vi "Generate NIPKG List from Installed Packages.vi"() -> ()   [LabVIEW 2017]
doc: "GUI tool for selecting NI PKG dependencies from the list of installed NI Packages. Allows selected package list to be exported to a file for use with the SBOM tools."
uses:
  <vilib>/National Instruments/NIPM API (Beta)/_support/package attributes.ctl
  ead8c88d-cf43-4405-a832-7fe61a0fbdd3.vi
  <vilib>/JDP Science/JSONtext/Variant to JSON Text.vi
  <userlib>/_OpenG.lib/array/array.llb/Delete Elements from 1D Array (Variant)__ogtk.vi
  <vilib>/National Instruments/NIPM API (Beta)/NIPM_API.lvlib
panel:
  in  "Export":bool
  in  "System Refresh Button":bool
  in  "System Stop Button":bool
  out "Package Info Progress":dbl(slide) scale=0.0..1.0
  in  "Add":bool
  in  "Remove":bool
  in  "Selected Packages":i32[](listbox)
  out "Current Package":T1={"Package Name"="", "Display name"="", "Version"="", "Display version"="", "Synopsis"="", "Description"="", "Maintainer"="", "Maintainer email address"="", "Category"="", "Homepage"="", "Release notes"="", "Depends"=[], "Recommends"=[], "Suggests"=[], "Conflicts"=[], "Provides"=[], "Replaces"=[], "Supplements"=[], "Enhances"=[], "Product"=FALSE, "User visible"=FALSE, "Installed size (KB)"=0, "Package filesize (bytes)"=0, "Architecture"="", "Agent"="file", "MD5Checksum"=""}
  in  "Installed NI Packages":i32[](listbox)
  # "NI Package Dependency Selector"
  # "Use this tool to generate a list of NI Package dependencies for a Software Bill-of-Materials."
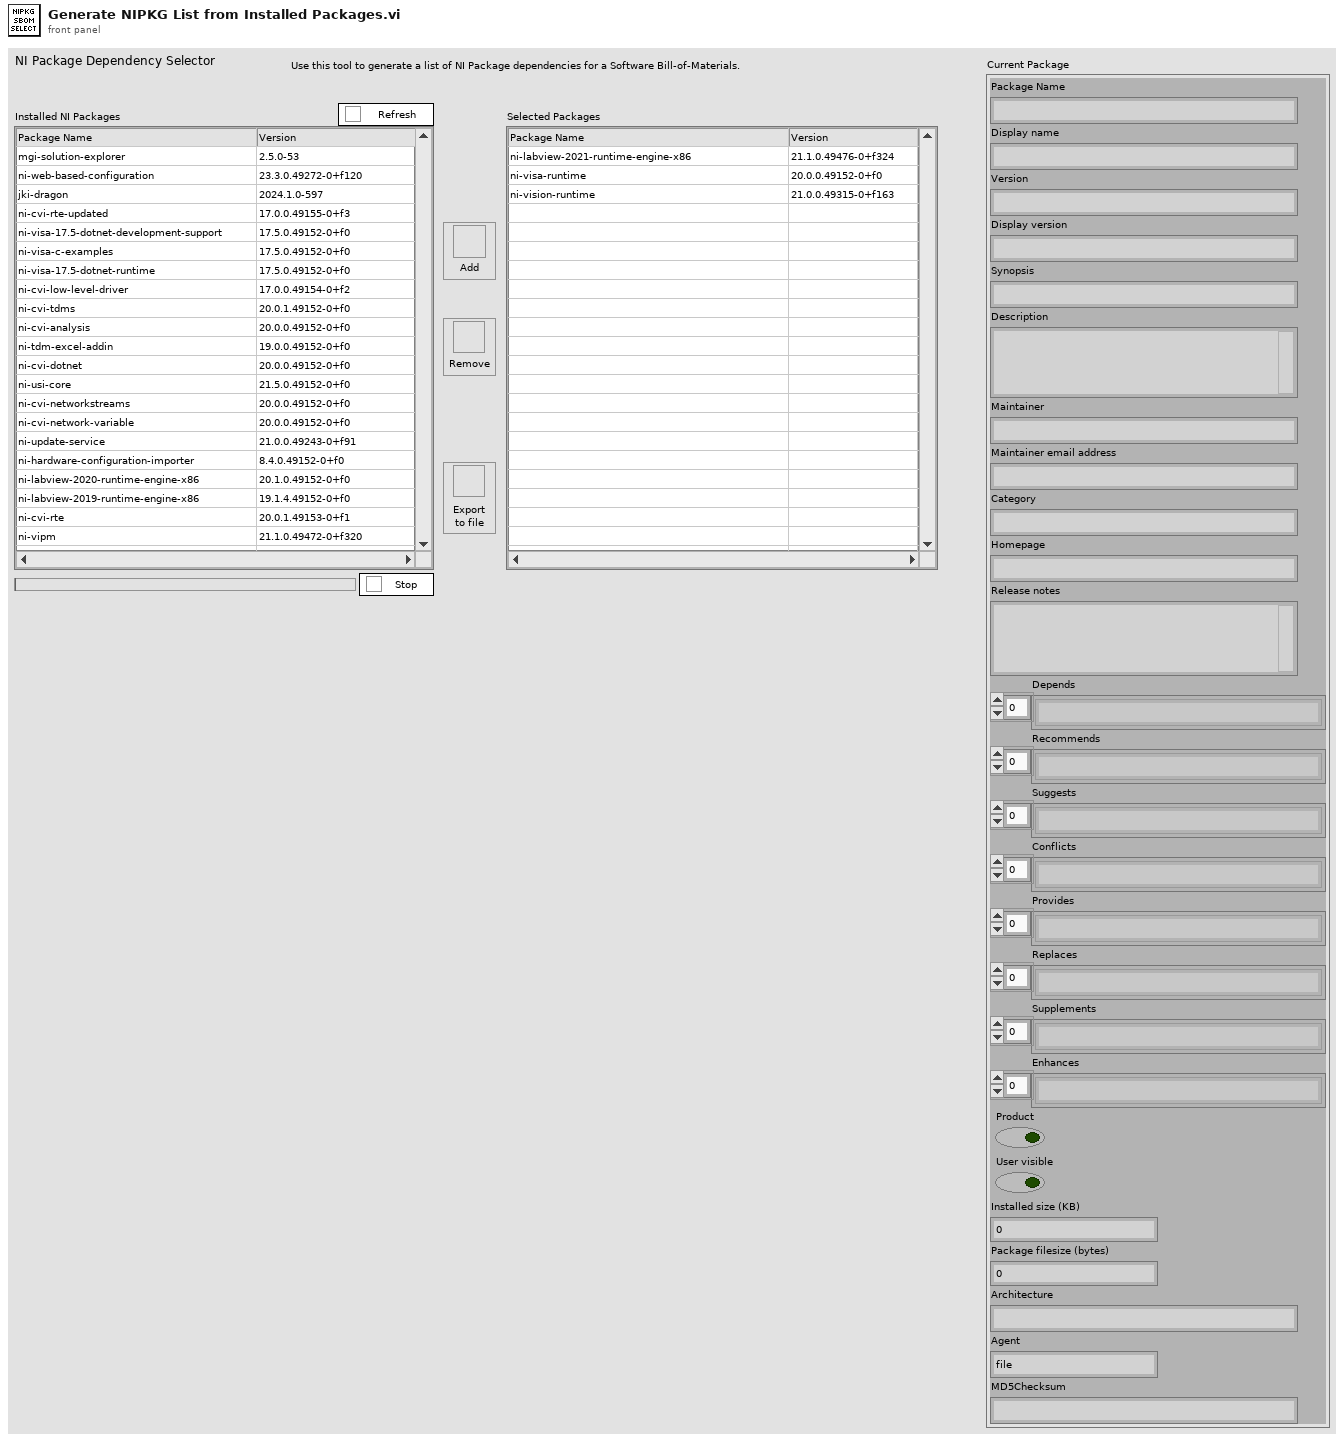
[diagram p1: front panel]
types:
  T1 = typedef "NIPM_API.lvlib/package attributes.ctl" = cluster{"Package Name":string, "Display name":string, "Version":string, "Display version":string, "Synopsis":string, "Description":string, "Maintainer":string, "Maintainer email address":string, "Category":string, "Homepage":string, "Release notes":string, "Depends":string[], "Recommends":string[], "Suggests":string[], "Conflicts":string[], "Provides":string[], "Replaces":string[], "Supplements":string[], "Enhances":string[], "Product":bool, "User visible":bool, "Installed size (KB)":u64, "Package filesize (bytes)":u64, "Architecture":string, "Agent":string, "MD5Checksum":string}
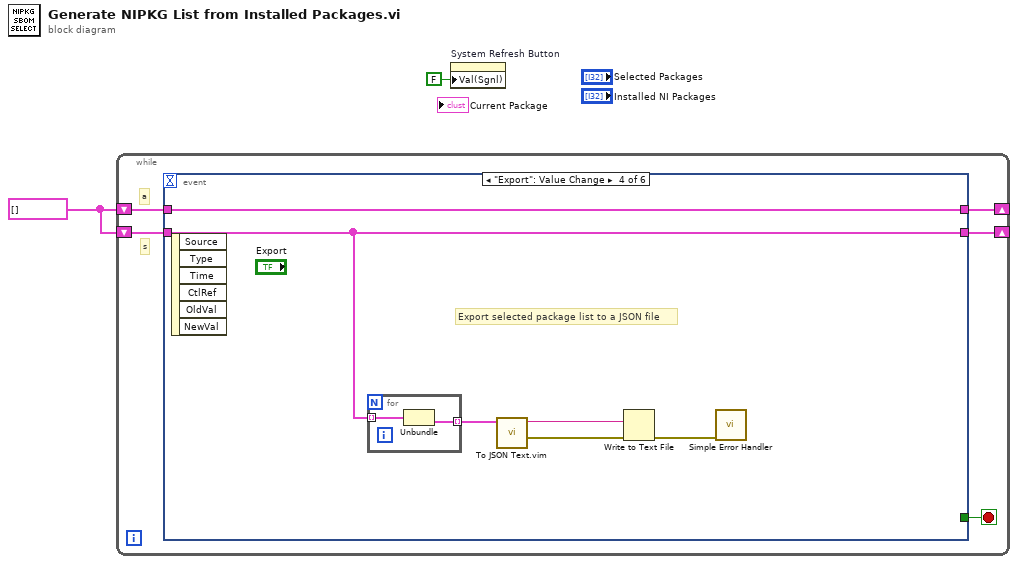
[diagram p0: block diagram]
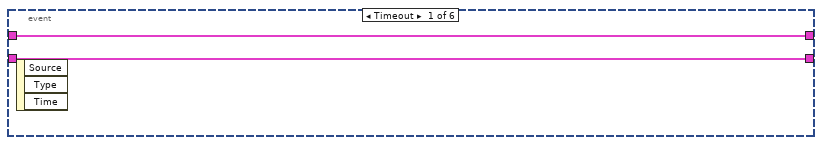
[diagram p2: hidden frame]
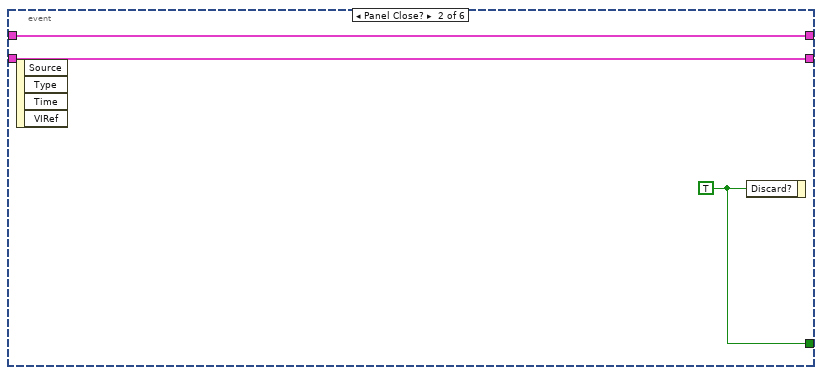
[diagram p3: hidden frame]
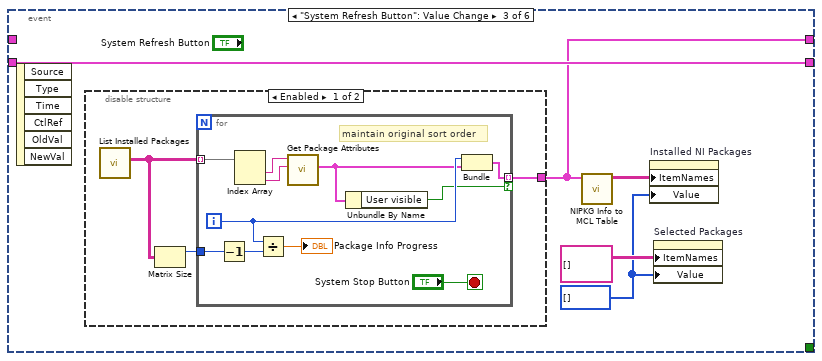
[diagram p4: hidden frame]
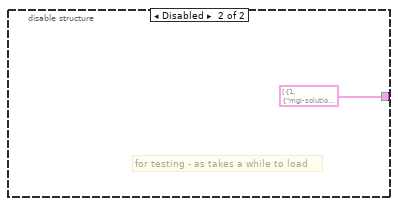
[diagram p5: hidden frame]
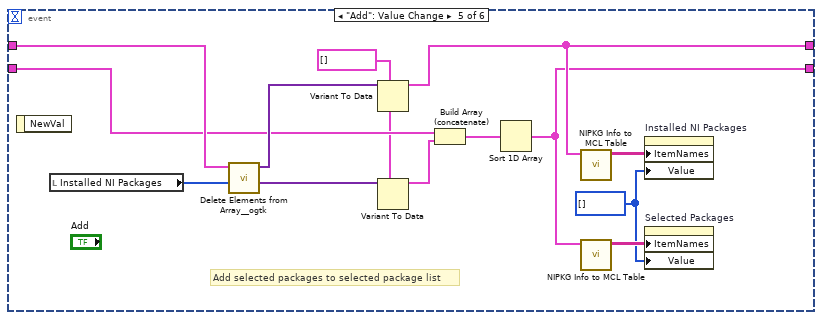
[diagram p6: hidden frame]
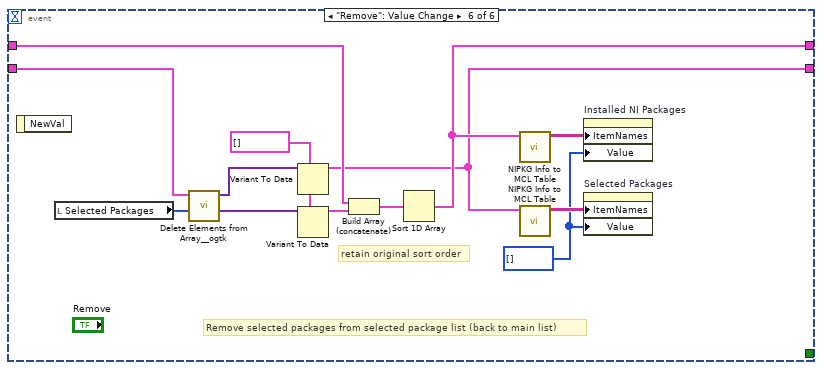
[diagram p7: hidden frame]
diagram:
  w1 = cluster{i32, "package attributes":T1}[] []
  n1 = while {
    shift-right: [w6] -> _
    shift-left: w1 -> [w5]
    shift-right: [w4] -> _
    shift-left: w1 -> [w3]
    stop <- w7 stop-if-true
    # "s"
    # "a"
    n2 = event shown="[3] \"Export\": Value Change" {
      selector: _ -> [_ _ _ _ _ _]
      dyn-events: _ -> [_ _ _ _ _ _]
      timeout: _ -> [_ _ _ _ _ _]
      tunnel: [_ w12 _ _ _ _] -> w7
      tunnel: [w9 w11 w14 w38 w43 w57] -> w6
      tunnel: w5 -> [w9 w11 _ w38 w53 w60]
      tunnel: [w8 w10 w17 w34 w42 w56] -> w4
      tunnel: w3 -> [w8 w10 w17 w34 w49 w63]
      event Timeout {
        n3 = event-data() -> ()  [unwired: 1 in, 3 out]
      }
      event Panel Close? {
        w12 = TRUE ("Discard?")
        n4 = event-data() -> ()  [unwired: 1 in, 4 out]
        n5 = event-data("Discard?"=w12) -> ()  [unwired: 1 in, 1 out]
      }
      event "System Refresh Button": Value Change {
        w13 = i32[] [] ("Installed NI Packages")
        n6 = event-data() -> ()  [unwired: 1 in, 6 out]
        n7 = disable-structure shown="Enabled" {
          disable-tunnel: [w18 cluster{i32, "package attributes":T1}[] [{1, "package attributes"={"Package Name"="mgi-solution-explorer", "Display name"="MGI Solution Explorer", "Version"="2.5.0-53", "Display version"="", "Synopsis"="Easily develop and build multi-project based LabVIEW Applications", "Description"="", "Maintainer"="Moore Good Ideas Inc", "Maintainer email address"="support@mooregoodideas.com", "Category"="Application Software", "Homepage"="http://www.mooregoodideas.com/products/solution-explorer/", "Release notes"="New supported features:\n\n* Added support for RT Packages and Exe\n\n* Added support for French, German, Japanese, Korean, and Chinese versions of LabVIEW (previously, some builds would fail in these environments due to differences in the build spec)\n\n.\n\nThe following reported bugs have all been fixed:\n\n* Unable to explore to destination when build spec destination is absolute (and other problems related to relative/absolute paths).\n\n* The version number saved in the lvsln file is not populated in the UI when the lvsoln is loaded from solution explorer vs double clicking a lvsln file on disk\n\n* Sub-Solutions always build as debug when using right-click shortcut to \"Rebuild\"", "Depends"=["ni-labview-2019-runtime-engine-x86"], "Recommends"=[], "Suggests"=[], "Conflicts"=[], "Provides"=["mgi-solution-explorer (= 2.5.0-53)"], "Replaces"=[], "Supplements"=[], "Enhances"=[], "Product"=TRUE, "User visible"=TRUE, "Installed size (KB)"=10798, "Package filesize (bytes)"=10207864, "Architecture"="windows_all", "Agent"="file", "MD5Checksum"=""}}, {7, "package attributes"={"Package Name"="ni-web-based-configuration", "Display name"="NI Web-Based Configuration and Monitoring", "Version"="23.3.0.49272-0+f120", "Display version"="2023 Q2", "Synopsis"="Enables remote configuration of the system from a web browser.", "Description"="Use NI Web-Based Configuration and Monitoring to configure and monitor NI web servers from a web browser.", "Maintainer"="National Instruments", "Maintainer email address"="support@ni.com", "Category"="Utilities", "Homepage"="https://www.ni.com", "Release notes"="", "Depends"=["ni-sysapi-webservice (>= 23.3.0)", "ni-system-webserver (>= 23.1.0)", "ni-wif-landingpage (>= 23.3.0)"], "Recommends"=[], "Suggests"=[], "Conflicts"=[], "Provides"=["ni-web-based-configuration (= 23.3.0.49272-0+f120)"], "Replaces"=[], "Supplements"=[], "Enhances"=[], "Product"=FALSE, "User visible"=TRUE, "Installed size (KB)"=0, "Package filesize (bytes)"=6390334, "Architecture"="windows_x64", "Agent"="file", "MD5Checksum"=""}}, {8, "package attributes"={"Package Name"="jki-dragon", "Display name"="JKI Dragon", "Version"="2024.1.0-597", "Display version"="2024 Q1", "Synopsis"="Manage package dependencies directly from your LabVIEW project. Works with VIPM and NI Package Manager to provide a complete dependency management solution for LabVIEW Add-ons, NI Software and Drivers, and more.", "Description"="", "Maintainer"="JKI", "Maintainer email address"="info@jki.net", "Category"="Application Software", "Homepage"="dragon.vipm.io", "Release notes"="", "Depends"=["ni-labview-command-line-interface-x86 (>= 23.1.0)", "ni-labview-2024-runtime-engine (>= 24.1.0)", "ni-certificates (>= 21.5.0)"], "Recommends"=["ni-certificates"], "Suggests"=[], "Conflicts"=[], "Provides"=["jki-dragon (= 2024.1.0-597)"], "Replaces"=[], "Supplements"=[], "Enhances"=[], "Product"=TRUE, "User visible"=TRUE, "Installed size (KB)"=6707, "Package filesize (bytes)"=30773408, "Architecture"="windows_x64", "Agent"="file", "MD5Checksum"=""}}, {13, "package attributes"={"Package Name"="ni-cvi-rte-updated", "Display name"="LabWindows/CVI Shared Runtime 2017 Merge Module Redeployment Support", "Version"="17.0.0.49155-0+f3", "Display version"="17.0.0", "Synopsis"="The LabWindows/CVI Shared Runtime 2017 Merge Module Redeployment Support contains the LabWindows/CVI support files necessary to deploy the LabWindows/CVI Runtime through merge modules to a target computer on which you want to run executables or use DLLs created with LabWindows/CVI.", "Description"="", "Maintainer"="National Instruments", "Maintainer email address"="support@ni.com", "Category"="Runtime", "Homepage"="http://www.ni.com", "Release notes"="", "Depends"=["ni-mdfsupport (>=17.0.0)", " ni-metauninstaller (>=17.0.0)", ""], "Recommends"=[], "Suggests"=[], "Conflicts"=["c6f76062-cdcb-4931-8580-012af2152602 (<<17.0.0)", ""], "Provides"=["c6f76062-cdcb-4931-8580-012af2152602 (=17.00.49155)", ""], "Replaces"=["c6f76062-cdcb-4931-8580-012af2152602 (<<17.0.0)", ""], "Supplements"=[], "Enhances"=[], "Product"=FALSE, "User visible"=TRUE, "Installed size (KB)"=0, "Package filesize (bytes)"=0, "Architecture"="windows_x64", "Agent"="wininst", "MD5Checksum"=""}}, {15, "package attributes"={"Package Name"="ni-visa-17.5-dotnet-development-support", "Display name"="NI-VISA .NET Development Support 17.5", "Version"="17.5.0.49152-0+f0", "Display version"="17.5.0", "Synopsis"="Installs the local assembly for development of NI-VISA applications using the standard .NET API specified by the IVI Foundation.", "Description"="", "Maintainer"="National Instruments", "Maintainer email address"="support@ni.com", "Category"="Drivers", "Homepage"="http://www.ni.com", "Release notes"="", "Depends"=["ni-help-assistant (>=2.1.0)", " ni-launcher (>=17.0.0)", " ni-mdfsupport (>=17.5.0)", " ni-metauninstaller (>=17.5.0)", " ni-msiproperties (>=17.5.0)", " ni-visa-17.5-dotnet-runtime (>=17.5.0)", " ni-visa-documentation (>=17.5.0)", ""], "Recommends"=[], "Suggests"=[], "Conflicts"=[], "Provides"=["ae0a052f-25d6-457c-8ef3-5a630d3852c5 (=17.50.49152)", " ec7cccdd-f896-4ef7-9679-bd24d9a0c5c3 (=17.50.49152)", ""], "Replaces"=[], "Supplements"=[], "Enhances"=[], "Product"=FALSE, "User visible"=TRUE, "Installed size (KB)"=0, "Package filesize (bytes)"=0, "Architecture"="windows_x64", "Agent"="wininst", "MD5Checksum"=""}}, {17, "package attributes"={"Package Name"="ni-visa-c-examples", "Display name"="NI-VISA C Examples", "Version"="17.5.0.49152-0+f0", "Display version"="17.5.0", "Synopsis"="NI-VISA examples for programming using the C API.", "Description"="", "Maintainer"="National Instruments", "Maintainer email address"="support@ni.com", "Category"="Drivers", "Homepage"="http://www.ni.com", "Release notes"="", "Depends"=["ni-launcher (>=17.0.0)", " ni-mdfsupport (>=17.5.0)", " ni-metauninstaller (>=17.5.0)", " ni-visa-development-support-compatibility (>=17.5.0)", ""], "Recommends"=[], "Suggests"=[], "Conflicts"=["e72d936f-f240-4f4b-90c4-a49999c2b116 (<<17.0.0)", ""], "Provides"=["e72d936f-f240-4f4b-90c4-a49999c2b116 (=17.50.49152)", ""], "Replaces"=["e72d936f-f240-4f4b-90c4-a49999c2b116 (<<17.0.0)", ""], "Supplements"=[], "Enhances"=[], "Product"=FALSE, "User visible"=TRUE, "Installed size (KB)"=0, "Package filesize (bytes)"=0, "Architecture"="windows_x64", "Agent"="wininst", "MD5Checksum"=""}}, {25, "package attributes"={"Package Name"="ni-visa-17.5-dotnet-runtime", "Display name"="NI-VISA .NET Runtime 17.5", "Version"="17.5.0.49152-0+f0", "Display version"="17.5.0", "Synopsis"="Enables you to run applications that use the NI-VISA .NET API.", "Description"="", "Maintainer"="National Instruments", "Maintainer email address"="support@ni.com", "Category"="Drivers", "Homepage"="http://www.ni.com", "Release notes"="", "Depends"=["ni-mdfsupport (>=17.5.0)", " ni-metauninstaller (>=17.5.0)", " ni-msiproperties (>=17.5.0)", " ni-mstudio-common-fx40-runtime (>=17.0.0)", " ni-visa-dotnet-shared-components-5.8 (>=5.8.1)", " ni-visa-runtime (>=17.5.0)", ""], "Recommends"=[], "Suggests"=[], "Conflicts"=[], "Provides"=["33687859-dc67-437f-a652-689b14a1c74c (=17.50.49152)", ""], "Replaces"=[], "Supplements"=[], "Enhances"=[], "Product"=FALSE, "User visible"=TRUE, "Installed size (KB)"=0, "Package filesize (bytes)"=0, "Architecture"="windows_x64", "Agent"="wininst", "MD5Checksum"=""}}, {36, "package attributes"={"Package Name"="ni-cvi-low-level-driver", "Display name"="LabWindows/CVI Low-Level Driver", "Version"="17.0.0.49154-0+f2", "Display version"="17.0.0", "Synopsis"="The NI LabWindows/CVI Low-Level Driver provides Port I/O functions.", "Description"="", "Maintainer"="National Instruments", "Maintainer email address"="support@ni.com", "Category"="Runtime", "Homepage"="http://www.ni.com", "Release notes"="", "Depends"=["ni-mdfsupport (>=17.0.0)", " ni-metauninstaller (>=17.0.0)", ""], "Recommends"=[], "Suggests"=[], "Conflicts"=["20931852-6aa9-4918-926b-130d07a4cf8b (<<15.5.0)", ""], "Provides"=["20931852-6aa9-4918-926b-130d07a4cf8b (=17.00.49154)", " f8d3f894-f912-4a7e-9318-0c547d37d033 (=17.00.49154)", ""], "Replaces"=["20931852-6aa9-4918-926b-130d07a4cf8b (<<15.5.0)", ""], "Supplements"=[], "Enhances"=[], "Product"=FALSE, "User visible"=TRUE, "Installed size (KB)"=0, "Package filesize (bytes)"=0, "Architecture"="windows_x64", "Agent"="wininst", "MD5Checksum"=""}}, {80, "package attributes"={"Package Name"="ni-cvi-tdms", "Display name"="LabWindows/CVI TDM Streaming Library Runtime", "Version"="20.0.1.49152-0+f0", "Display version"="2020 f1", "Synopsis"="The LabWindows/CVI TDM Streaming Library Runtime contains functions that you can use to log large amounts of test data quickly.", "Description"="", "Maintainer"="National Instruments", "Maintainer email address"="support@ni.com", "Category"="Runtime", "Homepage"="http://www.ni.com", "Release notes"="", "Depends"=["ni-mdfsupport (>= 20.0.0)", "ni-metauninstaller (>= 20.0.0)", "ni-tdms (>= 19.0.0)"], "Recommends"=[], "Suggests"=[], "Conflicts"=["5a8af88d-486d-4e30-a7a5-8d8a039bbebf (< 15.5.0)"], "Provides"=["5a8af88d-486d-4e30-a7a5-8d8a039bbebf (= 20.01.49152)", "d14439a1-ce0e-49de-9bed-1d89c532f9e4 (= 20.01.49152)", "ni-cvi-tdms (= 20.0.1.49152-0+f0)"], "Replaces"=["5a8af88d-486d-4e30-a7a5-8d8a039bbebf (< 15.5.0)"], "Supplements"=[], "Enhances"=[], "Product"=FALSE, "User visible"=TRUE, "Installed size (KB)"=0, "Package filesize (bytes)"=1050210, "Architecture"="windows_all", "Agent"="wininst", "MD5Checksum"=""}}, {81, "package attributes"={"Package Name"="ni-cvi-analysis", "Display name"="LabWindows/CVI Analysis Library Runtime", "Version"="20.0.0.49152-0+f0", "Display version"="2020", "Synopsis"="The LabWindows/CVI Analysis Library Runtime provides functions for 1D and 2D array manipulation, complex operations, matrix operations, and statistics.", "Description"="", "Maintainer"="National Instruments", "Maintainer email address"="support@ni.com", "Category"="Runtime", "Homepage"="http://www.ni.com", "Release notes"="", "Depends"=["ni-mdfsupport (>= 20.0.0)", "ni-metauninstaller (>= 20.0.0)", "ni-mkl-2020 (>= 20.0.0)"], "Recommends"=[], "Suggests"=[], "Conflicts"=["86208b51-159e-4f6f-9c62-0d5efc9324d8 (< 15.5.0)"], "Provides"=["6a61602b-c99a-49c8-a607-7fadd5124218 (= 20.00.49152)", "86208b51-159e-4f6f-9c62-0d5efc9324d8 (= 20.00.49152)", "ni-cvi-analysis (= 20.0.0.49152-0+f0)"], "Replaces"=["86208b51-159e-4f6f-9c62-0d5efc9324d8 (< 15.5.0)"], "Supplements"=[], "Enhances"=[], "Product"=FALSE, "User visible"=TRUE, "Installed size (KB)"=0, "Package filesize (bytes)"=1962742, "Architecture"="windows_all", "Agent"="wininst", "MD5Checksum"=""}}, {96, "package attributes"={"Package Name"="ni-tdm-excel-addin", "Display name"="TDM Excel Add-In", "Version"="19.0.0.49152-0+f0", "Display version"="19.0.0", "Synopsis"="Extends the capabilities of Microsoft Excel by adding the ability to load TDM or TDMS files written with NI hardware and application software.", "Description"="", "Maintainer"="National Instruments", "Maintainer email address"="support@ni.com", "Category"="Add-Ons", "Homepage"="http://www.ni.com", "Release notes"="", "Depends"=["ni-mdfsupport (>= 19.0.0)", "ni-metauninstaller (>= 19.0.0)", "ni-msvcrt-2015 (>= 14.1.5)"], "Recommends"=[], "Suggests"=[], "Conflicts"=["6d2ebdaf-6ccd-44f3-b767-4df9e0f2037b (< 15.1.0)"], "Provides"=["6d2ebdaf-6ccd-44f3-b767-4df9e0f2037b (= 19.00.49152)", "e19027c7-041a-ec1d-35b0-601b42088734 (= 19.00.49152)", "ni-tdm-excel-addin (= 19.0.0.49152-0+f0)"], "Replaces"=["6d2ebdaf-6ccd-44f3-b767-4df9e0f2037b (< 15.1.0)"], "Supplements"=[], "Enhances"=[], "Product"=FALSE, "User visible"=TRUE, "Installed size (KB)"=0, "Package filesize (bytes)"=17330464, "Architecture"="windows_all", "Agent"="wininst", "MD5Checksum"=""}}, {100, "package attributes"={"Package Name"="ni-cvi-dotnet", "Display name"="LabWindows/CVI .NET Library Runtime", "Version"="20.0.0.49152-0+f0", "Display version"="2020", "Synopsis"="The LabWindows/CVI .NET Library Runtime provides functions that facilitate calling .NET assemblies.", "Description"="", "Maintainer"="National Instruments", "Maintainer email address"="support@ni.com", "Category"="Runtime", "Homepage"="http://www.ni.com", "Release notes"="", "Depends"=["ni-cvi-2020-reflector (>= 20.0.0)", "ni-mdfsupport (>= 20.0.0)", "ni-metauninstaller (>= 20.0.0)", "ni-msvcrt-2015 (>= 14.1.5)"], "Recommends"=[], "Suggests"=[], "Conflicts"=["0ddb211a-941b-4125-9518-e81e10409f2e (< 15.5.0)"], "Provides"=["0ddb211a-941b-4125-9518-e81e10409f2e (= 20.00.49152)", "dea0ff7b-e7f3-45a4-80ea-cd21aad8b94e (= 20.00.49152)", "ni-cvi-dotnet (= 20.0.0.49152-0+f0)"], "Replaces"=["0ddb211a-941b-4125-9518-e81e10409f2e (< 15.5.0)"], "Supplements"=[], "Enhances"=[], "Product"=FALSE, "User visible"=TRUE, "Installed size (KB)"=0, "Package filesize (bytes)"=912820, "Architecture"="windows_all", "Agent"="wininst", "MD5Checksum"=""}}, {101, "package attributes"={"Package Name"="ni-usi-core", "Display name"="NI USI Core", "Version"="21.5.0.49152-0+f0", "Display version"="21.5.0", "Synopsis"="NI USI Core provides components for NI TDM software", "Description"="NI USI Core provides components for NI TDM software and allows access to any file format using DataPlugins.", "Maintainer"="National Instruments", "Maintainer email address"="support@ni.com", "Category"="Runtime", "Homepage"="https://www.ni.com", "Release notes"="", "Depends"=["ni-datafinder-desktop-quit-dc (>= 21.5.0)", "ni-dataplugins-python-host (>= 21.5.0)", "ni-mdfsupport (>= 20.7.0)", "ni-metauninstaller (>= 20.7.0)", "ni-msdotnet4x (>= 4.6.3)", "ni-msiproperties (>= 20.7.0)", "ni-msvcrt-2015 (>= 14.1.5)", "ni-tdms (>= 21.0.0)"], "Recommends"=[], "Suggests"=[], "Conflicts"=["10ccb544-327e-4681-a225-457c5c9a44a2 (< 18.00.0)"], "Provides"=["10ccb544-327e-4681-a225-457c5c9a44a2 (= 21.50.49152)", "61d0eb5a-10f6-49d6-afbc-83224e99263d (= 21.50.49152)", "ni-usi-core (= 21.5.0.49152-0+f0)"], "Replaces"=["10ccb544-327e-4681-a225-457c5c9a44a2 (< 18.00.0)"], "Supplements"=[], "Enhances"=[], "Product"=FALSE, "User visible"=TRUE, "Installed size (KB)"=0, "Package filesize (bytes)"=36049368, "Architecture"="windows_all", "Agent"="wininst", "MD5Checksum"=""}}, {109, "package attributes"={"Package Name"="ni-cvi-networkstreams", "Display name"="LabWindows/CVI Network Streams Library Runtime", "Version"="20.0.0.49152-0+f0", "Display version"="2020", "Synopsis"="The LabWindows/CVI Network Streams Library Runtime provides functions for reading and writing data to network streams. You also can use the Network Streams Library functions in real-time (RT) applications.", "Description"="", "Maintainer"="National Instruments", "Maintainer email address"="support@ni.com", "Category"="Runtime", "Homepage"="http://www.ni.com", "Release notes"="", "Depends"=["ni-logos (>= 20.0.0)", "ni-mdfsupport (>= 20.0.0)", "ni-metauninstaller (>= 20.0.0)", "ni-msvcrt-2015 (>= 14.1.5)"], "Recommends"=[], "Suggests"=[], "Conflicts"=["40a5ad7f-4baf-4a5c-8b56-426b84f75c05 (< 15.5.0)"], "Provides"=["1ab6d8ff-2c26-4bc0-b35b-afc94d6b0f0b (= 20.00.49152)", "40a5ad7f-4baf-4a5c-8b56-426b84f75c05 (= 20.00.49152)", "ni-cvi-networkstreams (= 20.0.0.49152-0+f0)"], "Replaces"=["40a5ad7f-4baf-4a5c-8b56-426b84f75c05 (< 15.5.0)"], "Supplements"=[], "Enhances"=[], "Product"=FALSE, "User visible"=TRUE, "Installed size (KB)"=0, "Package filesize (bytes)"=1353240, "Architecture"="windows_all", "Agent"="wininst", "MD5Checksum"=""}}, {110, "package attributes"={"Package Name"="ni-cvi-network-variable", "Display name"="LabWindows/CVI Network Variable Library Runtime", "Version"="20.0.0.49152-0+f0", "Display version"="2020", "Synopsis"="The LabWindows/CVI Network Variable Library Runtime provides functions for reading and writing data to network variables. You can use the functions in this library to communicate with LabVIEW shared variables and Measurement Studio network variables. You also can use the Network Variable Library functions in real-time (RT) applications.", "Description"="", "Maintainer"="National Instruments", "Maintainer email address"="support@ni.com", "Category"="Runtime", "Homepage"="http://www.ni.com", "Release notes"="", "Depends"=["ni-logos (>= 20.0.0)", "ni-mdfsupport (>= 20.0.0)", "ni-metauninstaller (>= 20.0.0)"], "Recommends"=[], "Suggests"=[], "Conflicts"=["15ce39fe-1354-484d-b8ca-459077449fb3 (< 15.5.0)"], "Provides"=["15ce39fe-1354-484d-b8ca-459077449fb3 (= 20.00.49152)", "f31a3240-633d-4040-ac85-0168d0f48b5f (= 20.00.49152)", "ni-cvi-network-variable (= 20.0.0.49152-0+f0)"], "Replaces"=["15ce39fe-1354-484d-b8ca-459077449fb3 (< 15.5.0)"], "Supplements"=[], "Enhances"=[], "Product"=FALSE, "User visible"=TRUE, "Installed size (KB)"=0, "Package filesize (bytes)"=1321840, "Architecture"="windows_all", "Agent"="wininst", "MD5Checksum"=""}}, {112, "package attributes"={"Package Name"="ni-update-service", "Display name"="NI Update Service", "Version"="21.0.0.49243-0+f91", "Display version"="21.0.0", "Synopsis"="NI Update Service checks for and electronically delivers software updates for NI software and drivers.", "Description"="", "Maintainer"="National Instruments", "Maintainer email address"="support@ni.com", "Category"="Utilities", "Homepage"="https://www.ni.com", "Release notes"="IMPROVEMENTS - Added support for NI Package Manager and package updates on 32-bit Windows OSes. - No longer holds installation mutex when UI is showing so that now you can install packages from NI Package Manager while Update Service is open. - When an update is selected, included package updates are automatically selected.\n\nRefer to the NI website at https://www.ni.com/r/zr1xoo for more information regarding known issues, compatibility, and important notices for Update Service.", "Depends"=["ni-euladepot (>= 21.0.0)", "ni-help-assistant (>= 2.2.0)", "ni-mdfsupport (>= 21.0.0)", "ni-metasuite (>= 21.0.0)", "ni-metauninstaller (>= 21.0.0)", "ni-msdotnet4x (>= 4.6.3)", "ni-msiproperties (>= 21.0.0)", "ni-msvcrt-2015 (>= 14.1.5)"], "Recommends"=[], "Suggests"=[], "Conflicts"=["11d580a9-caa9-4fae-acce-008751a7ae9f (< 16.1)"], "Provides"=["11d580a9-caa9-4fae-acce-008751a7ae9f (= 21.00.49243)", "a3b0165f-4500-4a92-b134-27f1a7dd5732 (= 21.00.49243)", "e14c752c-9307-4a71-b65e-e7b9ce0d063c (= 21.00.49243)", "ni-update-service (= 21.0.0.49243-0+f91)"], "Replaces"=["11d580a9-caa9-4fae-acce-008751a7ae9f (< 16.1)"], "Supplements"=[], "Enhances"=[], "Product"=TRUE, "User visible"=TRUE, "Installed size (KB)"=0, "Package filesize (bytes)"=28661130, "Architecture"="windows_x64", "Agent"="wininst", "MD5Checksum"=""}}, {123, "package attributes"={"Package Name"="ni-hardware-configuration-importer", "Display name"="NI Hardware Configuration Importer", "Version"="8.4.0.49152-0+f0", "Display version"="5.1.0", "Synopsis"="Program for importing NI hardware configurations.", "Description"="", "Maintainer"="National Instruments", "Maintainer email address"="support@ni.com", "Category"="Utilities", "Homepage"="https://www.ni.com", "Release notes"="", "Depends"=["ni-mdfsupport (>= 20.6.0)", "ni-metauninstaller (>= 20.6.0)", "ni-mstudio-common-fx40-19.0.0-runtime (>= 19.0.0)", "ni-portable-configuration (>= 19.5.0)", "ni-sysapi (>= 20.0.0)"], "Recommends"=[], "Suggests"=[], "Conflicts"=["b8ac606b-a9af-403c-9009-a8f27288faf1 (< 0.0.1)"], "Provides"=["b8ac606b-a9af-403c-9009-a8f27288faf1 (= 8.40.49152)", "ni-hardware-configuration-importer (= 8.4.0.49152-0+f0)"], "Replaces"=["b8ac606b-a9af-403c-9009-a8f27288faf1 (< 0.0.1)"], "Supplements"=[], "Enhances"=[], "Product"=FALSE, "User visible"=TRUE, "Installed size (KB)"=0, "Package filesize (bytes)"=16600588, "Architecture"="windows_x64", "Agent"="wininst", "MD5Checksum"=""}}, {124, "package attributes"={"Package Name"="ni-labview-2020-runtime-engine-x86", "Display name"="LabVIEW Runtime (32-bit)", "Version"="20.1.0.49152-0+f0", "Display version"="2020 SP1", "Synopsis"="The LabVIEW Runtime is a software add-on that enables engineers to run executables on a nondevelopment machine.", "Description"="The LabVIEW Runtime enables you to run executables created with the LabVIEW Application Builder on machines that do not have LabVIEW installed. The LabVIEW Runtime includes the libraries and other files necessary to run basic application types built in LabVIEW.", "Maintainer"="National Instruments", "Maintainer email address"="support@ni.com", "Category"="Programming Environments", "Homepage"="https://www.ni.com", "Release notes"="Refer to the NI website at https://www.ni.com/r/lv2020x1rm for installation instructions, known issues, bug fixes, compatibility information, and other important notices about this product.", "Depends"=["ni-activex-container (>= 17.1.2)", "ni-curl (>= 20.5.0)", "ni-deployment-framework-x86 (>= 20.0.0)", "ni-error-report-x86 (>= 20.1.0)", "ni-error-reporting-interface (>= 20.1.0)", "ni-labview-2020-realtime-nbfifo-x86 (>= 20.0.0)", "ni-labview-2020-runtime-engine-resource (>= 20.1.0)", "ni-logos (>= 20.0.0)", "ni-lv-web-server-labview-2020-runtime-engine-x86-support (>= 20.5.1)", "ni-mdfsupport (>= 20.6.0)", "ni-mdnsresponder (>= 19.0.0)", "ni-metauninstaller (>= 20.6.0)", "ni-mkl-2017 (>= 17.0.1)", "ni-mkl-2020 (>= 20.0.0)", "ni-msiproperties (>= 20.6.0)", "ni-mstudio-cw3dgraph (>= 8.7.5)", "ni-msvcrt-2015 (>= 14.1.5)", "ni-python-interface (>= 20.0.0)", "ni-svcloc (>= 20.0.0)", "ni-systemlogging-utils (>= 20.0.0)", "ni-tdms (>= 19.0.0)", "ni-traceengine (>= 20.0.0)"], "Recommends"=[], "Suggests"=[], "Conflicts"=[], "Provides"=["6394b505-4b86-41e5-affb-f6f12e05046c (= 20.10.49152)", "d84fc73f-d1e0-4c05-a30c-db882cd1abd8 (= 20.10.49152)", "ni-labview-2020-runtime-engine-x86 (= 20.1.0.49152-0+f0)"], "Replaces"=[], "Supplements"=[], "Enhances"=[], "Product"=TRUE, "User visible"=TRUE, "Installed size (KB)"=0, "Package filesize (bytes)"=27713636, "Architecture"="windows_all", "Agent"="wininst", "MD5Checksum"=""}}, {125, "package attributes"={"Package Name"="ni-labview-2019-runtime-engine-x86", "Display name"="LabVIEW Runtime (32-bit)", "Version"="19.1.4.49152-0+f0", "Display version"="2019 SP1 f4", "Synopsis"="The LabVIEW Runtime is a software add-on that enables engineers to run executables on a nondevelopment machine.", "Description"="The LabVIEW Runtime enables you to run executables created with the LabVIEW Application Builder on machines that do not have LabVIEW installed. The LabVIEW Runtime includes the libraries and other files necessary to run basic application types built in LabVIEW.", "Maintainer"="National Instruments", "Maintainer email address"="support@ni.com", "Category"="Programming Environments", "Homepage"="http://www.ni.com", "Release notes"="Refer to the NI website at http://www.ni.com/r/lv2019sp1rm for installation instructions, known issues, bug fixes, compatibility information, and other important notices about this product.", "Depends"=["ni-activex-container (>= 17.1.1)", "ni-curl (>= 20.5.0)", "ni-deployment-framework-x86 (>= 19.0.0)", "ni-error-report-x86 (>= 19.0.0)", "ni-error-reporting-interface (>= 19.0.0)", "ni-labview-2019-realtime-nbfifo-x86 (>= 19.0.0)", "ni-labview-2019-runtime-engine-resource (>= 19.1.0)", "ni-logos (>= 19.0.0)", "ni-lv-web-server-labview-2019-runtime-engine-x86-support (>= 19.0.0)", "ni-mdfsupport (>= 19.0.0)", "ni-mdnsresponder (>= 19.0.0)", "ni-metauninstaller (>= 19.0.0)", "ni-mkl-2017 (>= 17.0.1)", "ni-mkl-2018 (>= 18.0.1)", "ni-msiproperties (>= 19.0.0)", "ni-mstudio-cw3dgraph (>= 8.7.5)", "ni-msvcrt-2015 (>= 14.1.5)", "ni-python-interface (>= 19.0.0)", "ni-svcloc (>= 19.0.0)", "ni-systemlogging-utils (>= 19.0.0)", "ni-tdms (>= 19.0.0)", "ni-traceengine (>= 19.0.0)"], "Recommends"=[], "Suggests"=[], "Conflicts"=[], "Provides"=["76adfbe4-105e-4341-a6fb-36b5aefea0c7 (= 19.14.49152)", "7d6295e5-8fb8-4bce-b1cd-b5b396fa1d3f (= 19.14.49152)", "ni-labview-2019-runtime-engine-x86 (= 19.1.4.49152-0+f0)"], "Replaces"=[], "Supplements"=[], "Enhances"=[], "Product"=TRUE, "User visible"=TRUE, "Installed size (KB)"=0, "Package filesize (bytes)"=27547534, "Architecture"="windows_all", "Agent"="wininst", "MD5Checksum"=""}}, {126, "package attributes"={"Package Name"="ni-labview-2021-runtime-engine-x86", "Display name"="LabVIEW Runtime (32-bit)", "Version"="21.1.0.49476-0+f324", "Display version"="2021 SP1", "Synopsis"="The LabVIEW Runtime is a software add-on that enables engineers to run executables on a nondevelopment machine.", "Description"="The LabVIEW Runtime enables you to run executables created with the LabVIEW Application Builder on machines that do not have LabVIEW installed. The LabVIEW Runtime includes the libraries and other files necessary to run basic application types built in LabVIEW.", "Maintainer"="National Instruments", "Maintainer email address"="support@ni.com", "Category"="Programming Environments", "Homepage"="https://www.ni.com", "Release notes"="Refer to the NI website at https://www.ni.com/r/lv2021x1rm for installation instructions, known issues, bug fixes, compatibility information, and other important notices about this product.", "Depends"=["ni-activex-container (>= 17.1.2)", "ni-curl (>= 21.3.0)", "ni-deployment-framework-x86 (>= 21.0.0)", "ni-error-report-x86 (>= 20.1.0)", "ni-error-reporting-interface (>= 20.1.0)", "ni-labview-2021-realtime-nbfifo-x86 (>= 21.0.0)", "ni-labview-2021-runtime-engine-resource (>= 21.1.0)", "ni-logos (>= 21.0.0)", "ni-lv-web-server-labview-2021-runtime-engine-x86-support (>= 21.5.0)", "ni-matlab-interface (>= 21.1.0)", "ni-mdfsupport (>= 21.5.0)", "ni-mdnsresponder (>= 21.5.0)", "ni-metauninstaller (>= 21.5.0)", "ni-mkl-2017 (>= 17.0.1)", "ni-mkl-2020 (>= 20.0.0)", "ni-msiproperties (>= 21.5.0)", "ni-mstudio-cw3dgraph (>= 8.7.5)", "ni-msvcrt-2015 (>= 14.1.5)", "ni-python-interface (>= 21.1.0)", "ni-svcloc (>= 21.0.0)", "ni-systemlogging-utils (>= 20.0.0)", "ni-tdms (>= 21.1.0)", "ni-traceengine (>= 20.0.0)"], "Recommends"=[], "Suggests"=[], "Conflicts"=[], "Provides"=["0f5c3d28-ccea-37fa-af9e-554c677a3f03 (= 21.10.49476)", "251e8668-4013-3671-857c-61d46b2ac827 (= 21.10.49476)", "ni-labview-runtime-engine-x86 (= 21.1.0)", "ni-labview-2021-runtime-engine-x86 (= 21.1.0.49476-0+f324)"], "Replaces"=[], "Supplements"=[], "Enhances"=[], "Product"=TRUE, "User visible"=TRUE, "Installed size (KB)"=0, "Package filesize (bytes)"=29378434, "Architecture"="windows_x64", "Agent"="wininst", "MD5Checksum"=""}}, {127, "package attributes"={"Package Name"="ni-cvi-rte", "Display name"="LabWindows/CVI Shared Runtime Base", "Version"="20.0.1.49153-0+f1", "Display version"="2020 f1", "Synopsis"="The LabWindows/CVI Shared Runtime Base enables you to run most executables or use most DLLs created with LabWindows/CVI on a machine without the development environment installed.", "Description"="The LabWindows/CVI Shared Runtime Base enables you to run executables or use DLLs created with LabWindows/CVI that do not use separate LabWindows/CVI Shared Runtime libraries, and it must be present on any target computer on which you want to run your executable program. You can distribute the Runtime according to your license agreement.\n\nThe mark LabWindows is used under a license from Microsoft Corporation. Windows is a registered trademark of Microsoft Corporation in the United States and other countries.", "Maintainer"="National Instruments", "Maintainer email address"="support@ni.com", "Category"="Runtime", "Homepage"="http://www.ni.com", "Release notes"="", "Depends"=["ni-activex-container (>= 17.1.2)", "ni-cvi-activex (>= 20.0.0)", "ni-cvi-datasocket (>= 20.0.0)", "ni-cvi-instrsup (>= 20.0.1)", "ni-cvi-internet (>= 20.0.0)", "ni-cvi-opengl (>= 20.0.0)", "ni-cvi-openmp (>= 20.0.0)", "ni-cvi-runtime-core (>= 20.0.1)", "ni-cvi-runtime-realtime (>= 20.0.0)", "ni-cvi-usi (>= 20.0.0)", "ni-mdfsupport (>= 20.0.0)", "ni-mesa (>= 17.1.1)", "ni-metauninstaller (>= 20.0.0)", "ni-msiproperties (>= 20.0.0)", "ni-remote-configuration (>= 20.0.0)"], "Recommends"=["ni-cvi-analysis (>= 20.0.0)", "ni-cvi-dotnet (>= 20.0.0)", "ni-cvi-network-variable (>= 20.0.0)", "ni-cvi-networkstreams (>= 20.0.0)", "ni-cvi-tdms (>= 20.0.1)", "ni-datasocket (>= 20.0.0)"], "Suggests"=[], "Conflicts"=["80d3d303-75b9-4607-9312-e5fc68e5bfd2 (< 15.5.0)"], "Provides"=["5cf04e1e-f5d2-43ab-b9f1-5dcfb0df6cb6 (= 20.01.49153)", "80d3d303-75b9-4607-9312-e5fc68e5bfd2 (= 20.01.49153)", "ni-cvi-rte (= 20.0.1.49153-0+f1)"], "Replaces"=["80d3d303-75b9-4607-9312-e5fc68e5bfd2 (< 15.5.0)"], "Supplements"=[], "Enhances"=[], "Product"=FALSE, "User visible"=TRUE, "Installed size (KB)"=0, "Package filesize (bytes)"=863794, "Architecture"="windows_all", "Agent"="wininst", "MD5Checksum"=""}}, {128, "package attributes"={"Package Name"="ni-vipm", "Display name"="JKI VI Package Manager", "Version"="21.1.0.49472-0+f320", "Display version"="2021 SP1", "Synopsis"="VI Package Manager helps you discover, create, and install LabVIEW add-ons.", "Description"="VI Package Manager helps you discover and install LabVIEW add-ons from the LabVIEW Tools Network. VI Package Manager can also help you work smarter by building reusable code libraries and tools for your developers and customers.", "Maintainer"="JKI", "Maintainer email address"="https://vipm.jki.net/", "Category"="Add-Ons", "Homepage"="https://vipm.jki.net/", "Release notes"="Refer to the JKI website at https://vipm.jki.net/ for installation instructions, known issues, bug fixes, compatibility information, and other important notices about this product.", "Depends"=["ni-labview-2019-runtime-engine-x86 (>= 19.1.4)", "ni-mdfsupport (>= 21.5.0)", "ni-metauninstaller (>= 21.5.0)", "ni-msiproperties (>= 21.5.0)"], "Recommends"=[], "Suggests"=[], "Conflicts"=["ccfdbb6f-1545-4eba-93dd-9cc7cd53cdde (< 17.0.10000)"], "Provides"=["09f056a7-a421-4827-8514-430d9e6e1d62 (= 21.10.49472)", "5663f4ac-5ec4-4d6d-851f-c5c5bbe495ce (= 21.1.2754)", "ccfdbb6f-1545-4eba-93dd-9cc7cd53cdde (= 21.10.49472)", "ni-vipm (= 21.1.0.49472-0+f320)"], "Replaces"=["ccfdbb6f-1545-4eba-93dd-9cc7cd53cdde (< 17.0.10000)"], "Supplements"=[], "Enhances"=[], "Product"=TRUE, "User visible"=TRUE, "Installed size (KB)"=0, "Package filesize (bytes)"=72011214, "Architecture"="windows_x64", "Agent"="wininst", "MD5Checksum"=""}}, {129, "package attributes"={"Package Name"="ni-labview-2021-datafinder-runtime-x86", "Display name"="LabVIEW DataFinder Connectivity Runtime (32-bit)", "Version"="21.0.0.49153-0+f1", "Display version"="2021", "Synopsis"="LabVIEW DataFinder Connectivity Runtime enables the connection to DataFinder Server", "Description"="", "Maintainer"="National Instruments", "Maintainer email address"="support@ni.com", "Category"="Runtime", "Homepage"="https://www.ni.com", "Release notes"="Place Holder", "Depends"=["ni-datafinder-client-api (>= 21.0.0)", "ni-dataplugins-aop5 (>= 19.5.0)", "ni-labview-2021-runtime-engine-x86 (>= 21.0.0)", "ni-mdfsupport (>= 21.0.0)", "ni-metauninstaller (>= 21.0.0)", "ni-msvcrt-2015 (>= 14.1.5)", "ni-usi-core (>= 21.0.0)"], "Recommends"=[], "Suggests"=[], "Conflicts"=[], "Provides"=["7e2dacda-6020-4633-bc96-e4ed2c4c2881 (= 21.00.49153)", "ni-labview-2021-datafinder-runtime-x86 (= 21.0.0.49153-0+f1)"], "Replaces"=[], "Supplements"=[], "Enhances"=[], "Product"=FALSE, "User visible"=TRUE, "Installed size (KB)"=0, "Package filesize (bytes)"=740294, "Architecture"="windows_x64", "Agent"="wininst", "MD5Checksum"=""}}, {130, "package attributes"={"Package Name"="ni-distributed-system-manager-2021", "Display name"="NI Distributed System Manager 2021", "Version"="21.0.0.49488-0+f336", "Display version"="21.0.0", "Synopsis"="Support for creating and monitoring variables, processes, I/O servers, and Web services, as well as interacting with the NI Variable Engine and managing security aliases.", "Description"="", "Maintainer"="National Instruments", "Maintainer email address"="support@ni.com", "Category"="Runtime", "Homepage"="https://www.ni.com", "Release notes"="Refer to the NI website at https://www.ni.com/r/lv2021rm for installation instructions, known issues, bug fixes, compatibility information, and other important notices about this product.", "Depends"=["ni-deployment-framework-x86 (>= 21.0.0)", "ni-labview-2021-runtime-engine-x86 (>= 21.0.0)", "ni-mdfsupport (>= 21.0.0)", "ni-metauninstaller (>= 21.0.0)"], "Recommends"=[], "Suggests"=[], "Conflicts"=["ecaf201a-e0cc-3bc4-984d-e94c3af29064 (< 19.0.0)"], "Provides"=["ecaf201a-e0cc-3bc4-984d-e94c3af29064 (= 21.00.49488)", "ni-distributed-system-manager-2021 (= 21.0.0.49488-0+f336)"], "Replaces"=["ecaf201a-e0cc-3bc4-984d-e94c3af29064 (< 19.0.0)"], "Supplements"=[], "Enhances"=[], "Product"=TRUE, "User visible"=TRUE, "Installed size (KB)"=0, "Package filesize (bytes)"=17139738, "Architecture"="windows_x64", "Agent"="wininst", "MD5Checksum"=""}}, {131, "package attributes"={"Package Name"="ni-cvi-runtime-engine", "Display name"="LabWindows/CVI Shared Runtime", "Version"="20.0.1.49154-0+f2", "Display version"="2020 f1", "Synopsis"="The LabWindows/CVI Shared Runtime enables you to run executables or use DLLs created with LabWindows/CVI on machines without LabWindows/CVI installed.", "Description"="The LabWindows/CVI Shared Runtime is backwards compatible and may be used with applications that were created with previous versions of LabWindows/CVI. You can distribute the Runtime according to your license agreement. The mark LabWindows is used under a license from Microsoft Corporation. Windows is a registered trademark of Microsoft Corporation in the United States and other countries.", "Maintainer"="National Instruments", "Maintainer email address"="support@ni.com", "Category"="Runtime", "Homepage"="http://www.ni.com", "Release notes"="Refer to the NI website at http://www.ni.com/r/cvi2020readme for installation instructions, known issues, bug fixes, compatibility information, and other important notices about this product.\n\nYou must have at least 200 MB of free space available to install this product.", "Depends"=["ni-cvi-analysis (>= 20.0.0)", "ni-cvi-dotnet (>= 20.0.0)", "ni-cvi-network-variable (>= 20.0.0)", "ni-cvi-networkstreams (>= 20.0.0)", "ni-cvi-rte (>= 20.0.1)", "ni-cvi-tdms (>= 20.0.1)", "ni-datasocket (>= 20.0.0)", "ni-metauninstaller (>= 20.0.0)"], "Recommends"=[], "Suggests"=[], "Conflicts"=["8c766eca-a110-4317-a767-5027278427ae (< 19.0.0)"], "Provides"=["8c766eca-a110-4317-a767-5027278427ae (= 20.01.49154)", "ni-cvi-runtime-engine (= 20.0.1.49154-0+f2)"], "Replaces"=["8c766eca-a110-4317-a767-5027278427ae (< 19.0.0)"], "Supplements"=[], "Enhances"=[], "Product"=TRUE, "User visible"=TRUE, "Installed size (KB)"=0, "Package filesize (bytes)"=434570, "Architecture"="windows_all", "Agent"="wininst", "MD5Checksum"=""}}, {132, "package attributes"={"Package Name"="ni-labview-2021-core-x86-en", "Display name"="LabVIEW (32-bit) English", "Version"="21.1.0.49478-0+f326", "Display version"="2021 SP1", "Synopsis"="LabVIEW is systems engineering software for applications that require test, measurement, and control with rapid access to hardware and data insights.", "Description"="The LabVIEW programming environment simplifies hardware integration for engineering applications so that you have a consistent way to acquire data from NI and third-party hardware. LabVIEW reduces the complexity of programming, so you can focus on your unique engineering problem. LabVIEW enables you to immediately visualize results with built-in, drag-and-drop engineering user interface creation and integrated data viewers. To turn your acquired data into real business results, you can develop algorithms for data analysis and advanced control with included math and signal processing IP or reuse your own libraries from a variety of tools. To ensure compatibility with other engineering tools, LabVIEW can interoperate with, and reuse libraries from, other software and open-source languages.", "Maintainer"="National Instruments", "Maintainer email address"="support@ni.com", "Category"="Programming Environments", "Homepage"="https://www.ni.com", "Release notes"="Refer to the NI website at https://www.ni.com/r/lv2021x1rm for installation instructions, known issues, bug fixes, compatibility information, and other important notices about this product.", "Depends"=["ni-assistant-framework-labview-2021-codegen-x86-support (>= 21.0.0)", "ni-assistant-framework-x86 (>= 21.0.0)", "ni-ceip-x86 (>= 21.5.0)", "ni-codesignapi (>= 21.0.0)", "ni-curl (>= 21.3.0)", "ni-cvi-labview-dll-builder-15.1.0 (>= 15.1.1)", "ni-cvi-runtime-engine (>= 20.0.1)", "ni-daqmx-labview-shared-docs (>= 21.3.0)", "ni-datasocket (>= 21.0.0)", "ni-distributed-system-manager-2021 (>= 21.0.0)", "ni-error-report-x86 (>= 20.1.0)", "ni-example-finder-x86 (>= 21.0.0)", "ni-iioa-labview-2020-support-x86 (>= 20.0.0)", "ni-json-map (>= 21.0.0)", "ni-labview-2021-coreother-x86-en (>= 21.1.0)", "ni-labview-2021-deployable-license (>= 21.1.0)", "ni-labview-2021-example-x86-en (>= 21.1.0)", "ni-labview-2021-executable-x86 (>= 21.1.0)", "ni-labview-2021-help-x86-en (>= 21.1.0)", "ni-labview-2021-helpchm (>= 21.1.0)", "ni-labview-2021-license (>= 21.1.0)", "ni-labview-2021-manuals-x86-en (>= 21.1.0)", "ni-labview-2021-measapps-chm (>= 21.0.0)", "ni-labview-2021-runtime-engine-x86 (>= 21.1.0)", "ni-labview-2021-scripting-codegen-x86 (>= 21.0.0)", "ni-labview-2021-simulation-x86 (>= 21.1.0)", "ni-labview-2021-vilib-x86-en (>= 21.1.0)", "ni-labview-c-interface (>= 1.0.4)", "ni-labview-max-xml (>= 19.0.0)", "ni-labview-vicompare-x86 (>= 21.0.0)", "ni-labview-vimerge-x86 (>= 21.0.0)", "ni-logos (>= 21.0.0)", "ni-logos-labview-2021-support-x86-en (>= 21.1.0)", "ni-mdfsupport (>= 21.5.0)", "ni-metauninstaller (>= 21.5.0)", "ni-mkl-2020 (>= 20.0.0)", "ni-msdotnet4x (>= 4.6.3)", "ni-msvcrt-2015 (>= 14.1.5)", "ni-mxs (>= 21.5.0)", "ni-opc-support (>= 21.0.0)", "ni-package-builder-labview-2021-support-x86-en (>= 21.1.0)", "ni-python-interface (>= 21.1.0)", "ni-search-labview-2021-support-x86 (>= 21.0.0)", "ni-slcp-x86 (>= 21.5.0)", "ni-ssl-labview-2021-x86-support (>= 21.0.0)", "ni-ssp-notifier (>= 20.6.0)", "ni-svcloc (>= 21.0.0)", "ni-system-webserver (>= 21.5.0)", "ni-system-webserver-appserver (>= 21.5.0)", "ni-systemlogging-utils (>= 20.0.0)", "ni-update-service (>= 21.0.0)", "ni-usi-core (>= 21.0.0)", "ni-variable-engine (>= 21.0.0)", "ni-variable-engine-labview-2021-support-x86-en (>= 21.1.0)", "ni-vipm-helper (>= 21.1.0)", "ni-web-based-configuration (>= 21.5.0)", "ni-web-pipeline-19.0 (>= 19.0.0)", "ni-web-services-labview-2021-x86-support (>= 21.5.0)"], "Recommends"=["mgi-solution-explorer (>= 2.5.0)", "ni-certificates (>= 21.5.0)", "ni-labview-2021-database-toolkit-x86 (>= 21.0.0)", "ni-labview-2021-datafinder-connectivity-x86 (>= 21.0.0)", "ni-labview-2021-report-generation-toolkit-x86 (>= 21.0.0)", "ni-labview-command-line-interface-x86 (>= 4.0.0)", "ni-max (>= 21.5.0)", "ni-syscfg-labview-2021-support-x86 (>= 21.5.0)", "ni-tdm-excel-addin (>= 19.0.0)", "ni-vipm (>= 21.1.0)", "ni-webservices-amqp-labview-2021-support-x86 (>= 21.5.0)"], "Suggests"=["ni-labview-2021-ff-runtime-engine-x86 (>= 21.1.0)", "ni-wif (>= 20.5.1)"], "Conflicts"=["ni-labview-2021-x86-de (>= 0.0.0)", "ni-labview-2021-x86-fr (>= 0.0.0)", "ni-labview-2021-x86-ja (>= 0.0.0)", "ni-labview-2021-x86-ko (>= 0.0.0)", "ni-labview-2021-x86-zh-cn (>= 0.0.0)"], "Provides"=["1c63d3e6-6922-3263-ab3c-5a79761ae0fc (= 21.10.49478)", "456b17ca-f321-36cf-abe1-12d8844d4395 (= 21.10.49478)", "ni-labview (= 21.1.0)", "ni-labview-2021-x86 (= 21.1.0)", "ni-labview-2021-x86-en", "ni-labview-2021-core-x86-en (= 21.1.0.49478-0+f326)"], "Replaces"=[], "Supplements"=[], "Enhances"=[], "Product"=TRUE, "User visible"=TRUE, "Installed size (KB)"=0, "Package filesize (bytes)"=2419060, "Architecture"="windows_x64", "Agent"="wininst", "MD5Checksum"=""}}, {133, "package attributes"={"Package Name"="ni-labview-2021-database-toolkit-x86", "Display name"="LabVIEW Database Connectivity Toolkit (32-bit)", "Version"="21.0.0.49154-0+f2", "Display version"="2021", "Synopsis"="The LabVIEW Database Connectivity Toolkit helps you connect to local and remote databases and implement common database operations.", "Description"="The LabVIEW Database Connectivity Toolkit is a software add-on for LabVIEW that helps you perform many database operations without using structured query language (SQL) programming. It readily connects to popular databases, such as Microsoft Access, SQL Server, and Oracle. If you need advanced database functionality and flexibility, the LabVIEW Database Connectivity Toolkit also offers complete SQL capabilities.", "Maintainer"="National Instruments", "Maintainer email address"="support@ni.com", "Category"="Add-Ons", "Homepage"="https://www.ni.com", "Release notes"="Refer to the NI website at https://www.ni.com/r/lvdct2021rm for installation instructions, known issues, bug fixes, compatibility information, and other important notices about this product.", "Depends"=["ni-labview-2021-database-toolkit-lic (>= 21.0.0)", "ni-labview-2021-x86 (>= 21.0.0)", "ni-mdfsupport (>= 21.0.0)", "ni-metauninstaller (>= 21.0.0)"], "Recommends"=[], "Suggests"=[], "Conflicts"=[], "Provides"=["6ac8b688-f4ea-4625-90b8-acec8ec0a211 (= 21.00.49154)", "ni-labview-2021-database-toolkit-x86 (= 21.0.0.49154-0+f2)"], "Replaces"=[], "Supplements"=["ni-labview-2021-x86 (>= 21.0.0)"], "Enhances"=[], "Product"=TRUE, "User visible"=TRUE, "Installed size (KB)"=0, "Package filesize (bytes)"=5704496, "Architecture"="windows_x64", "Agent"="wininst", "MD5Checksum"=""}}, {134, "package attributes"={"Package Name"="ni-labview-2021-datafinder-connectivity-x86", "Display name"="LabVIEW DataFinder Connectivity VIs (32-bit)", "Version"="21.0.0.49152-0+f0", "Display version"="2021", "Synopsis"="The LabVIEW DataFinder Connectivity VIs software provides a DataFinder Server interface for LabVIEW applications.", "Description"="The LabVIEW DataFinder Connectivity VIs software add-on for LabVIEW connects your LabVIEW applications with the indexing and searching capabilities of DataFinder Server. Using this functionality, you can design interfaces to search a DataFinder Server index and find valuable information in your test files. DataFinder technology indexes the properties and metadata in your test files and stores them in a behind-the-scenes, self-scaling database for fast search and retrieval. DataFinder Server enables distributed networked data communications, storage, and mining.", "Maintainer"="National Instruments", "Maintainer email address"="support@ni.com", "Category"="Add-Ons", "Homepage"="https://www.ni.com", "Release notes"="Refer to the NI website at https://www.ni.com/r/lv2021rm for installation instructions, known issues, bug fixes, compatibility information, and other important notices about this product.", "Depends"=["ni-labview-2021-datafinder-runtime-x86 (>= 21.0.0)", "ni-labview-2021-x86 (>= 21.0.0)", "ni-mdfsupport (>= 21.0.0)", "ni-metauninstaller (>= 21.0.0)"], "Recommends"=[], "Suggests"=[], "Conflicts"=[], "Provides"=["86e2bedd-b28e-4270-ae5c-d47f2004fc7f (= 21.00.49152)", "ni-labview-2021-datafinder-connectivity-x86 (= 21.0.0.49152-0+f0)"], "Replaces"=[], "Supplements"=[], "Enhances"=["ni-labview-2021-x86 (>= 21.0.0)"], "Product"=TRUE, "User visible"=TRUE, "Installed size (KB)"=0, "Package filesize (bytes)"=2352712, "Architecture"="windows_x64", "Agent"="wininst", "MD5Checksum"=""}}, {135, "package attributes"={"Package Name"="ni-labview-2021-report-generation-toolkit-x86", "Display name"="LabVIEW Report Generation Toolkit (32-bit)", "Version"="21.0.0.49154-0+f2", "Display version"="2021", "Synopsis"="The LabVIEW Report Generation Toolkit provides VIs for programmatically creating and editing Microsoft Word and Excel reports from LabVIEW.", "Description"="The LabVIEW Report Generation Toolkit is a software add-on for LabVIEW that can generate reports on manufacturing test results or compile process statistics to improve your production yields. With this toolkit, you can easily populate report templates, email reports, execute macros, and manage report layout and appearance.", "Maintainer"="National Instruments", "Maintainer email address"="support@ni.com", "Category"="Add-Ons", "Homepage"="https://www.ni.com", "Release notes"="Refer to the NI website at https://www.ni.com/r/lvrgt2021rm for installation instructions, known issues, bug fixes, compatibility information, and other important notices about this product.", "Depends"=["ni-labview-2021-report-generation-toolkit-lic (>= 21.0.0)", "ni-labview-2021-x86 (>= 21.0.0)", "ni-mdfsupport (>= 21.0.0)", "ni-metauninstaller (>= 21.0.0)"], "Recommends"=[], "Suggests"=[], "Conflicts"=[], "Provides"=["c075d068-8cb6-4666-8419-8a9f7a452457 (= 21.00.49154)", "ni-labview-2021-report-generation-toolkit-x86 (= 21.0.0.49154-0+f2)"], "Replaces"=[], "Supplements"=["ni-labview-2021-x86 (>= 21.0.0)"], "Enhances"=[], "Product"=TRUE, "User visible"=TRUE, "Installed size (KB)"=0, "Package filesize (bytes)"=6817692, "Architecture"="windows_x64", "Agent"="wininst", "MD5Checksum"=""}}, {136, "package attributes"={"Package Name"="ni-syscfg-labview-2021-support-x86", "Display name"="NI System Configuration Support for LabVIEW 2021 (32-bit)", "Version"="21.5.0.49392-0+f240", "Display version"="21.5.0", "Synopsis"="Provides libraries, documentation, and examples for using the NI System Configuration API to discover and configure systems and devices within LabVIEW 2021 (32-bit).", "Description"="", "Maintainer"="National Instruments", "Maintainer email address"="support@ni.com", "Category"="Add-Ons", "Homepage"="https://www.ni.com", "Release notes"="", "Depends"=["ni-mdfsupport (>= 21.5.0)", "ni-metauninstaller (>= 21.5.0)", "ni-syscfg-labview-support (>= 21.5.0)", "ni-syscfg-runtime (>= 21.5.0)", "ni-labview-2021-x86 (>= 21.0.0)"], "Recommends"=[], "Suggests"=[], "Conflicts"=["50dc228b-a5b3-47a2-9367-bad46b8e8bfd (< 17.99.9)"], "Provides"=["50dc228b-a5b3-47a2-9367-bad46b8e8bfd (= 21.50.49392)", "ni-syscfg-labview-2021-support-x86 (= 21.5.0.49392-0+f240)"], "Replaces"=["50dc228b-a5b3-47a2-9367-bad46b8e8bfd (< 17.99.9)"], "Supplements"=["ni-labview-2021-x86 (>= 21.0.0)"], "Enhances"=[], "Product"=FALSE, "User visible"=TRUE, "Installed size (KB)"=0, "Package filesize (bytes)"=12368540, "Architecture"="windows_x64", "Agent"="wininst", "MD5Checksum"=""}}, {137, "package attributes"={"Package Name"="ni-webservices-amqp-labview-2021-support-x86", "Display name"="NI Web Server Development Support for LabVIEW 2021 32-bit", "Version"="21.5.0.49152-0+f0", "Display version"="21.5.0", "Synopsis"="Provides support for developing G Web services in LabVIEW 2021 (32-bit) hosted by NI Web Server.", "Description"="", "Maintainer"="National Instruments", "Maintainer email address"="support@ni.com", "Category"="Add-Ons", "Homepage"="https://www.ni.com", "Release notes"="", "Depends"=["ni-labview-2021-x86 (>= 21.0.0)", "ni-mdfsupport (>= 21.5.0)", "ni-metauninstaller (>= 21.5.0)", "ni-webservices-amqp-deployment-support-x86 (>= 21.5.0)"], "Recommends"=[], "Suggests"=[], "Conflicts"=[], "Provides"=["e0c60e83-8804-32a9-a787-0a293daf2eae (= 21.50.49152)", "ni-webservices-amqp-labview-2021-support-x86 (= 21.5.0.49152-0+f0)"], "Replaces"=[], "Supplements"=["ni-labview-2021-x86 (>= 21.0.0)"], "Enhances"=[], "Product"=FALSE, "User visible"=TRUE, "Installed size (KB)"=0, "Package filesize (bytes)"=886044, "Architecture"="windows_x64", "Agent"="wininst", "MD5Checksum"=""}}, {150, "package attributes"={"Package Name"="ni-iotrace", "Display name"="NI I/O Trace", "Version"="20.0.0.49152-0+f0", "Display version"="20.0.0", "Synopsis"="Debugging utility for monitoring function calls to various National Instruments APIs.", "Description"="NI I/O Trace is an application that monitors, records, and displays National Instruments API calls made by applications. Use NI I/O Trace to quickly locate and analyze any erroneous National Instruments API calls that your application makes, and to verify that the communication with your instrument is correct.", "Maintainer"="National Instruments", "Maintainer email address"="support@ni.com", "Category"="Utilities", "Homepage"="http://www.ni.com", "Release notes"="", "Depends"=["ni-labview-2019-runtime-engine-x86 (>= 19.1.1)", "ni-launcher (>= 20.0.0)", "ni-mdfsupport (>= 20.0.0)", "ni-metauninstaller (>= 20.0.0)", "ni-msvcrt-2015 (>= 14.1.5)"], "Recommends"=[], "Suggests"=[], "Conflicts"=["b87bcb47-3c93-11d4-88e6-0008c7c25519 (< 17.0.0)"], "Provides"=["0a0c3489-a948-4922-b9ac-92e09de3162e (= 20.00.49152)", "b87bcb47-3c93-11d4-88e6-0008c7c25519 (= 20.00.49152)", "ni-iotrace (= 20.0.0.49152-0+f0)"], "Replaces"=["b87bcb47-3c93-11d4-88e6-0008c7c25519 (< 17.0.0)"], "Supplements"=[], "Enhances"=[], "Product"=FALSE, "User visible"=TRUE, "Installed size (KB)"=0, "Package filesize (bytes)"=3903218, "Architecture"="windows_all", "Agent"="wininst", "MD5Checksum"=""}}, {153, "package attributes"={"Package Name"="ni-visa-runtime", "Display name"="NI-VISA Runtime", "Version"="20.0.0.49152-0+f0", "Display version"="20.0.0", "Synopsis"="Provides an API for controlling USB, TCPIP, GPIB, Serial, PXI, and other types of instruments.", "Description"="", "Maintainer"="National Instruments", "Maintainer email address"="support@ni.com", "Category"="Drivers", "Homepage"="http://www.ni.com", "Release notes"="", "Depends"=["ni-curl (>= 20.0.0)", "ni-mdfsupport (>= 20.0.0)", "ni-mdnsresponder (>= 19.0.0)", "ni-metauninstaller (>= 20.0.0)", "ni-msiproperties (>= 20.0.0)", "ni-msvcrt-2015 (>= 14.1.5)", "ni-svcloc (>= 20.0.0)", "ni-visa-errors (>= 20.0.0)", "ni-visa-headers (>= 20.0.0)", "ni-visa-passport-enet (>= 20.0.0)", "ni-visa-passport-enet-serial (>= 20.0.0)", "ni-visa-passport-gpib (>= 20.0.0)", "ni-visa-passport-pxi (>= 20.0.0)", "ni-visa-passport-remote (>= 20.0.0)", "ni-visa-passport-serial (>= 20.0.0)", "ni-visa-passport-tulip (>= 20.0.0)", "ni-visa-passport-usb (>= 20.0.0)", "ni-visa-shared-components (>= 5.12.0)", "ni-visa-sysapi (>= 20.0.0)"], "Recommends"=[], "Suggests"=[], "Conflicts"=["8627993a-3f66-483c-a562-0d3ba3f267b1 (< 17.0.0)"], "Provides"=["8627993a-3f66-483c-a562-0d3ba3f267b1 (= 20.00.49152)", "b44b9383-dfac-4ff5-a056-354ccd10bd77 (= 20.00.49152)", "ni-visa-runtime (= 20.0.0.49152-0+f0)"], "Replaces"=["8627993a-3f66-483c-a562-0d3ba3f267b1 (< 17.0.0)"], "Supplements"=[], "Enhances"=[], "Product"=FALSE, "User visible"=TRUE, "Installed size (KB)"=0, "Package filesize (bytes)"=1481252, "Architecture"="windows_all", "Agent"="wininst", "MD5Checksum"=""}}, {154, "package attributes"={"Package Name"="ni-visa-interactive-control", "Display name"="NI-VISA Interactive Control", "Version"="20.0.0.49152-0+f0", "Display version"="20.0.0", "Synopsis"="Provides the NI-VISA Interactive Control utility to interact and communicate with NI-VISA resources.", "Description"="", "Maintainer"="National Instruments", "Maintainer email address"="support@ni.com", "Category"="Drivers", "Homepage"="http://www.ni.com", "Release notes"="", "Depends"=["ni-labview-2019-runtime-engine-x86 (>= 19.1.1)", "ni-launcher (>= 19.0.0)", "ni-mdfsupport (>= 20.0.0)", "ni-metauninstaller (>= 20.0.0)", "ni-visa-documentation (>= 20.0.0)", "ni-visa-runtime (>= 20.0.0)"], "Recommends"=[], "Suggests"=[], "Conflicts"=["8b393b9f-4233-4ae4-9f2e-982bedd305d3 (< 17.0.0)"], "Provides"=["65188d4e-5a04-4431-89bb-ca12a5c97de3 (= 20.00.49152)", "8b393b9f-4233-4ae4-9f2e-982bedd305d3 (= 20.00.49152)", "ni-visa-interactive-control (= 20.0.0.49152-0+f0)"], "Replaces"=["8b393b9f-4233-4ae4-9f2e-982bedd305d3 (< 17.0.0)"], "Supplements"=[], "Enhances"=[], "Product"=FALSE, "User visible"=TRUE, "Installed size (KB)"=0, "Package filesize (bytes)"=3641194, "Architecture"="windows_all", "Agent"="wininst", "MD5Checksum"=""}}, {155, "package attributes"={"Package Name"="ni-visa-configuration", "Display name"="NI-VISA Configuration Support", "Version"="20.0.0.49152-0+f0", "Display version"="20.0.0", "Synopsis"="Provides support for viewing and/or configuring NI-VISA resources in NI MAX.", "Description"="", "Maintainer"="National Instruments", "Maintainer email address"="support@ni.com", "Category"="Drivers", "Homepage"="http://www.ni.com", "Release notes"="", "Depends"=["ni-max (>= 20.0.0)", "ni-mdfsupport (>= 20.0.0)", "ni-metauninstaller (>= 20.0.0)", "ni-msvcrt-2015 (>= 14.1.5)", "ni-visa-runtime (>= 20.0.0)"], "Recommends"=[], "Suggests"=[], "Conflicts"=["093eeccf-de2b-4226-b7e5-b1fd4028a783 (< 17.0.0)"], "Provides"=["093eeccf-de2b-4226-b7e5-b1fd4028a783 (= 20.00.49152)", "48be9cc1-5b4f-43f2-aab5-cb4117eea019 (= 20.00.49152)", "ni-visa-configuration (= 20.0.0.49152-0+f0)"], "Replaces"=["093eeccf-de2b-4226-b7e5-b1fd4028a783 (< 17.0.0)"], "Supplements"=[], "Enhances"=[], "Product"=FALSE, "User visible"=TRUE, "Installed size (KB)"=0, "Package filesize (bytes)"=4282110, "Architecture"="windows_all", "Agent"="wininst", "MD5Checksum"=""}}, {156, "package attributes"={"Package Name"="ni-pxiplatformservices-provider", "Display name"="NI PXI Platform Services Configuration", "Version"="20.0.0.49152-0+f0", "Display version"="20.0.0", "Synopsis"="Allows PXI system configuration in Measurement & Automation Explorer.", "Description"="", "Maintainer"="National Instruments", "Maintainer email address"="support@ni.com", "Category"="Drivers", "Homepage"="http://www.ni.com", "Release notes"="", "Depends"=["ni-max (>= 20.0.0)", "ni-mdfsupport (>= 19.5.0)", "ni-metauninstaller (>= 19.5.0)", "ni-msvcrt-2015 (>= 14.1.5)", "ni-pxiplatformservices-runtime (>= 20.0.0)"], "Recommends"=[], "Suggests"=[], "Conflicts"=["84494c93-949f-40db-8ce2-d9728e8eaa49 (< 17.0.0)"], "Provides"=["84494c93-949f-40db-8ce2-d9728e8eaa49 (= 20.00.49152)", "ni-pxiplatformservices-provider (= 20.0.0.49152-0+f0)"], "Replaces"=["84494c93-949f-40db-8ce2-d9728e8eaa49 (< 17.0.0)"], "Supplements"=[], "Enhances"=[], "Product"=FALSE, "User visible"=TRUE, "Installed size (KB)"=0, "Package filesize (bytes)"=8369750, "Architecture"="windows_all", "Agent"="wininst", "MD5Checksum"=""}}, {157, "package attributes"={"Package Name"="ni-visa-server", "Display name"="NI-VISA Server", "Version"="20.0.0.49152-0+f0", "Display version"="20.0.0", "Synopsis"="Provides remote access to resources on the current machine.", "Description"="", "Maintainer"="National Instruments", "Maintainer email address"="support@ni.com", "Category"="Drivers", "Homepage"="http://www.ni.com", "Release notes"="", "Depends"=["ni-launcher (>= 19.0.0)", "ni-mdfsupport (>= 20.0.0)", "ni-metauninstaller (>= 20.0.0)", "ni-msvcrt-2015 (>= 14.1.5)", "ni-rpc (>= 19.0.0)", "ni-visa-configuration (>= 20.0.0)", "ni-visa-runtime (>= 20.0.0)"], "Recommends"=[], "Suggests"=[], "Conflicts"=["951e7f56-f1cd-403c-b138-9befc6ceb343 (< 17.0.0)"], "Provides"=["951e7f56-f1cd-403c-b138-9befc6ceb343 (= 20.00.49152)", "ni-visa-server (= 20.0.0.49152-0+f0)"], "Replaces"=["951e7f56-f1cd-403c-b138-9befc6ceb343 (< 17.0.0)"], "Supplements"=[], "Enhances"=[], "Product"=FALSE, "User visible"=TRUE, "Installed size (KB)"=0, "Package filesize (bytes)"=475510, "Architecture"="windows_all", "Agent"="wininst", "MD5Checksum"=""}}, {160, "package attributes"={"Package Name"="ni-visa-labview-2017-support-x86", "Display name"="NI-VISA LabVIEW 2017 (32-Bit) Support", "Version"="20.0.0.49152-0+f0", "Display version"="20.0.0", "Synopsis"="Provides NI-VISA Probes for using NI-VISA resources within LabVIEW 2017 (32-bit).", "Description"="", "Maintainer"="National Instruments", "Maintainer email address"="support@ni.com", "Category"="Drivers", "Homepage"="http://www.ni.com", "Release notes"="", "Depends"=["ni-mdfsupport (>= 20.0.0)", "ni-metauninstaller (>= 20.0.0)", "ni-visa-development-support-compatibility (>= 20.0.0)", "aa4b25c0-a1f6-472e-8f76-32e406b7e44d (>= 17.0.0) | 7a80ea72-c69d-4740-afbf-326544b9462c (>= 17.1.0)"], "Recommends"=[], "Suggests"=[], "Conflicts"=["d8c88edf-395a-4334-8067-9650c6a28d83 (< 17.0.0)"], "Provides"=["d8c88edf-395a-4334-8067-9650c6a28d83 (= 20.00.49152)", "ni-visa-labview-2017-support-x86 (= 20.0.0.49152-0+f0)"], "Replaces"=["d8c88edf-395a-4334-8067-9650c6a28d83 (< 17.0.0)"], "Supplements"=["7a80ea72-c69d-4740-afbf-326544b9462c (>= 17.1.0)", "aa4b25c0-a1f6-472e-8f76-32e406b7e44d (>= 17.0.0)"], "Enhances"=[], "Product"=FALSE, "User visible"=TRUE, "Installed size (KB)"=0, "Package filesize (bytes)"=735922, "Architecture"="windows_all", "Agent"="wininst", "MD5Checksum"=""}}, {161, "package attributes"={"Package Name"="ni-visa-driver-development-wizard", "Display name"="NI-VISA Driver Development Wizard", "Version"="20.0.0.49152-0+f0", "Display version"="20.0.0", "Synopsis"="Provides the NI-VISA Driver Development Wizard for creating INF files for PXI and USB.", "Description"="", "Maintainer"="National Instruments", "Maintainer email address"="support@ni.com", "Category"="Drivers", "Homepage"="http://www.ni.com", "Release notes"="", "Depends"=["ni-labview-2019-runtime-engine-x86 (>= 19.1.1)", "ni-launcher (>= 19.0.0)", "ni-mdfsupport (>= 20.0.0)", "ni-metauninstaller (>= 20.0.0)", "ni-visa-development-support-compatibility (>= 20.0.0)"], "Recommends"=[], "Suggests"=[], "Conflicts"=["b0068589-eb45-4591-b602-ed3a3a259dca (< 17.0.0)"], "Provides"=["b0068589-eb45-4591-b602-ed3a3a259dca (= 20.00.49152)", "ni-visa-driver-development-wizard (= 20.0.0.49152-0+f0)"], "Replaces"=["b0068589-eb45-4591-b602-ed3a3a259dca (< 17.0.0)"], "Supplements"=[], "Enhances"=[], "Product"=FALSE, "User visible"=TRUE, "Installed size (KB)"=0, "Package filesize (bytes)"=3456406, "Architecture"="windows_all", "Agent"="wininst", "MD5Checksum"=""}}, {162, "package attributes"={"Package Name"="ni-visa", "Display name"="NI-VISA", "Version"="20.0.0.49152-0+f0", "Display version"="20.0.0", "Synopsis"="NI-VISA provides support for customers using Ethernet, GPIB, serial, USB, and other types of instruments.", "Description"="NI-VISA is an NI instrument driver that is an implementation of the Virtual Instrument Software Architecture (VISA) I/O standard. VISA is a standard for configuring, programming, and troubleshooting instrumentation systems comprising GPIB, VXI, PXI, serial (RS232/RS485), Ethernet/LXI, and/or USB interfaces. NI-VISA includes utilities, low-level control features, and examples to help you create your application.", "Maintainer"="National Instruments", "Maintainer email address"="support@ni.com", "Category"="Drivers", "Homepage"="http://www.ni.com", "Release notes"="Refer to the NI website at http://www.ni.com/r/visa200readme for installation instructions, known issues, bug fixes, compatibility information, and other important notices about this product.\n\nYou must have at least 910 MB of free space available to install this product.\n\nThis version supports LabVIEW NXG 5.0.", "Depends"=["ni-mdfsupport (>= 20.0.0)", "ni-metauninstaller (>= 20.0.0)", "ni-update-service (>= 19.0.0)", "ni-visa-runtime (>= 20.0.0)"], "Recommends"=["ni-iotrace (>= 20.0.0)", "ni-pxiplatformservices-runtime (>= 20.0.0)", "ni-visa-19.0-dotnet-development-support (>= 19.0.0)", "ni-visa-19.0-dotnet-runtime (>= 19.0.0)", "ni-visa-20.0.0-realtime-bin (>= 20.0.0)", "ni-visa-c-examples (>= 20.0.0)", "ni-visa-configuration (>= 20.0.0)", "ni-visa-driver-development-wizard (>= 20.0.0)", "ni-visa-interactive-control (>= 20.0.0)", "ni-visa-labview-2017-support (>= 20.0.0)", "ni-visa-labview-2017-support-x86 (>= 20.0.0)", "ni-visa-labview-2018-support (>= 20.0.0)", "ni-visa-labview-2018-support-x86 (>= 20.0.0)", "ni-visa-labview-2019-support (>= 20.0.0)", "ni-visa-labview-2019-support-x86 (>= 20.0.0)", "ni-visa-labview-2020-support (>= 20.0.0)", "ni-visa-labview-2020-support-x86 (>= 20.0.0)", "ni-visa-labview-nxg-5.0.0-rte-support (>= 20.0.0)", "ni-visa-labview-nxg-5.0.0-support (>= 20.0.0)"], "Suggests"=["ni-linux-rt-system-image-20.0.0 (>= 20.0.0)", "ni-visa-cvi-examples (>= 20.0.0)", "ni-visa-cvi-support (>= 20.0.0)", "ni-visa-server (>= 20.0.0)"], "Conflicts"=["8cf4f6cd-20c9-4bbc-962d-8d8c0d72e22d (< 16.99.0)"], "Provides"=["8cf4f6cd-20c9-4bbc-962d-8d8c0d72e22d (= 20.00.49152)", "ni-visa (= 20.0.0.49152-0+f0)"], "Replaces"=["8cf4f6cd-20c9-4bbc-962d-8d8c0d72e22d (< 16.99.0)"], "Supplements"=[], "Enhances"=[], "Product"=TRUE, "User visible"=TRUE, "Installed size (KB)"=0, "Package filesize (bytes)"=377744, "Architecture"="windows_all", "Agent"="wininst", "MD5Checksum"=""}}, {164, "package attributes"={"Package Name"="ni-labview-2021-vi-analyzer-toolkit-x86", "Display name"="LabVIEW VI Analyzer Toolkit (32-bit)", "Version"="21.0.0.49154-0+f2", "Display version"="2021", "Synopsis"="The LabVIEW VI Analyzer Toolkit helps you perform static code analysis to improve the quality and readability of your LabVIEW code.", "Description"="The LabVIEW VI Analyzer Toolkit is a software add-on for LabVIEW that helps you improve graphical code developed in LabVIEW. With this toolkit, you can configure more than 90 included tests for automated code review and static code analysis of all VIs in an application, or you can create your own using the test creation wizard. The LabVIEW VI Analyzer Toolkit provides debugging tools that help you avoid improper coding techniques that could impact an application's performance, functionality, or maintainability. In addition, you can enforce effective programming practices and coding styles within teams of developers to ensure code readability and functionality.", "Maintainer"="National Instruments", "Maintainer email address"="support@ni.com", "Category"="Add-Ons", "Homepage"="https://www.ni.com", "Release notes"="Refer to the NI website at https://www.ni.com/r/lvvat2021rm for installation instructions, known issues, bug fixes, compatibility information, and other important notices about this product.", "Depends"=["ni-labview-2021-vi-analyzer-toolkit-lic (>= 21.0.0)", "ni-labview-2021-x86 (>= 21.0.0)", "ni-mdfsupport (>= 21.0.0)", "ni-metauninstaller (>= 21.0.0)"], "Recommends"=[], "Suggests"=[], "Conflicts"=[], "Provides"=["143ec0b7-6e7a-4cd2-aa4b-9044162f847c (= 21.00.49154)", "ni-labview-2021-vi-analyzer-toolkit-x86 (= 21.0.0.49154-0+f2)"], "Replaces"=[], "Supplements"=["ni-labview-2021-x86 (>= 21.0.0)"], "Enhances"=[], "Product"=TRUE, "User visible"=TRUE, "Installed size (KB)"=0, "Package filesize (bytes)"=10375768, "Architecture"="windows_x64", "Agent"="wininst", "MD5Checksum"=""}}, {165, "package attributes"={"Package Name"="ni-openvino-model-optimizer", "Display name"="NI OpenVINO Model Optimizer Support for Python 3.6", "Version"="21.0.0.49315-0+f163", "Display version"="21.0.0", "Synopsis"="Provides Python 3.6 support for using the OpenVINO Toolkit Model Optimizer", "Description"="", "Maintainer"="National Instruments", "Maintainer email address"="support@ni.com", "Category"="Add-Ons", "Homepage"="https://www.ni.com", "Release notes"="", "Depends"=["ni-mdfsupport (>= 21.0.0)", "ni-metauninstaller (>= 21.0.0)"], "Recommends"=[], "Suggests"=[], "Conflicts"=["4b7c7d16-1e9f-41c3-921e-3c9685a3518b (< 0.0.1)"], "Provides"=["4b7c7d16-1e9f-41c3-921e-3c9685a3518b (= 21.00.49315)", "71ab5a9b-3040-4518-b4d8-f50a4b17a91e (= 21.00.49315)", "ni-openvino-model-optimizer (= 21.0.0.49315-0+f163)"], "Replaces"=["4b7c7d16-1e9f-41c3-921e-3c9685a3518b (< 0.0.1)"], "Supplements"=[], "Enhances"=[], "Product"=FALSE, "User visible"=TRUE, "Installed size (KB)"=0, "Package filesize (bytes)"=6403120, "Architecture"="windows_x64", "Agent"="wininst", "MD5Checksum"=""}}, {201, "package attributes"={"Package Name"="ni-pxiplatformservices-runtime", "Display name"="PXI Platform Services Runtime", "Version"="21.0.0.49348-0+f196", "Display version"="21.0.0", "Synopsis"="PXI Platform Services Runtime supports NI PXI Chassis and Controllers, implements the PXI specifications, and supplies system services to other NI products.", "Description"="", "Maintainer"="National Instruments", "Maintainer email address"="support@ni.com", "Category"="Drivers", "Homepage"="https://www.ni.com", "Release notes"="", "Depends"=["ni-apal-errors (>= 21.0.0)", "ni-apxipm2 (>= 21.0.0)", "ni-controllerdriver (>= 21.0.0)", "ni-mdfsupport (>= 21.0.0)", "ni-metauninstaller (>= 21.0.0)", "ni-mru (>= 21.0.0)", "ni-msvcrt-2015 (>= 14.1.5)", "ni-mximanager (>= 21.0.0)", "ni-pal (>= 21.0.0)", "ni-pcibrd (>= 21.0.0)", "ni-pxiplatformframework (>= 21.0.0)", "ni-pxiplatformservices-expert (>= 21.0.0)", "ni-pxiplatformsoftware-errors (>= 21.0.0)", "ni-qpxi (>= 21.0.0)", "ni-roco (>= 21.0.0)", "ni-svcloc (>= 21.0.0)", "ni-sysapi (>= 21.0.0)"], "Recommends"=["ni-certificates (>= 21.0.0)"], "Suggests"=[], "Conflicts"=["a0865ca8-e3fc-4fa2-ae33-3b027dafff94 (< 17.0.0)"], "Provides"=["2e41587c-0be1-455f-8ce6-671921397484 (= 21.00.49348)", "74cd996e-746d-4a5e-b7d9-4ed5fbafcf0d (= 21.00.49348)", "a0865ca8-e3fc-4fa2-ae33-3b027dafff94 (= 21.00.49348)", "c3b27671-335d-4816-b189-3eac7e5db5e7 (= 21.00.49348)", "ni-pxiplatformservices-runtime (= 21.0.0.49348-0+f196)"], "Replaces"=["a0865ca8-e3fc-4fa2-ae33-3b027dafff94 (< 17.0.0)"], "Supplements"=[], "Enhances"=[], "Product"=FALSE, "User visible"=TRUE, "Installed size (KB)"=0, "Package filesize (bytes)"=9000854, "Architecture"="windows_x64", "Agent"="wininst", "MD5Checksum"=""}}, {204, "package attributes"={"Package Name"="ni-vision-common-resources", "Display name"="Vision Common Resources", "Version"="21.0.0.49315-0+f163", "Display version"="2021", "Synopsis"="Vision Common Resources provides support for developing and deploying applications using basic machine vision functions.", "Description"="Vision Common Resources provides support for NI Vision image management functions, Image Display controls, and image shared variables across both Windows or NI Linux Real-Time hardware. Comprehensive machine vision support is available through the Vision Development Module.", "Maintainer"="National Instruments", "Maintainer email address"="support@ni.com", "Category"="Drivers", "Homepage"="https://www.ni.com", "Release notes"="Refer to the NI website at https://www.ni.com/r/vdmreadme2021 for installation instructions, known issues, bug fixes, compatibility information, and other important notices about this product.", "Depends"=["ni-mdfsupport (>= 21.0.0)", "ni-metauninstaller (>= 21.0.0)", "ni-msvcrt-2015 (>= 14.1.5)", "ni-openvino-inference-engine (>= 21.0.0)", "ni-rpc (>= 21.0.0)", "ni-tensorflow (>= 21.0.0)", "ni-vision-errors (>= 21.0.0)"], "Recommends"=["ni-vision-common-labview-2018-support (>= 21.0.0)", "ni-vision-common-labview-2018-support-x86 (>= 21.0.0)", "ni-vision-common-labview-2019-support (>= 21.0.0)", "ni-vision-common-labview-2019-support-x86 (>= 21.0.0)", "ni-vision-common-labview-2020-support (>= 21.0.0)", "ni-vision-common-labview-2020-support-x86 (>= 21.0.0)", "ni-vision-common-labview-2021-support (>= 21.0.0)", "ni-vision-common-labview-2021-support-x86 (>= 21.0.0)", "ni-vision-common-resources-21.0.0-realtime-bin (>= 21.0.0)"], "Suggests"=["ni-linux-rt-system-image-21.0.0 (>= 21.0.0)"], "Conflicts"=["409befa9-eb3e-472f-ad77-271a4a1d5927 (< 17.49.0)"], "Provides"=["409befa9-eb3e-472f-ad77-271a4a1d5927 (= 21.00.49315)", "7f4475d6-4602-47c8-a5f0-c896e5ba80f6 (= 21.00.49315)", "ni-vision-common-resources (= 21.0.0.49315-0+f163)"], "Replaces"=["409befa9-eb3e-472f-ad77-271a4a1d5927 (< 17.49.0)"], "Supplements"=[], "Enhances"=[], "Product"=TRUE, "User visible"=TRUE, "Installed size (KB)"=0, "Package filesize (bytes)"=29024130, "Architecture"="windows_x64", "Agent"="wininst", "MD5Checksum"=""}}, {205, "package attributes"={"Package Name"="ni-vision-common-labview-2021-support-x86", "Display name"="NI Vision Common Support for LabVIEW 2021 (32-bit)", "Version"="21.0.0.49316-0+f164", "Display version"="21.0.0", "Synopsis"="Provides LabVIEW 2021 (32-bit) Common support for NI Vision.", "Description"="", "Maintainer"="National Instruments", "Maintainer email address"="support@ni.com", "Category"="Add-Ons", "Homepage"="https://www.ni.com", "Release notes"="", "Depends"=["ni-labview-2021-fpga-advanced-session-resources-x86 (>= 21.0.0)", "ni-labview-2021-x86 (>= 21.0.0)", "ni-metauninstaller (>= 21.0.0)", "ni-vision-common-resources (>= 21.0.0)"], "Recommends"=[], "Suggests"=[], "Conflicts"=[], "Provides"=["ni-vision-common-labview-2021-support-x86 (= 21.0.0.49316-0+f164)"], "Replaces"=[], "Supplements"=["ni-labview-2021-x86 (>= 21.0.0)"], "Enhances"=[], "Product"=FALSE, "User visible"=TRUE, "Installed size (KB)"=0, "Package filesize (bytes)"=20096134, "Architecture"="windows_x64", "Agent"="wininst", "MD5Checksum"=""}}, {206, "package attributes"={"Package Name"="ni-vision-runtime", "Display name"="Vision Development Module Runtime", "Version"="21.0.0.49315-0+f163", "Display version"="2021", "Synopsis"="The Vision Development Module Runtime helps you run compiled code such as DLLs, libraries, and executables built using Vision Development Module software.", "Description"="The Vision Development Module (VDM) Runtime is an edition of VDM software that helps you deploy code to target hardware, but the edition does not include APIs for developing and running applications in the programming environments. The VDM Runtime includes the libraries and other files required to run machine vision applications built with VDM.", "Maintainer"="National Instruments", "Maintainer email address"="support@ni.com", "Category"="Add-Ons", "Homepage"="https://www.ni.com", "Release notes"="Refer to the NI website at https://www.ni.com/r/vdmreadme2021 for installation instructions, known issues, bug fixes, compatibility information, and other important notices about this product.", "Depends"=["ni-license-manager (>= 21.0.0)", "ni-mdfsupport (>= 21.0.0)", "ni-metauninstaller (>= 21.0.0)", "ni-mstudio-common-fx40-19.1.0-runtime (>= 19.1.0)", "ni-slcp (>= 21.0.0)", "ni-slcp-x86 (>= 21.0.0)", "ni-vision-common-resources (>= 21.0.0)"], "Recommends"=[], "Suggests"=[], "Conflicts"=["63df74e5-a5c9-11d4-814e-005004d6cdd6 (< 17.49.0)"], "Provides"=["63df74e5-a5c9-11d4-814e-005004d6cdd6 (= 21.00.49315)", "a497e263-56ae-44bd-b2b6-1497f3229135 (= 21.00.49315)", "c1ed176f-5f97-4349-90be-4b742ecc97b4 (= 21.00.49315)", "ni-vision-runtime (= 21.0.0.49315-0+f163)"], "Replaces"=["63df74e5-a5c9-11d4-814e-005004d6cdd6 (< 17.49.0)"], "Supplements"=[], "Enhances"=[], "Product"=TRUE, "User visible"=TRUE, "Installed size (KB)"=0, "Package filesize (bytes)"=1128762, "Architecture"="windows_x64", "Agent"="wininst", "MD5Checksum"=""}}, {207, "package attributes"={"Package Name"="ni-vision-full-common", "Display name"="NI Vision Common Development Support", "Version"="21.0.0.49315-0+f163", "Display version"="21.0.0", "Synopsis"="Provides shared development support for NI Vision across development environments", "Description"="", "Maintainer"="National Instruments", "Maintainer email address"="support@ni.com", "Category"="Add-Ons", "Homepage"="https://www.ni.com", "Release notes"="", "Depends"=["ni-license-manager (>= 21.0.0)", "ni-mdfsupport (>= 21.0.0)", "ni-metauninstaller (>= 21.0.0)", "ni-mstudio-common-fx40-19.1.0-development (>= 19.1.1)", "ni-vision-runtime (>= 21.0.0)"], "Recommends"=[], "Suggests"=[], "Conflicts"=["7f7bd153-832b-4e6e-a100-3f28e7bc5d80 (< 17.49.0)"], "Provides"=["7f7bd153-832b-4e6e-a100-3f28e7bc5d80 (= 21.00.49315)", "ee6868ef-1adc-42f8-b39f-61cdf9083610 (= 21.00.49315)", "ni-vision-full-common (= 21.0.0.49315-0+f163)"], "Replaces"=["7f7bd153-832b-4e6e-a100-3f28e7bc5d80 (< 17.49.0)"], "Supplements"=[], "Enhances"=[], "Product"=FALSE, "User visible"=TRUE, "Installed size (KB)"=0, "Package filesize (bytes)"=941850, "Architecture"="windows_x64", "Agent"="wininst", "MD5Checksum"=""}}, {209, "package attributes"={"Package Name"="ni-vision-assistant-app-x86", "Display name"="Vision Assistant (32-bit)", "Version"="21.0.0.49316-0+f164", "Display version"="21.0.0", "Synopsis"="Provides Vision Assistant (32-bit) Application.", "Description"="", "Maintainer"="National Instruments", "Maintainer email address"="support@ni.com", "Category"="Add-Ons", "Homepage"="https://www.ni.com", "Release notes"="", "Depends"=["ni-ceip-x86 (>= 21.0.0)", "ni-labview-2021-runtime-engine-x86 (>= 21.0.0)", "ni-license-manager (>= 21.0.0)", "ni-metauninstaller (>= 21.0.0)", "ni-msvcrt-2015 (>= 14.1.5)", "ni-vision-assistant-common (>= 21.0.0)", "ni-vision-assistant-examples-x86 (>= 21.0.0)", "ni-vision-full-common (>= 21.0.0)"], "Recommends"=[], "Suggests"=[], "Conflicts"=["4f5311cf-c7fd-4d9b-8c07-802147170128 (< 18.49.0)", "e829c668-e1bd-4a79-8820-0838961d3268 (< 18.49.0)"], "Provides"=["4f5311cf-c7fd-4d9b-8c07-802147170128 (= 21.00.49316)", "c978398d-94da-4cd7-a905-ca939dbc7a35 (= 21.00.49316)", "e829c668-e1bd-4a79-8820-0838961d3268 (= 21.00.49316)", "ni-vision-assistant-app-x86 (= 21.0.0.49316-0+f164)"], "Replaces"=["4f5311cf-c7fd-4d9b-8c07-802147170128 (< 18.49.0)", "e829c668-e1bd-4a79-8820-0838961d3268 (< 18.49.0)"], "Supplements"=[], "Enhances"=[], "Product"=FALSE, "User visible"=TRUE, "Installed size (KB)"=0, "Package filesize (bytes)"=56459424, "Architecture"="windows_x64", "Agent"="wininst", "MD5Checksum"=""}}, {212, "package attributes"={"Package Name"="ni-vision-labview-2021-support-x86", "Display name"="NI Vision Support for LabVIEW 2021 (32-bit)", "Version"="21.0.0.49316-0+f164", "Display version"="21.0.0", "Synopsis"="Provides LabVIEW 2021 (32-bit) support for NI Vision.", "Description"="", "Maintainer"="National Instruments", "Maintainer email address"="support@ni.com", "Category"="Add-Ons", "Homepage"="https://www.ni.com", "Release notes"="", "Depends"=["ni-ceip-x86 (>= 21.0.0)", "ni-labview-2021-x86 (>= 21.0.0)", "ni-metauninstaller (>= 21.0.0)", "ni-vision-common-labview-2021-support-x86 (>= 21.0.0)", "ni-vision-example-finder-support-x86 (>= 21.0.0)", "ni-vision-example-images (>= 21.0.0)", "ni-vision-full-common (>= 21.0.0)", "ni-vision-legacy (>= 21.0.0)", "ni-vision-training-interfaces (>= 21.0.0)"], "Recommends"=[], "Suggests"=[], "Conflicts"=[], "Provides"=["ni-vision-labview-2021-support-x86 (= 21.0.0.49316-0+f164)"], "Replaces"=[], "Supplements"=["ni-labview-2021-x86 (>= 21.0.0)"], "Enhances"=[], "Product"=FALSE, "User visible"=TRUE, "Installed size (KB)"=0, "Package filesize (bytes)"=16807904, "Architecture"="windows_x64", "Agent"="wininst", "MD5Checksum"=""}}, {213, "package attributes"={"Package Name"="ni-vision-assistant-labview-2021-support-x86", "Display name"="Vision Assistant Support for LabVIEW 2021 (32-bit)", "Version"="21.0.0.49316-0+f164", "Display version"="21.0.0", "Synopsis"="Provides LabVIEW 2021 (32-bit) Code Generation and Express VI support for Vision Assistant.", "Description"="", "Maintainer"="National Instruments", "Maintainer email address"="support@ni.com", "Category"="Add-Ons", "Homepage"="https://www.ni.com", "Release notes"="", "Depends"=["ni-assistant-framework-labview-2021-codegen-x86-support (>= 21.0.0)", "ni-labview-2021-x86 (>= 21.0.0)", "ni-mdfsupport (>= 21.0.0)", "ni-metauninstaller (>= 21.0.0)", "ni-vision-assistant-app-x86 (>= 21.0.0)", "ni-vision-assistant-labview-common-x86 (>= 21.0.0)", "ni-vision-labview-2021-support-x86 (>= 21.0.0)"], "Recommends"=[], "Suggests"=[], "Conflicts"=[], "Provides"=["ni-vision-assistant-labview-2021-support-x86 (= 21.0.0.49316-0+f164)"], "Replaces"=[], "Supplements"=["ni-labview-2021-x86 (>= 21.0.0)"], "Enhances"=[], "Product"=FALSE, "User visible"=TRUE, "Installed size (KB)"=0, "Package filesize (bytes)"=6127832, "Architecture"="windows_x64", "Agent"="wininst", "MD5Checksum"=""}}, {214, "package attributes"={"Package Name"="ni-vision-development-module", "Display name"="Vision Development Module", "Version"="21.0.0.49316-0+f164", "Display version"="2021", "Synopsis"="Vision Development Module provides hundreds of functions for developing and deploying machine vision applications.", "Description"="Vision Development Module (VDM) is designed to help you develop machine vision applications using LabVIEW or C/C++ and deploy those applications to Windows or NI Linux Real-Time hardware. With its comprehensive function library, you can access hundreds of image processing algorithms and machine vision functions to enhance images, check for presence, locate features, identify objects, measure parts, and more. VDM also includes the Vision Assistant, which is an algorithm engineering tool that simplifies vision system design by helping you develop algorithms for deployment on either CPUs or FPGAs.", "Maintainer"="National Instruments", "Maintainer email address"="support@ni.com", "Category"="Add-Ons", "Homepage"="https://www.ni.com", "Release notes"="Refer to the NI website at https://www.ni.com/r/vdmreadme2021 for installation instructions, known issues, bug fixes, compatibility information, and other important notices about this product.\n\nThis version supports LabVIEW NXG 5.1.", "Depends"=["ni-metauninstaller (>= 21.0.0)", "ni-update-service (>= 21.0.0)", "ni-vision-runtime (>= 21.0.0)"], "Recommends"=["ni-openvino-model-optimizer (>= 21.0.0)", "ni-vision-assistant-app (>= 21.0.0)", "ni-vision-assistant-app-x86 (>= 21.0.0)", "ni-vision-assistant-c-support (>= 21.0.0)", "ni-vision-assistant-c-support-x86 (>= 21.0.0)", "ni-vision-assistant-labview-2018-support (>= 21.0.0)", "ni-vision-assistant-labview-2018-support-x86 (>= 21.0.0)", "ni-vision-assistant-labview-2019-support (>= 21.0.0)", "ni-vision-assistant-labview-2019-support-x86 (>= 21.0.0)", "ni-vision-assistant-labview-2020-support (>= 21.0.0)", "ni-vision-assistant-labview-2020-support-x86 (>= 21.0.0)", "ni-vision-assistant-labview-2021-support (>= 21.0.0)", "ni-vision-assistant-labview-2021-support-x86 (>= 21.0.0)", "ni-vision-assistant-labview-nxg-5.0.0-support (>= 21.0.0)", "ni-vision-assistant-labview-nxg-5.0.0-support-x86 (>= 21.0.0)", "ni-vision-c-support-x86 (>= 21.0.0)", "ni-vision-common-resources-21.0.0-realtime-bin (>= 21.0.0)", "ni-vision-cvi-support-x86 (>= 21.0.0)", "ni-vision-fpga-labview-2018-x86 (>= 21.0.0)", "ni-vision-fpga-labview-2019-x86 (>= 21.0.0)", "ni-vision-fpga-labview-2020 (>= 21.0.0)", "ni-vision-fpga-labview-2020-x86 (>= 21.0.0)", "ni-vision-fpga-labview-2021 (>= 21.0.0)", "ni-vision-fpga-labview-2021-x86 (>= 21.0.0)", "ni-vision-full-common (>= 21.0.0)", "ni-vision-labview-2018-support (>= 21.0.0)", "ni-vision-labview-2018-support-x86 (>= 21.0.0)", "ni-vision-labview-2019-support (>= 21.0.0)", "ni-vision-labview-2019-support-x86 (>= 21.0.0)", "ni-vision-labview-2020-support (>= 21.0.0)", "ni-vision-labview-2020-support-x86 (>= 21.0.0)", "ni-vision-labview-2021-support (>= 21.0.0)", "ni-vision-labview-2021-support-x86 (>= 21.0.0)", "ni-vision-labview-nxg-5.0.0-rte-support (>= 21.0.0)", "ni-vision-labview-nxg-5.0.0-support (>= 21.0.0)"], "Suggests"=["ni-linux-rt-system-image-21.0.0 (>= 21.0.0)", "ni-max (>= 21.0.0)"], "Conflicts"=["261ea00d-33df-42bd-b4c6-3a47a64289f8 (< 0.0.1)"], "Provides"=["261ea00d-33df-42bd-b4c6-3a47a64289f8 (= 21.00.49316)", "ni-vision-development-module (= 21.0.0.49316-0+f164)"], "Replaces"=["261ea00d-33df-42bd-b4c6-3a47a64289f8 (< 0.0.1)"], "Supplements"=[], "Enhances"=[], "Product"=TRUE, "User visible"=TRUE, "Installed size (KB)"=0, "Package filesize (bytes)"=380506, "Architecture"="windows_x64", "Agent"="wininst", "MD5Checksum"=""}}, {217, "package attributes"={"Package Name"="ni-gigevision", "Display name"="NI GigE Vision Driver", "Version"="21.0.0.49308-0+f156", "Display version"="21.0.0", "Synopsis"="Optimized GigE Vision driver supporting Intel Pro 1000 Network Interface Cards and NI 8237 cards.", "Description"="", "Maintainer"="National Instruments", "Maintainer email address"="support@ni.com", "Category"="Drivers", "Homepage"="https://www.ni.com", "Release notes"="", "Depends"=["ni-mdfsupport (>= 21.0.0)", "ni-metauninstaller (>= 21.0.0)", "ni-msiproperties (>= 21.0.0)", "ni-pal (>= 21.0.0)"], "Recommends"=["ni-certificates (>= 21.0.0)"], "Suggests"=[], "Conflicts"=["05544a20-4a6f-4ef3-b202-cfe6c5e6041c (< 17.49.0)"], "Provides"=["05544a20-4a6f-4ef3-b202-cfe6c5e6041c (= 21.00.49308)", "1051d066-b795-40e9-a1b7-1bb215033dfa (= 21.00.49308)", "ni-gigevision (= 21.0.0.49308-0+f156)"], "Replaces"=["05544a20-4a6f-4ef3-b202-cfe6c5e6041c (< 17.49.0)"], "Supplements"=[], "Enhances"=[], "Product"=FALSE, "User visible"=TRUE, "Installed size (KB)"=0, "Package filesize (bytes)"=1493584, "Architecture"="windows_x64", "Agent"="wininst", "MD5Checksum"=""}}, {233, "package attributes"={"Package Name"="ni-serial-runtime", "Display name"="NI-Serial Runtime", "Version"="20.0.0.49152-0+f0", "Display version"="20.0.0", "Synopsis"="NI-Serial support for National Instruments RS-232 and RS-485 Hardware.", "Description"="", "Maintainer"="National Instruments", "Maintainer email address"="support@ni.com", "Category"="Drivers", "Homepage"="http://www.ni.com", "Release notes"="", "Depends"=["ni-apal-errors (>= 19.0.0)", "ni-apxipm (>= 19.0.0)", "ni-mdfsupport (>= 20.0.0)", "ni-metauninstaller (>= 20.0.0)", "ni-msvcrt-2008 (>= 9.1.1)", "ni-msvcrt-2015 (>= 14.1.5)", "ni-mxs (>= 20.0.0)", "ni-qpxi (>= 20.0.0)", "ni-sysapi (>= 20.0.0)"], "Recommends"=["ni-certificates (>= 2.0.2)"], "Suggests"=[], "Conflicts"=["01d82f43-b48d-46ff-8601-fc4faae20f41 (< 17.0.0)"], "Provides"=["01d82f43-b48d-46ff-8601-fc4faae20f41 (= 20.00.49152)", "664a2b91-5e36-4102-ad42-e1dd3d61c77b (= 20.00.49152)", "ni-visa-optional-runtime (= 20.00.49152)", "ni-serial-runtime (= 20.0.0.49152-0+f0)"], "Replaces"=["01d82f43-b48d-46ff-8601-fc4faae20f41 (< 17.0.0)"], "Supplements"=[], "Enhances"=[], "Product"=FALSE, "User visible"=TRUE, "Installed size (KB)"=0, "Package filesize (bytes)"=3318370, "Architecture"="windows_all", "Agent"="wininst", "MD5Checksum"=""}}, {236, "package attributes"={"Package Name"="ni-imaq-runtime", "Display name"="NI-IMAQ Runtime", "Version"="21.0.0.49311-0+f159", "Display version"="21.0.0", "Synopsis"="NI-IMAQ provides support for acquiring, displaying, and saving images from parallel digital and Camera Link devices.", "Description"="", "Maintainer"="National Instruments", "Maintainer email address"="support@ni.com", "Category"="Drivers", "Homepage"="https://www.ni.com", "Release notes"="", "Depends"=["ni-imaq-expert (>= 21.0.0)", "ni-mdfsupport (>= 21.0.0)", "ni-metauninstaller (>= 21.0.0)", "ni-msiproperties (>= 21.0.0)", "ni-msvcrt-2015 (>= 14.1.5)", "ni-pal (>= 21.0.0)", "ni-pxiplatformframework (>= 21.0.0)", "ni-pxiplatformservices-runtime (>= 21.0.0)", "ni-vas-coinstaller (>= 21.0.0)", "ni-vas-errors (>= 21.0.0)", "ni-vision-common-resources (>= 21.0.0)"], "Recommends"=["ni-certificates (>= 21.0.0)"], "Suggests"=[], "Conflicts"=["a1a903c1-6270-11d4-8133-005004d6cdd6 (< 17.49.0)"], "Provides"=["497b8a53-0198-43e7-a361-d3d3b41267c9 (= 21.00.49311)", "a1a903c1-6270-11d4-8133-005004d6cdd6 (= 21.00.49311)", "ni-imaq-runtime (= 21.0.0.49311-0+f159)"], "Replaces"=["a1a903c1-6270-11d4-8133-005004d6cdd6 (< 17.49.0)"], "Supplements"=[], "Enhances"=[], "Product"=FALSE, "User visible"=TRUE, "Installed size (KB)"=0, "Package filesize (bytes)"=10420554, "Architecture"="windows_x64", "Agent"="wininst", "MD5Checksum"=""}}, {237, "package attributes"={"Package Name"="ni-imaq-config", "Display name"="NI Vision Acquisition Software Configuration Support", "Version"="21.0.0.49311-0+f159", "Display version"="21.0.0", "Synopsis"="Provides support for configuring cameras and Camera Link image acquisition devices via Measurement & Automation Explorer (MAX). Refer to the Vision Acquisition Software readme on ni.com/manuals for a full list of supported hardware.", "Description"="", "Maintainer"="National Instruments", "Maintainer email address"="support@ni.com", "Category"="Drivers", "Homepage"="https://www.ni.com", "Release notes"="", "Depends"=["ni-imaq-camera-files (>= 21.0.0)", "ni-imaq-config-client (>= 21.0.0)", "ni-labview-2020-runtime-engine-x86 (>= 20.1.0)", "ni-max (>= 21.0.0)", "ni-mdfsupport (>= 21.0.0)", "ni-mesa (>= 17.1.1)", "ni-metauninstaller (>= 21.0.0)", "ni-mstudio-cw-ui (>= 8.6.8)", "ni-msvcrt-2015 (>= 14.1.5)"], "Recommends"=[], "Suggests"=[], "Conflicts"=["1a86bcc0-3fee-4cc7-96d8-cdec14d6ed8c (< 17.49.0)", "93b90cdf-a4a3-4ee5-a063-19c0ff0602c5 (< 17.49.0)"], "Provides"=["93b90cdf-a4a3-4ee5-a063-19c0ff0602c5 (= 21.00.49311)", "f7279756-89cb-484e-b59c-f9ec4ac4404b (= 21.00.49311)", "ni-imaq-config (= 21.0.0.49311-0+f159)"], "Replaces"=["78c4d7cc-e93e-4c8f-92d2-39821cdf9854 (< 17.49.0)", "93b90cdf-a4a3-4ee5-a063-19c0ff0602c5 (< 17.49.0)"], "Supplements"=[], "Enhances"=[], "Product"=FALSE, "User visible"=TRUE, "Installed size (KB)"=0, "Package filesize (bytes)"=6864094, "Architecture"="windows_x64", "Agent"="wininst", "MD5Checksum"=""}}, {238, "package attributes"={"Package Name"="ni-serial-config", "Display name"="NI-Serial Configuration", "Version"="20.0.0.49152-0+f0", "Display version"="20.0.0", "Synopsis"="Support for configuring NI-Serial hardware settings in Measurement & Automation Explorer.", "Description"="", "Maintainer"="National Instruments", "Maintainer email address"="support@ni.com", "Category"="Drivers", "Homepage"="http://www.ni.com", "Release notes"="", "Depends"=["ni-iotrace (>= 20.0.0)", "ni-launcher (>= 20.0.0)", "ni-max (>= 20.0.0)", "ni-mdfsupport (>= 20.0.0)", "ni-metauninstaller (>= 20.0.0)", "ni-msvcrt-2008 (>= 9.1.1)", "ni-msvcrt-2015 (>= 14.1.5)", "ni-serial-runtime (>= 20.0.0)", "ni-visa-configuration (>= 20.0.0)", "ni-visa-runtime (>= 20.0.0)"], "Recommends"=[], "Suggests"=[], "Conflicts"=["795891ec-c372-47d5-acdc-cb64f07783da (< 17.0.0)"], "Provides"=["795891ec-c372-47d5-acdc-cb64f07783da (= 20.00.49152)", "ni-serial-config (= 20.0.0.49152-0+f0)"], "Replaces"=["795891ec-c372-47d5-acdc-cb64f07783da (< 17.0.0)"], "Supplements"=[], "Enhances"=[], "Product"=FALSE, "User visible"=TRUE, "Installed size (KB)"=0, "Package filesize (bytes)"=2186044, "Architecture"="windows_all", "Agent"="wininst", "MD5Checksum"=""}}, {239, "package attributes"={"Package Name"="ni-imaqdx-runtime", "Display name"="NI-IMAQdx Runtime", "Version"="21.0.0.49311-0+f159", "Display version"="21.0.0", "Synopsis"="Runtime components required to deploy image acquisition applications.", "Description"="", "Maintainer"="National Instruments", "Maintainer email address"="support@ni.com", "Category"="Drivers", "Homepage"="https://www.ni.com", "Release notes"="", "Depends"=["ni-gvsp (>= 21.0.0)", "ni-imaq-config-client (>= 21.0.0)", "ni-imaq-runtime (>= 21.0.0)", "ni-imaqdx-expert (>= 21.0.0)", "ni-imaqdx-isc178x-win (>= 21.0.0)", "ni-license-manager (>= 21.0.0)", "ni-mdfsupport (>= 21.0.0)", "ni-mdnsresponder (>= 21.0.0)", "ni-metauninstaller (>= 21.0.0)", "ni-msiproperties (>= 21.0.0)", "ni-mstudio-common-fx40-19.0.0-runtime (>= 19.0.0)", "ni-msvcrt-2015 (>= 14.1.5)", "ni-pal (>= 21.0.0)", "ni-slcp (>= 21.0.0)", "ni-slcp-x86 (>= 21.0.0)", "ni-usb3vision (>= 21.0.0)", "ni-vas-coinstaller (>= 21.0.0)", "ni-vas-errors (>= 21.0.0)", "ni-vision-common-resources (>= 21.0.0)"], "Recommends"=["ni-certificates (>= 21.0.0)", "ni-gvsp-gigevision (>= 17.5.0)"], "Suggests"=[], "Conflicts"=["3d104ab3-ce10-43c0-b647-07600754072c (< 17.49.0)"], "Provides"=["05b883f6-ebf8-428c-bdd3-9a72bb9f37e9 (= 21.00.49311)", "3d104ab3-ce10-43c0-b647-07600754072c (= 21.00.49311)", "ni-imaqdx-runtime (= 21.0.0.49311-0+f159)"], "Replaces"=["3d104ab3-ce10-43c0-b647-07600754072c (< 17.49.0)"], "Supplements"=[], "Enhances"=[], "Product"=FALSE, "User visible"=TRUE, "Installed size (KB)"=0, "Package filesize (bytes)"=4658872, "Architecture"="windows_x64", "Agent"="wininst", "MD5Checksum"=""}}, {241, "package attributes"={"Package Name"="ni-imaqdx-development-support", "Display name"="NI-IMAQdx Common Development Support", "Version"="21.0.0.49311-0+f159", "Display version"="21.0.0", "Synopsis"="Provides shared development support for NI-IMAQdx across development environments", "Description"="", "Maintainer"="National Instruments", "Maintainer email address"="support@ni.com", "Category"="Drivers", "Homepage"="https://www.ni.com", "Release notes"="", "Depends"=["ni-cvs-firmware (>= 21.0.0)", "ni-cvs-max-provider (>= 21.0.0)", "ni-imaq-config (>= 21.0.0)", "ni-mdfsupport (>= 21.0.0)", "ni-metauninstaller (>= 21.0.0)", "ni-mstudio-common-fx40-19.0.0-development (>= 19.0.0)", "ni-serial-config (>= 20.0.0)", "ni-smartcamera-max-provider (>= 21.0.0)"], "Recommends"=[], "Suggests"=[], "Conflicts"=["870fd426-33dc-43b4-8ec8-22d38cb92015 (< 18.99.0)"], "Provides"=["4c079442-2937-4bd9-8f1c-0dac19f8af5d (= 21.00.49311)", "870fd426-33dc-43b4-8ec8-22d38cb92015 (= 21.00.49311)", "ni-imaqdx-development-support (= 21.0.0.49311-0+f159)"], "Replaces"=["870fd426-33dc-43b4-8ec8-22d38cb92015 (< 18.99.0)"], "Supplements"=[], "Enhances"=[], "Product"=FALSE, "User visible"=TRUE, "Installed size (KB)"=0, "Package filesize (bytes)"=1635834, "Architecture"="windows_x64", "Agent"="wininst", "MD5Checksum"=""}}, {242, "package attributes"={"Package Name"="ni-gvsp-gigevision", "Display name"="NI-IMAQdx High-Performance GigE Vision Driver", "Version"="21.0.0.49311-0+f159", "Display version"="21.0.0", "Synopsis"="Optimized GigE Vision driver supporting Intel Pro 1000 Network Interface Cards.", "Description"="", "Maintainer"="National Instruments", "Maintainer email address"="support@ni.com", "Category"="Drivers", "Homepage"="https://www.ni.com", "Release notes"="", "Depends"=["ni-apal-errors (>= 21.0.0)", "ni-gigevision (>= 21.0.0)", "ni-imaqdx-runtime (>= 21.0.0)", "ni-mdfsupport (>= 21.0.0)", "ni-metauninstaller (>= 21.0.0)", "ni-msiproperties (>= 21.0.0)", "ni-msvcrt-2015 (>= 14.1.5)"], "Recommends"=["ni-certificates (>= 21.0.0)"], "Suggests"=[], "Conflicts"=["b2eea39b-669f-4fe0-b559-ff4bb9b21229 (< 17.49.0)"], "Provides"=["b2eea39b-669f-4fe0-b559-ff4bb9b21229 (= 21.00.49311)", "e85b1f5a-0b0e-43fe-9d85-41fdb014147b (= 21.00.49311)", "vision-gigevision-optional-runtime", "ni-gvsp-gigevision (= 21.0.0.49311-0+f159)"], "Replaces"=["b2eea39b-669f-4fe0-b559-ff4bb9b21229 (< 17.49.0)"], "Supplements"=[], "Enhances"=[], "Product"=FALSE, "User visible"=TRUE, "Installed size (KB)"=0, "Package filesize (bytes)"=1690534, "Architecture"="windows_x64", "Agent"="wininst", "MD5Checksum"=""}}, {243, "package attributes"={"Package Name"="ni-imaq-labview-2021-support-x86", "Display name"="NI-IMAQ Support for LabVIEW 2021 (32-bit)", "Version"="21.0.0.49313-0+f161", "Display version"="21.0.0", "Synopsis"="Provides API, documentation, and examples for using NI-IMAQ devices within LabVIEW 2021 (32-bit)", "Description"="", "Maintainer"="National Instruments", "Maintainer email address"="support@ni.com", "Category"="Drivers", "Homepage"="https://www.ni.com", "Release notes"="", "Depends"=["ni-ceip-x86 (>= 21.0.0)", "ni-imaq-development-support (>= 21.0.0)", "ni-imaq-runtime (>= 21.0.0)", "ni-labview-2021-x86 (>= 21.0.0)", "ni-mdfsupport (>= 21.0.0)", "ni-metauninstaller (>= 21.0.0)", "ni-syscfg-labview-2021-support-x86 (>= 21.0.0)", "ni-vision-acquisition-express-labview-2021-x86 (>= 21.0.0)", "ni-vision-acquisition-labview-2021-provider (>= 21.0.0)", "ni-vision-common-labview-2021-support-x86 (>= 21.0.0)", "ni-vision-example-finder-support-x86 (>= 21.0.0)"], "Recommends"=[], "Suggests"=[], "Conflicts"=[], "Provides"=["ni-imaq-labview-2021-support-x86 (= 21.0.0.49313-0+f161)"], "Replaces"=[], "Supplements"=["ni-labview-2021-x86 (>= 21.0.0)"], "Enhances"=[], "Product"=FALSE, "User visible"=TRUE, "Installed size (KB)"=0, "Package filesize (bytes)"=2905668, "Architecture"="windows_x64", "Agent"="wininst", "MD5Checksum"=""}}, {244, "package attributes"={"Package Name"="ni-imaqdx-labview-2021-support-x86", "Display name"="NI-IMAQdx Support for LabVIEW 2021 (32-bit)", "Version"="21.0.0.49313-0+f161", "Display version"="21.0.0", "Synopsis"="Provides API, documentation, and examples for using NI-IMAQdx devices within LabVIEW 2021 (32-bit)", "Description"="", "Maintainer"="National Instruments", "Maintainer email address"="support@ni.com", "Category"="Drivers", "Homepage"="https://www.ni.com", "Release notes"="", "Depends"=["ni-ceip-x86 (>= 21.0.0)", "ni-imaqdx-development-support (>= 21.0.0)", "ni-imaqdx-runtime (>= 21.0.0)", "ni-labview-2021-x86 (>= 21.0.0)", "ni-mdfsupport (>= 21.0.0)", "ni-metauninstaller (>= 21.0.0)", "ni-rio-fpga-driver (>= 21.0.0)", "ni-syscfg-labview-2021-support-x86 (>= 21.0.0)", "ni-vision-acquisition-express-labview-2021-x86 (>= 21.0.0)", "ni-vision-acquisition-labview-2021-provider (>= 21.0.0)", "ni-vision-common-labview-2021-support-x86 (>= 21.0.0)", "ni-vision-example-finder-support-x86 (>= 21.0.0)"], "Recommends"=[], "Suggests"=[], "Conflicts"=[], "Provides"=["ni-imaqdx-labview-2021-support-x86 (= 21.0.0.49313-0+f161)"], "Replaces"=[], "Supplements"=["ni-labview-2021-x86 (>= 21.0.0)"], "Enhances"=[], "Product"=FALSE, "User visible"=TRUE, "Installed size (KB)"=0, "Package filesize (bytes)"=3055952, "Architecture"="windows_x64", "Agent"="wininst", "MD5Checksum"=""}}, {245, "package attributes"={"Package Name"="ni-imaq", "Display name"="NI-IMAQ", "Version"="21.0.0.49313-0+f161", "Display version"="21.0.0", "Synopsis"="NI-IMAQ is driver software for acquiring, displaying, and saving images using Camera Link Frame Grabber Devices.", "Description"="NI-IMAQ is driver software for acquiring images from Camera Link Frame Grabber Devices. You can use this driver in conjunction with the Vision Development Module or Vision Builder for Automated Inspection to develop and deploy machine vision applications.", "Maintainer"="National Instruments", "Maintainer email address"="support@ni.com", "Category"="Drivers", "Homepage"="https://www.ni.com", "Release notes"="Refer to the NI website at https://www.ni.com/r/vasreadme210 for installation instructions, known issues, bug fixes, compatibility information, and other important notices about this product.", "Depends"=["ni-imaq-runtime (>= 21.0.0)", "ni-metauninstaller (>= 21.0.0)", "ni-msiproperties (>= 21.0.0)", "ni-update-service (>= 21.0.0)"], "Recommends"=["ni-imaq-c-support (>= 21.0.0)", "ni-imaq-config (>= 21.0.0)", "ni-imaq-cvi-support (>= 21.0.0)", "ni-imaq-labview-2018-support (>= 21.0.0)", "ni-imaq-labview-2018-support-x86 (>= 21.0.0)", "ni-imaq-labview-2019-support (>= 21.0.0)", "ni-imaq-labview-2019-support-x86 (>= 21.0.0)", "ni-imaq-labview-2020-support (>= 21.0.0)", "ni-imaq-labview-2020-support-x86 (>= 21.0.0)", "ni-imaq-labview-2021-support (>= 21.0.0)", "ni-imaq-labview-2021-support-x86 (>= 21.0.0)"], "Suggests"=[], "Conflicts"=["2daef249-ffc5-4da0-b89a-c45aa3c8a8c1 (< 0.0.1)"], "Provides"=["2daef249-ffc5-4da0-b89a-c45aa3c8a8c1 (= 21.00.49313)", "ni-imaq (= 21.0.0.49313-0+f161)"], "Replaces"=["2daef249-ffc5-4da0-b89a-c45aa3c8a8c1 (< 0.0.1)"], "Supplements"=[], "Enhances"=[], "Product"=TRUE, "User visible"=TRUE, "Installed size (KB)"=0, "Package filesize (bytes)"=374418, "Architecture"="windows_x64", "Agent"="wininst", "MD5Checksum"=""}}, {246, "package attributes"={"Package Name"="ni-imaqdx", "Display name"="NI-IMAQdx", "Version"="21.0.0.49313-0+f161", "Display version"="21.0.0", "Synopsis"="NI-IMAQdx supports acquiring, displaying, and saving images from cameras.", "Description"="NI-IMAQdx is driver software for acquiring images from Camera Link, USB3 Vision, GigE Vision cameras, DirectShow-compliant USB devices, and Smart Cameras. You can use this driver in conjunction with the Vision Development Module or Vision Builder for Automated Inspection to develop and deploy machine vision applications.", "Maintainer"="National Instruments", "Maintainer email address"="support@ni.com", "Category"="Drivers", "Homepage"="https://www.ni.com", "Release notes"="Refer to the NI website at https://www.ni.com/r/vasreadme210 for installation instructions, known issues, bug fixes, compatibility information, and other important notices about this product.\n\nThis version supports LabVIEW NXG 5.1.", "Depends"=["ni-imaqdx-runtime (>= 21.0.0)", "ni-metauninstaller (>= 21.0.0)", "ni-msiproperties (>= 21.0.0)", "ni-update-service (>= 21.0.0)"], "Recommends"=["ni-gvsp-gigevision (>= 21.0.0)", "ni-imaq-config (>= 21.0.0)", "ni-imaqdx-21.0.0-realtime-bin (>= 21.0.0)", "ni-imaqdx-c-support (>= 21.0.0)", "ni-imaqdx-cvi-support (>= 21.0.0)", "ni-imaqdx-development-support (>= 21.0.0)", "ni-imaqdx-labview-2018-support (>= 21.0.0)", "ni-imaqdx-labview-2018-support-x86 (>= 21.0.0)", "ni-imaqdx-labview-2019-support (>= 21.0.0)", "ni-imaqdx-labview-2019-support-x86 (>= 21.0.0)", "ni-imaqdx-labview-2020-support (>= 21.0.0)", "ni-imaqdx-labview-2020-support-x86 (>= 21.0.0)", "ni-imaqdx-labview-2021-support (>= 21.0.0)", "ni-imaqdx-labview-2021-support-x86 (>= 21.0.0)", "ni-imaqdx-labview-nxg-5.0.0-rte-support (>= 21.0.0)", "ni-imaqdx-labview-nxg-5.0.0-support (>= 21.0.0)"], "Suggests"=["ni-linux-rt-system-image-21.0.0 (>= 21.0.0)"], "Conflicts"=["d95c0954-bbb0-44cb-938a-ad4815937902 (< 0.0.1)"], "Provides"=["d95c0954-bbb0-44cb-938a-ad4815937902 (= 21.00.49313)", "ni-imaqdx (= 21.0.0.49313-0+f161)"], "Replaces"=["d95c0954-bbb0-44cb-938a-ad4815937902 (< 0.0.1)"], "Supplements"=[], "Enhances"=[], "Product"=TRUE, "User visible"=TRUE, "Installed size (KB)"=0, "Package filesize (bytes)"=380040, "Architecture"="windows_x64", "Agent"="wininst", "MD5Checksum"=""}}, {247, "package attributes"={"Package Name"="ni-labview-2017-runtime-engine-x86", "Display name"="NI LabVIEW 2017 Runtime", "Version"="17.5.1.49152-0+f0", "Display version"="17.5.1", "Synopsis"="NI LabVIEW 2017 Runtime provides libraries and other files necessary to execute LabVIEW 2017-built applications and shared libraries. Includes NI Reports, 3D graph support, and a browser plug-in that enables clients to view and control front panels remotely using a browser.", "Description"="", "Maintainer"="National Instruments", "Maintainer email address"="support@ni.com", "Category"="Programming Environments", "Homepage"="http://www.ni.com", "Release notes"="", "Depends"=["ni-activex-container (>=17.1.0)", " ni-curl (>=18.0.0)", " ni-cvi-low-level-driver (>=17.0.0)", " ni-deployment-framework-x86 (>=18.0.0)", " ni-error-report-x86 (>=18.0.0)", " ni-error-reporting-interface (>=18.0.0)", " ni-labview-2017-runtime-engine-resource (>=17.1.0)", " ni-logos (>=18.0.0)", " ni-lv-web-server-labview-2017-runtime-engine-x86-support (>=17.0.1)", " ni-mdfsupport (>=18.0.0)", " ni-mdnsresponder (>=17.0.0)", " ni-metauninstaller (>=18.0.0)", " ni-mkl-2017 (>=17.0.0)", " ni-msiproperties (>=18.0.0)", " ni-mstudio-cw3dgraph (>=8.6.3)", " ni-msvcrt-2008 (>=9.1.0)", " ni-msvcrt-2010 (>=10.1.0)", " ni-msvcrt-2015 (>=14.1.4)", " ni-realtime-nbfifo-labview-2017-support (>=17.0.0)", " ni-svcloc (>=18.0.0)", " ni-systemlogging-utils (>=18.0.0)", " ni-tdms (>=18.0.0)", " ni-traceengine (>=18.0.0)", ""], "Recommends"=[], "Suggests"=[], "Conflicts"=[], "Provides"=["1f26181b-7add-482f-be80-20b5023c2580 (=17.51.49152)", " 620dbae1-b159-4204-8186-0813c8a6434c (=17.51.49152)", ""], "Replaces"=[], "Supplements"=[], "Enhances"=[], "Product"=TRUE, "User visible"=TRUE, "Installed size (KB)"=0, "Package filesize (bytes)"=0, "Architecture"="windows_x64", "Agent"="wininst", "MD5Checksum"=""}}, {251, "package attributes"={"Package Name"="ni-labview-dett-labview-2021-support-x86", "Display name"="LabVIEW Desktop Execution Trace Toolkit Support for LabVIEW 2021", "Version"="21.0.0.49152-0+f0", "Display version"="2021", "Synopsis"="This installs the LabVIEW Desktop Execution Trace Toolkit support files for LabVIEW 2021.", "Description"="", "Maintainer"="National Instruments", "Maintainer email address"="support@ni.com", "Category"="Add-Ons", "Homepage"="https://www.ni.com", "Release notes"="", "Depends"=["ni-labview-2021-helpchm (>= 21.0.0)", "ni-labview-2021-x86 (>= 21.0.0)", "ni-labview-dett (>= 21.0.0)", "ni-mdfsupport (>= 21.0.0)", "ni-metauninstaller (>= 21.0.0)"], "Recommends"=[], "Suggests"=[], "Conflicts"=["6a00423d-5b21-4ce1-bc64-aadece149d7d (< 19.0.0)"], "Provides"=["6a00423d-5b21-4ce1-bc64-aadece149d7d (= 21.00.49152)", "ni-labview-dett-labview-2021-support-x86 (= 21.0.0.49152-0+f0)"], "Replaces"=["6a00423d-5b21-4ce1-bc64-aadece149d7d (< 19.0.0)"], "Supplements"=["ni-labview-2021-x86 (>= 21.0.0)"], "Enhances"=[], "Product"=FALSE, "User visible"=TRUE, "Installed size (KB)"=0, "Package filesize (bytes)"=750612, "Architecture"="windows_x64", "Agent"="wininst", "MD5Checksum"=""}}, {267, "package attributes"={"Package Name"="e2930e04-b1e7-49c2-9d5d-d9d8d208a4ba", "Display name"="Command", "Version"="1.1.0", "Display version"="", "Synopsis"="This is built using NI software.", "Description"="", "Maintainer"="Agilent Technologies Inc.", "Maintainer email address"="", "Category"="Other Software", "Homepage"="", "Release notes"="", "Depends"=["fcf64b73-b7d4-4971-8f11-24baf7cc3e6c (>= 17.0.59)", " 620dbae1-b159-4204-8186-0813c8a6434c (>= 17.02.49152)", " 578b3422-eae6-428c-a17a-7549578fe2c1 (>= 8.75.49152)"], "Recommends"=[], "Suggests"=[], "Conflicts"=[], "Provides"=["e2930e04-b1e7-49c2-9d5d-d9d8d208a4ba (= 1.1.0)"], "Replaces"=[], "Supplements"=[], "Enhances"=[], "Product"=FALSE, "User visible"=TRUE, "Installed size (KB)"=0, "Package filesize (bytes)"=0, "Architecture"="windows_all", "Agent"="wininst", "MD5Checksum"=""}}, {270, "package attributes"={"Package Name"="ff14843e-cd62-44fd-8b3f-2b6e418fbbd3", "Display name"="NI 1588-2008 Network Management 17.0.0 LabVIEW API Core", "Version"="17.0.26", "Display version"="", "Synopsis"="This is required for NI software.", "Description"="", "Maintainer"="National Instruments", "Maintainer email address"="support@ni.com", "Category"="Other Software", "Homepage"="", "Release notes"="", "Depends"=["5b0cb826-e499-4e6b-94f0-75b6327ed934", " be400a3d-e9d6-48d9-af14-337722a11d40", " 5b0cb826-e499-4e6b-94f0-75b6327ed934", " be400a3d-e9d6-48d9-af14-337722a11d40", " 47022337-36f3-4ac7-9021-e190df115288 (>= 17.00.32772)", " aa333f93-319c-4ecc-8388-d40d5f7582f4 (>= 17.0.20)"], "Recommends"=[], "Suggests"=[], "Conflicts"=[], "Provides"=["cce3dc38-7a88-47e1-8466-ccc2ce49c049 (= 17.00)", " ff14843e-cd62-44fd-8b3f-2b6e418fbbd3 (= 17.0.26)"], "Replaces"=[], "Supplements"=[], "Enhances"=[], "Product"=FALSE, "User visible"=TRUE, "Installed size (KB)"=0, "Package filesize (bytes)"=0, "Architecture"="windows_all", "Agent"="wininst", "MD5Checksum"=""}}, {282, "package attributes"={"Package Name"="5200154e-c313-4829-96aa-04adb772c374", "Display name"="NI LabVIEW 2013 SP1 (32-bit)", "Version"="13.1.101", "Display version"="", "Synopsis"="This is required for NI software.", "Description"="", "Maintainer"="National Instruments", "Maintainer email address"="support@ni.com", "Category"="LabVIEW", "Homepage"="", "Release notes"="", "Depends"=["5b0cb826-e499-4e6b-94f0-75b6327ed934", " be400a3d-e9d6-48d9-af14-337722a11d40", " 5b0cb826-e499-4e6b-94f0-75b6327ed934", " 81a7e53e-9524-41ce-90d3-7dd3d90b6c58 (>= 5.1.227)", " 9ac94877-534e-480a-8770-90007dcdd5fb (>= 1.0.1)", " b07bce56-3625-40e3-8d46-5e6ea0fd65c8 (>= 13.1.99)", " 1670a9fc-09ea-49f9-9f9e-ca88675aba17 (>= 13.1.99)", " 8f101784-9b55-4e67-92c8-0e845f12f3ab (>= 9.75.49152)", " 9b45d5a6-3453-459c-8b9f-3a2253295364 (>= 1.0.14.0)", " 6119c43c-b47a-4f5d-bf64-977e510d0761 (>= 9.0.6.0)", " 16188476-79e6-4579-b97a-d01daf48554f (>= 13.1.99)", " ea05dcf9-f239-4387-8904-04d678031f6b (>= 13.0.13)", " ab3599b6-97d9-4fe7-9e0d-87528fd8e8a7 (>= 5.60.49152)", " be400a3d-e9d6-48d9-af14-337722a11d40", " 5e4a4ce3-4d06-11d4-8b22-006008c16337 (>= 5.5.293)", " d1edc484-7b17-11d7-83ce-00c0f03ebebe (>= 2.1.05374)", " d41b7da9-c5a7-41b5-8420-4cd6c925ef58 (>= 13.0.296)", " eb7a3c81-1c0f-4495-8ce5-0a427e4e6285 (>= 2.7.297)", " e3edda5c-9326-44cb-8cc1-567e6b7a745f (>= 3.30.24)", " a298c267-3ce7-4b95-9d8b-bcb6672bc7b9 (>= 2.70.346)", " 11d580a9-caa9-4fae-acce-008751a7ae9f (>= 2.30.65)", " f8eb8d56-5463-4111-867f-16fe80585c0a (>= 13.1.99)", " 63b491e3-07d0-4df4-80d4-3e750eb6770b (>= 13.1.99)", " e5b722cc-4a62-4556-9bbc-2140d8c08c00 (>= 13.1.99)", " 5b0cb826-e499-4e6b-94f0-75b6327ed934", " 14627488-7864-4983-9279-21a2eda32254 (>= 13.1.99)", " e7ede771-7c2b-4703-89c1-73f5336a23d9 (>= 13.1.99)", " 2ad69d6e-8bb6-4b2f-9d1c-7d148ced9a7f (>= 13.1.99)", " 43502725-a204-aa51-7023-e7bca149cac9 (>= 13.0.16)", " 36d12883-82a6-4be5-82dd-7fcbc50d2aef (>= 13.0.324)", " f8dde999-ce37-4251-9233-5eda85f0fa38 (>= 13.0.339)", " 686b8442-1f2d-4821-b40f-a1f5bd419bb8 (>= 13.0.340)", " 3db93f85-a052-4cc0-a7ca-bf8269170235 (>= 13.0.338)", " 690350a2-a200-4724-9cdb-ca5ba6bfff38 (>= 13.5.26)", " 784a62b0-6185-4e48-affb-0f4b0311f30f (>= 13.5.26)", " be400a3d-e9d6-48d9-af14-337722a11d40", " 04df33ba-8339-4a40-b62c-f9b859206716 (>= 13.5.70)", " f8ddb933-6a5d-4518-aea1-f251411ed98a (>= 13.5.69)", " f546fd4f-adc2-4933-bc31-9cae6c1a8685 (>= 13.5.70)", " b235b862-6a92-4a04-a8b2-6d71f777de67 (>= 13.5.70)", " 24ce31e6-358e-4583-9171-339af97c4847 (>= 13.1.99)", " a661d981-0a3b-4081-a5b5-1faa03cfaf84 (>= 13.1.101)", " 42e818c6-2b08-4de7-bd91-b0fd704c119a (>= 13.1.98)", " 562b2def-90a0-44a4-b79c-580b98833817 (>= 13.1.8)", " 3b7f3be4-8b26-4920-872e-b63cf714aaca (>= 13.1.99)", " d7aa8e34-ae59-45eb-acb9-3573dbf88dc9 (>= 2.0.77)", " 883e8a94-1250-442b-bb63-464792c2ed3c (>= 9.0.143)", " 82cae047-05b9-47ab-9c11-60dc11943f9d (>= 2.0.27)", " 47022337-36f3-4ac7-9021-e190df115288 (>= 5.60.30)", " d5004764-029c-4be1-828d-c8bc7b2f96a1 (>= 5.60.28)", " fda3f8bb-baa9-45d7-8dc7-22e1f5c76315 (>= 9.0.401)", " ba13bc17-0a77-40fb-8066-58b4266b153c (>= 4.01.49152)", " 7fb990c5-1a51-4c1d-99c4-c6e50368e105 (>= 3.11.190)", " 63b2a505-eba1-4284-af46-7c458073ab41 (>= 9.0.107)", " a9c3aed6-ae46-47ae-88e4-7aaeecf71a73 (>= 9.0.172)", " 80d3d303-75b9-4607-9312-e5fc68e5bfd2 (>= 10.0.1434)", " 9477fd26-0006-480f-9585-16a4c4f3f743 (>= 12.0.0422)", " 5b0cb826-e499-4e6b-94f0-75b6327ed934", " be400a3d-e9d6-48d9-af14-337722a11d40", " 5b0cb826-e499-4e6b-94f0-75b6327ed934", " be400a3d-e9d6-48d9-af14-337722a11d40", " 5b0cb826-e499-4e6b-94f0-75b6327ed934", " be400a3d-e9d6-48d9-af14-337722a11d40", " 5b0cb826-e499-4e6b-94f0-75b6327ed934", " be400a3d-e9d6-48d9-af14-337722a11d40", " 5b0cb826-e499-4e6b-94f0-75b6327ed934", " be400a3d-e9d6-48d9-af14-337722a11d40", " 5b0cb826-e499-4e6b-94f0-75b6327ed934", " be400a3d-e9d6-48d9-af14-337722a11d40", " 5b0cb826-e499-4e6b-94f0-75b6327ed934", " be400a3d-e9d6-48d9-af14-337722a11d40"], "Recommends"=[], "Suggests"=[], "Conflicts"=[], "Provides"=["b1197a7f-b64c-45de-b22d-f77e71c77a25 (= 13.1.101)", " 5200154e-c313-4829-96aa-04adb772c374 (= 13.1.101)", " 57a06a9a-a158-4b43-983e-1d14874f7e89 (= 13.1.101)", " 34dc243e-8b33-47f3-aa66-4a4bb7213b8b (= 13.1.101)", " f9ec26b7-9632-41a9-9c0b-22c424a9eafe (= 13.1.101)", " ad216f72-9c5d-4502-9f65-bde194bcc552 (= 13.1.101)", " a7b668a7-cf75-49c4-8f26-0489a3843173 (= 13.1.101)", " 7ef255b7-8219-4130-8077-5baeb7972fca (= 13.1.101)", " 0b45c248-4c28-42fd-bc86-6669aaac31ae (= 13.1.101)"], "Replaces"=[], "Supplements"=[], "Enhances"=[], "Product"=FALSE, "User visible"=TRUE, "Installed size (KB)"=0, "Package filesize (bytes)"=0, "Architecture"="windows_all", "Agent"="wininst", "MD5Checksum"=""}}, {287, "package attributes"={"Package Name"="a5e522fc-df4c-4aa7-a7c0-08b696662aa8", "Display name"="NI Instrument I/O Assistant", "Version"="17.0.9", "Display version"="", "Synopsis"="This is required for NI software.", "Description"="", "Maintainer"="National Instruments", "Maintainer email address"="support@ni.com", "Category"="Other Software", "Homepage"="", "Release notes"="", "Depends"=["5b0cb826-e499-4e6b-94f0-75b6327ed934", " be400a3d-e9d6-48d9-af14-337722a11d40", " 125332d8-372f-406e-baf2-9a6f1f9f57b2 (>= 4.80.768)", " 883e8a94-1250-442b-bb63-464792c2ed3c (>= 17.00.49152)", " 249f796d-f8da-49ff-89c5-be2d582fc277 (>= 8.6.10603)", " 5d6378b2-b24d-4ad6-5da2-faefdb81a250 (>= 13.0.3)", " be400a3d-e9d6-48d9-af14-337722a11d40", " 5b0cb826-e499-4e6b-94f0-75b6327ed934", " be400a3d-e9d6-48d9-af14-337722a11d40", " 5b0cb826-e499-4e6b-94f0-75b6327ed934", " be400a3d-e9d6-48d9-af14-337722a11d40", " 5b0cb826-e499-4e6b-94f0-75b6327ed934", " be400a3d-e9d6-48d9-af14-337722a11d40", " 5b0cb826-e499-4e6b-94f0-75b6327ed934"], "Recommends"=[], "Suggests"=[], "Conflicts"=[], "Provides"=["a5e522fc-df4c-4aa7-a7c0-08b696662aa8 (= 17.0.9)"], "Replaces"=[], "Supplements"=[], "Enhances"=[], "Product"=FALSE, "User visible"=TRUE, "Installed size (KB)"=0, "Package filesize (bytes)"=0, "Architecture"="windows_all", "Agent"="wininst", "MD5Checksum"=""}}, {294, "package attributes"={"Package Name"="3f4af77b-da0f-4b38-ae9b-56be5ab6da16", "Display name"="NI LabVIEW 2017 SP1 (32-bit)", "Version"="17.1.55", "Display version"="", "Synopsis"="This is required for NI software.", "Description"="", "Maintainer"="National Instruments", "Maintainer email address"="support@ni.com", "Category"="LabVIEW", "Homepage"="", "Release notes"="", "Depends"=["5b0cb826-e499-4e6b-94f0-75b6327ed934", " be400a3d-e9d6-48d9-af14-337722a11d40", " 5b0cb826-e499-4e6b-94f0-75b6327ed934", " be400a3d-e9d6-48d9-af14-337722a11d40", " 5b0cb826-e499-4e6b-94f0-75b6327ed934", " be400a3d-e9d6-48d9-af14-337722a11d40", " 5b0cb826-e499-4e6b-94f0-75b6327ed934", " be400a3d-e9d6-48d9-af14-337722a11d40", " 5b0cb826-e499-4e6b-94f0-75b6327ed934", " be400a3d-e9d6-48d9-af14-337722a11d40", " 5b0cb826-e499-4e6b-94f0-75b6327ed934", " 81a7e53e-9524-41ce-90d3-7dd3d90b6c58 (>= 5.50.49152)", " 9ac94877-534e-480a-8770-90007dcdd5fb (>= 1.03.49152)", " 62b7f1f4-da37-4ac5-9927-bc2bb4f59a6b (>= 17.1.51)", " 1e832e4e-2e4c-440d-83cb-523c610ba673 (>= 17.1.51)", " 8f101784-9b55-4e67-92c8-0e845f12f3ab (>= 17.10.49152)", " 5f89de52-e2a5-4e59-968c-f8e36e4703ed (>= 17.0.9)", " 6119c43c-b47a-4f5d-bf64-977e510d0761 (>= 15.0.4)", " 57119033-3f01-4ec2-a13d-f68ac8a80c54 (>= 17.1.51)", " 699c1ac5-2cf2-4745-9674-b19536eba8a3 (>= 17.00.49152)", " ab3599b6-97d9-4fe7-9e0d-87528fd8e8a7 (>= 17.00.49152)", " be400a3d-e9d6-48d9-af14-337722a11d40", " 5e4a4ce3-4d06-11d4-8b22-006008c16337 (>= 5.90.49152)", " d1edc484-7b17-11d7-83ce-00c0f03ebebe (>= 17.0.06654)", " d41b7da9-c5a7-41b5-8420-4cd6c925ef58 (>= 17.00.49152)", " eb7a3c81-1c0f-4495-8ce5-0a427e4e6285 (>= 17.00.49152)", " 739a9903-3a5f-442f-b551-ae7e3c83a668 (>= 17.00.49152)", " a298c267-3ce7-4b95-9d8b-bcb6672bc7b9 (>= 2.70.346)", " 11d580a9-caa9-4fae-acce-008751a7ae9f (>= 17.00.49152)", " fa89e82f-c220-43ff-acc0-47aa84d2be86 (>= 17.1.51)", " f25b73d5-73ef-457c-a906-b97ee6aa9998 (>= 17.1.51)", " 66421a85-b860-4356-a4cf-227fc81e2b5e (>= 17.1.51)", " 5b0cb826-e499-4e6b-94f0-75b6327ed934", " 2b749e2a-f771-4d55-80b2-322d1343c96f (>= 17.1.51)", " ab9b6d50-242e-4a2e-ac74-71647f3238c8 (>= 17.1.52)", " 683fc7bb-3f45-4156-a835-6f33b768888b (>= 17.00.49152)", " e48165c3-1d98-4281-ba67-e90a94e3a7ea (>= 17.0.5)", " 36d12883-82a6-4be5-82dd-7fcbc50d2aef (>= 17.0.207)", " f8dde999-ce37-4251-9233-5eda85f0fa38 (>= 17.0.205)", " 686b8442-1f2d-4821-b40f-a1f5bd419bb8 (>= 17.0.205)", " 49570182-efa6-4b4e-9181-572ecd14b262 (>= 17.0.206)", " a0851bb9-ad72-42db-bce9-24a13e79af47 (>= 17.0.62)", " b387fb1d-d22f-4dbe-bb3d-b689323905d7 (>= 17.0.57)", " be400a3d-e9d6-48d9-af14-337722a11d40", " 04df33ba-8339-4a40-b62c-f9b859206716 (>= 16.0.148)", " f8ddb933-6a5d-4518-aea1-f251411ed98a (>= 17.00.49152)", " f546fd4f-adc2-4933-bc31-9cae6c1a8685 (>= 17.0.57)", " fcf64b73-b7d4-4971-8f11-24baf7cc3e6c (>= 17.0.59)", " b235b862-6a92-4a04-a8b2-6d71f777de67 (>= 17.00.49153)", " 7a80ea72-c69d-4740-afbf-326544b9462c (>= 17.1.48)", " 620dbae1-b159-4204-8186-0813c8a6434c (>= 17.10.49154)", " 42e818c6-2b08-4de7-bd91-b0fd704c119a (>= 17.00.49152)", " 562b2def-90a0-44a4-b79c-580b98833817 (>= 17.01.49152)", " d7aa8e34-ae59-45eb-acb9-3573dbf88dc9 (>= 2.20.49155)", " 883e8a94-1250-442b-bb63-464792c2ed3c (>= 17.00.49153)", " 82cae047-05b9-47ab-9c11-60dc11943f9d (>= 2.20.49155)", " 47022337-36f3-4ac7-9021-e190df115288 (>= 17.50.32778)", " df644b10-84f5-4898-8e72-5f6af0d91330 (>= 17.50.32778)", " fda3f8bb-baa9-45d7-8dc7-22e1f5c76315 (>= 9.10.49152)", " d42e7bae-6589-4570-b6a3-3e28889392e7 (>= 14.14.49153)", " ba13bc17-0a77-40fb-8066-58b4266b153c (>= 4.62.49152)", " 7fb990c5-1a51-4c1d-99c4-c6e50368e105 (>= 17.50.49153)", " c3f9801f-8582-223e-e7ad-491795eeb8a6 (>= 17.1.3)", " fda19990-a725-4c6a-826c-a4f248917c7a (>= 17.00.49153)", " 0d590f8e-bfa2-49c8-b568-5a2d4001698c (>= 17.00.49153)", " 2ba6dd5e-d6eb-40ee-b781-3e61615e434a (>= 17.00.49152)", " 80d3d303-75b9-4607-9312-e5fc68e5bfd2 (>= 17.00.49157)", " ffd34a4d-6f7f-484b-a7c2-e34a427a27b6 (>= 15.00.49153)", " 5b0cb826-e499-4e6b-94f0-75b6327ed934", " be400a3d-e9d6-48d9-af14-337722a11d40", " 5b0cb826-e499-4e6b-94f0-75b6327ed934", " be400a3d-e9d6-48d9-af14-337722a11d40", " 5b0cb826-e499-4e6b-94f0-75b6327ed934", " be400a3d-e9d6-48d9-af14-337722a11d40", " 5b0cb826-e499-4e6b-94f0-75b6327ed934", " be400a3d-e9d6-48d9-af14-337722a11d40"], "Recommends"=[], "Suggests"=[], "Conflicts"=[], "Provides"=["c7846bae-e048-4342-8645-8d9b10d8b68f (= 17.1.55)", " dc669ffb-aa39-4fe5-af97-323288b1337e (= 17.1.55)", " 7804f495-62d3-43ab-b757-c77f9c798350 (= 17.1.55)", " 811c31ea-6ba5-4397-b4b5-acaacb053b0d (= 17.1.55)", " 9e2401b2-edb8-4faf-b0ff-d2801e3c9c60 (= 17.1.55)", " 3f4af77b-da0f-4b38-ae9b-56be5ab6da16 (= 17.1.55)", " 90dc7ac9-20f8-44ff-bbb7-db3c8ccd1e68 (= 17.1.263)", " e87a5b54-7589-4dce-bf76-032c21d97a3b (= 17.1.55)", " d6b0af80-1b82-4b87-94ea-219ade4eb883 (= 17.1.55)", " ee8caee7-07df-44f2-9584-5eeaaa2d0c4b (= 17.1.55)"], "Replaces"=[], "Supplements"=[], "Enhances"=[], "Product"=FALSE, "User visible"=TRUE, "Installed size (KB)"=0, "Package filesize (bytes)"=0, "Architecture"="windows_all", "Agent"="wininst", "MD5Checksum"=""}}, {297, "package attributes"={"Package Name"="aa333f93-319c-4ecc-8388-d40d5f7582f4", "Display name"="NI 1588-2008 Network Management Runtime 17.0.0", "Version"="17.0.26", "Display version"="", "Synopsis"="This is required for NI software.", "Description"="", "Maintainer"="National Instruments", "Maintainer email address"="support@ni.com", "Category"="Other Software", "Homepage"="", "Release notes"="", "Depends"=["5b0cb826-e499-4e6b-94f0-75b6327ed934", " be400a3d-e9d6-48d9-af14-337722a11d40", " 0e192465-cc28-4c84-be81-710b71c595a3 (>= 17.00.32772)", " 5b0cb826-e499-4e6b-94f0-75b6327ed934", " be400a3d-e9d6-48d9-af14-337722a11d40", " 0e192465-cc28-4c84-be81-710b71c595a3 (>= 17.00.32772)", " fda3f8bb-baa9-45d7-8dc7-22e1f5c76315 (>= 9.0.401)"], "Recommends"=[], "Suggests"=[], "Conflicts"=[], "Provides"=["aa333f93-319c-4ecc-8388-d40d5f7582f4 (= 17.0.26)", " 79fc6919-546a-4625-ae4c-a4e3db7d76ac (= 17.0.26)"], "Replaces"=[], "Supplements"=[], "Enhances"=[], "Product"=FALSE, "User visible"=TRUE, "Installed size (KB)"=0, "Package filesize (bytes)"=0, "Architecture"="windows_all", "Agent"="wininst", "MD5Checksum"=""}}, {299, "package attributes"={"Package Name"="6f882022-a36e-49bf-a815-f8142c16915f", "Display name"="NI LabVIEW 2017 Report Generation Toolkit for Microsoft Office", "Version"="17.0.166", "Display version"="", "Synopsis"="This is required for NI software.", "Description"="", "Maintainer"="National Instruments", "Maintainer email address"="support@ni.com", "Category"="LabVIEW", "Homepage"="", "Release notes"="", "Depends"=["5b0cb826-e499-4e6b-94f0-75b6327ed934", " be400a3d-e9d6-48d9-af14-337722a11d40", " 1f21a337-af6a-4451-b909-36a7874f26df (>= 17.0.174)"], "Recommends"=[], "Suggests"=[], "Conflicts"=[], "Provides"=["6f882022-a36e-49bf-a815-f8142c16915f (= 17.0.166)"], "Replaces"=[], "Supplements"=[], "Enhances"=[], "Product"=FALSE, "User visible"=TRUE, "Installed size (KB)"=0, "Package filesize (bytes)"=0, "Architecture"="windows_all", "Agent"="wininst", "MD5Checksum"=""}}, {303, "package attributes"={"Package Name"="d419ef00-27bb-48ea-936a-48466aec76ee", "Display name"="NI LabVIEW 2017 Database Connectivity Toolkit", "Version"="17.0.179", "Display version"="", "Synopsis"="This is required for NI software.", "Description"="", "Maintainer"="National Instruments", "Maintainer email address"="support@ni.com", "Category"="LabVIEW", "Homepage"="", "Release notes"="", "Depends"=["5b0cb826-e499-4e6b-94f0-75b6327ed934", " be400a3d-e9d6-48d9-af14-337722a11d40", " 86458082-85e4-47ff-a1f6-0c3ad40e6ffa (>= 17.0.180)"], "Recommends"=[], "Suggests"=[], "Conflicts"=[], "Provides"=["d419ef00-27bb-48ea-936a-48466aec76ee (= 17.0.179)"], "Replaces"=[], "Supplements"=[], "Enhances"=[], "Product"=FALSE, "User visible"=TRUE, "Installed size (KB)"=0, "Package filesize (bytes)"=0, "Architecture"="windows_all", "Agent"="wininst", "MD5Checksum"=""}}, {314, "package attributes"={"Package Name"="d9869122-d97c-42e4-8dfe-8e83b46698e6", "Display name"="NI LabWindows/CVI Side-By-Side Run-Time Engine 2013 SP2", "Version"="13.0.2278", "Display version"="", "Synopsis"="This is required for NI software.", "Description"="", "Maintainer"="National Instruments", "Maintainer email address"="support@ni.com", "Category"="Other Software", "Homepage"="", "Release notes"="", "Depends"=["be400a3d-e9d6-48d9-af14-337722a11d40 (>= 3.3.0)", " 5b0cb826-e499-4e6b-94f0-75b6327ed934 (>= 3.3.0)", " f222d8cd-bcab-4bcb-be60-767846d12a1b (>= 13.0)", " efba6f9e-f934-4bd7-ac51-60cca480489c (>= 10.0.100)", " bd1e864a-2acc-4f7e-9a7d-977c39952a52 (>= 9.0)", " 3109870c-c165-4896-ac99-afdd3ca3304a (>= 10.10)", " 5d6378b2-b24d-4ad6-5da2-faefdb81a250 (>= 13.0.0)", " 1038a887-23e1-4289-b0bd-0c4b83c6ba21 (>= 14.0.0)", " dd161794-1659-45e4-b2fd-53897e751e5b (>= 13.0)", " 63297dd3-02f1-4480-9f0c-b22d2f882749 (>= 13.0)", " d5cd591f-b8d5-4982-83e4-d19a33d85c4c (>= 13.0)", " 4eb6cbae-61a4-413d-a615-cc9012a73412 (>= 13.0)", " 20931852-6aa9-4918-926b-130d07a4cf8b (>= 13.0)", " 5b0cb826-e499-4e6b-94f0-75b6327ed934 (>= 3.3.0)", " be400a3d-e9d6-48d9-af14-337722a11d40 (>= 3.3.0)", " da6bbf6f-0910-4860-ad46-f14dadf645e9 (>= 14.00)", " fda3f8bb-baa9-45d7-8dc7-22e1f5c76315 (>= 9.0.401)"], "Recommends"=[], "Suggests"=[], "Conflicts"=[], "Provides"=["b10f5d52-1efa-435f-9404-c566d09e4875 (= 13.0.2278)", " d9869122-d97c-42e4-8dfe-8e83b46698e6 (= 13.0.2278)"], "Replaces"=[], "Supplements"=[], "Enhances"=[], "Product"=FALSE, "User visible"=TRUE, "Installed size (KB)"=0, "Package filesize (bytes)"=0, "Architecture"="windows_all", "Agent"="wininst", "MD5Checksum"=""}}, {326, "package attributes"={"Package Name"="ni-labview-2020-runtime-engine", "Display name"="LabVIEW Runtime (64-bit)", "Version"="20.1.1.49157-0+f5", "Display version"="2020 SP1 f1", "Synopsis"="The LabVIEW Runtime is a software add-on that enables engineers to run executables on a nondevelopment machine.", "Description"="The LabVIEW Runtime enables you to run executables created with the LabVIEW Application Builder on machines that do not have LabVIEW installed. The LabVIEW Runtime includes the libraries and other files necessary to run basic application types built in LabVIEW.", "Maintainer"="National Instruments", "Maintainer email address"="support@ni.com", "Category"="Programming Environments", "Homepage"="https://www.ni.com", "Release notes"="Refer to the NI website at https://www.ni.com/r/lv2020x1rm for installation instructions, known issues, bug fixes, compatibility information, and other important notices about this product.", "Depends"=["ni-activex-container (>= 17.1.2)", "ni-curl (>= 20.5.0)", "ni-deployment-framework-x86 (>= 20.0.0)", "ni-error-report (>= 20.1.0)", "ni-error-reporting-interface (>= 20.1.0)", "ni-labview-2020-realtime-nbfifo-x86 (>= 20.0.0)", "ni-logos (>= 20.0.0)", "ni-lv-web-server-labview-2020-runtime-engine-support (>= 20.5.1)", "ni-mdfsupport (>= 20.6.0)", "ni-mdnsresponder (>= 19.0.0)", "ni-metauninstaller (>= 20.6.0)", "ni-mkl-2017 (>= 17.0.1)", "ni-mkl-2020 (>= 20.0.0)", "ni-msiproperties (>= 20.6.0)", "ni-mstudio-cw3dgraph (>= 8.7.5)", "ni-msvcrt-2015 (>= 14.1.5)", "ni-python-interface (>= 20.0.0)", "ni-svcloc (>= 20.0.0)", "ni-systemlogging-utils (>= 20.0.0)", "ni-tdms (>= 19.0.0)", "ni-traceengine (>= 20.0.0)"], "Recommends"=[], "Suggests"=[], "Conflicts"=[], "Provides"=["580bec51-af79-4bf4-9227-4a78e80d2211 (= 20.11.49157)", "9a9fe130-6c4c-498b-a054-ceb195f36bb4 (= 20.11.49157)", "ni-labview-2020-runtime-engine (= 20.1.1.49157-0+f5)"], "Replaces"=[], "Supplements"=[], "Enhances"=[], "Product"=TRUE, "User visible"=TRUE, "Installed size (KB)"=0, "Package filesize (bytes)"=32106954, "Architecture"="windows_x64", "Agent"="wininst", "MD5Checksum"=""}}, {328, "package attributes"={"Package Name"="ni-package-manager", "Display name"="NI Package Manager", "Version"="24.3.0.49316-0+f164", "Display version"="2024 Q2", "Synopsis"="NI Package Manager facilitates the installation, removal, and management of NI software.", "Description"="", "Maintainer"="National Instruments", "Maintainer email address"="support@ni.com", "Category"="Utilities", "Homepage"="https://www.ni.com", "Release notes"="Refer to the NI website at https://www.ni.com/r/nipmrn for installation instructions, known issues, bug fixes, compatibility information, and other important notices about this product.", "Depends"=["ni-msdotnet4x (>= 23.8.0)", "ni-package-manager-upgrader", "ni-package-manager-deployment-support (>= 24.3.0.49316-0+f164)"], "Recommends"=[], "Suggests"=[], "Conflicts"=[], "Provides"=["ni-package-manager (= 24.3.0.49316-0+f164)"], "Replaces"=[], "Supplements"=[], "Enhances"=[], "Product"=TRUE, "User visible"=TRUE, "Installed size (KB)"=0, "Package filesize (bytes)"=19053996, "Architecture"="windows_x64", "Agent"="wininst", "MD5Checksum"="9720e4d5a9683f7cb1ece6f4a2ad272d"}}, {358, "package attributes"={"Package Name"="ni-labview-project-dependency-support", "Display name"="LabVIEW Project Dependency Support Software", "Version"="24.1.0.49312-0+f160", "Display version"="2024 Q1", "Synopsis"="Provides files required to identify dependencies for LabVIEW projects", "Description"="", "Maintainer"="National Instruments", "Maintainer email address"="support@ni.com", "Category"="Add-Ons", "Homepage"="https://www.ni.com", "Release notes"="Refer to the NI website at https://www.ni.com/r/labviewrn for installation instructions, known issues, bug fixes, compatibility information, and other important notices about this product.", "Depends"=["ni-mdfsupport (>= 24.0.0)", "ni-metauninstaller (>= 24.0.0)"], "Recommends"=[], "Suggests"=[], "Conflicts"=[], "Provides"=["ni-labview-project-dependency-support (= 24.1.0.49312-0+f160)"], "Replaces"=[], "Supplements"=[], "Enhances"=[], "Product"=TRUE, "User visible"=TRUE, "Installed size (KB)"=0, "Package filesize (bytes)"=444538, "Architecture"="windows_x64", "Agent"="wininst", "MD5Checksum"=""}}, {375, "package attributes"={"Package Name"="ni-dataplugins-aop5", "Display name"="ASAM e.V. DataPlugin for AOP5", "Version"="21.5.0.49290-0+f138", "Display version"="21.5.0", "Synopsis"="The ASAM Standards DataPlugin for AOP5 supports reading, writing, importing, and exporting of ASAM operational data store (ODS) data objects.", "Description"="", "Maintainer"="National Instruments", "Maintainer email address"="support@ni.com", "Category"="Add-Ons", "Homepage"="https://www.ni.com", "Release notes"="Refer to the NI website at https://www.ni.com/r/dp_aop5_doc for installation instructions, known issues, bug fixes, compatibility information, and other important notices about this product.", "Depends"=["ni-mdfsupport (>= 21.5.0)", "ni-metauninstaller (>= 21.5.0)", "ni-msvcrt-2015 (>= 14.1.5)"], "Recommends"=[], "Suggests"=[], "Conflicts"=["76c5a1fb-6d44-a455-703a-e98bbfcb69a1 (< 19.1.0)"], "Provides"=["76c5a1fb-6d44-a455-703a-e98bbfcb69a1 (= 21.50.49290)", "7d8169d2-eccc-49f5-9e79-4632c12673d0 (= 21.50.49290)", "ni-dataplugins-aop5 (= 21.5.0.49290-0+f138)"], "Replaces"=["76c5a1fb-6d44-a455-703a-e98bbfcb69a1 (< 19.1.0)"], "Supplements"=[], "Enhances"=[], "Product"=TRUE, "User visible"=TRUE, "Installed size (KB)"=0, "Package filesize (bytes)"=6416840, "Architecture"="windows_x64", "Agent"="wininst", "MD5Checksum"=""}}, {408, "package attributes"={"Package Name"="ni-datasocket", "Display name"="DataSocket", "Version"="24.1.0.49351-0+f199", "Display version"="2024 Q1.1", "Synopsis"="Support for built applications or shared libraries that use DataSocket. This installer includes the DataSocket Server, DataSocket Server Manager, and OPC Demo Server.", "Description"="", "Maintainer"="National Instruments", "Maintainer email address"="support@ni.com", "Category"="Runtime", "Homepage"="https://www.ni.com", "Release notes"="", "Depends"=["ni-logos (>= 24.1.0)", "ni-mdfsupport (>= 24.0.0)", "ni-metauninstaller (>= 24.0.0)", "ni-opcenum (>= 5.6.3)"], "Recommends"=[], "Suggests"=[], "Conflicts"=["81a7e53e-9524-41ce-90d3-7dd3d90b6c58 (< 5.50.0)"], "Provides"=["6d47a181-7ce8-4db2-92bc-521ff4bb5567 (= 24.10.49351)", "81a7e53e-9524-41ce-90d3-7dd3d90b6c58 (= 24.10.49351)", "ni-datasocket (= 24.1.0.49351-0+f199)"], "Replaces"=["81a7e53e-9524-41ce-90d3-7dd3d90b6c58 (< 5.50.0)"], "Supplements"=[], "Enhances"=[], "Product"=FALSE, "User visible"=TRUE, "Installed size (KB)"=0, "Package filesize (bytes)"=6574970, "Architecture"="windows_x64", "Agent"="wininst", "MD5Checksum"=""}}, {410, "package attributes"={"Package Name"="ni-variable-engine", "Display name"="Variable Engine", "Version"="24.1.0.49354-0+f202", "Display version"="2024 Q1.1", "Synopsis"="NI Variable Engine supports applications that read and write live data using shared variables. You must install this engine if you host, configure, or create shared variables in your application.", "Description"="", "Maintainer"="National Instruments", "Maintainer email address"="support@ni.com", "Category"="Runtime", "Homepage"="https://www.ni.com", "Release notes"="", "Depends"=["ni-logos (>= 24.1.0)", "ni-mdfsupport (>= 24.0.0)", "ni-metauninstaller (>= 24.0.0)", "ni-mxs (>= 24.0.0)", "ni-opc-support (>= 24.1.0)"], "Recommends"=[], "Suggests"=[], "Conflicts"=["eb7a3c81-1c0f-4495-8ce5-0a427e4e6285 (< 16.0.16384)"], "Provides"=["55805794-fdd9-4e71-8ad8-9896517f98c8 (= 24.10.49354)", "eb7a3c81-1c0f-4495-8ce5-0a427e4e6285 (= 24.10.49354)", "ni-variable-engine (= 24.1.0.49354-0+f202)"], "Replaces"=["eb7a3c81-1c0f-4495-8ce5-0a427e4e6285 (< 16.0.16384)"], "Supplements"=[], "Enhances"=[], "Product"=FALSE, "User visible"=TRUE, "Installed size (KB)"=0, "Package filesize (bytes)"=4294538, "Architecture"="windows_x64", "Agent"="wininst", "MD5Checksum"=""}}, {420, "package attributes"={"Package Name"="ni-labview-2023-runtime-engine-x86", "Display name"="LabVIEW Runtime (32-bit)", "Version"="23.3.0.49272-0+f120", "Display version"="2023 Q3", "Synopsis"="The LabVIEW Runtime is a software add-on that enables engineers to run executables on a nondevelopment machine.", "Description"="The LabVIEW Runtime enables you to run executables created with the LabVIEW Application Builder on machines that do not have LabVIEW installed. The LabVIEW Runtime includes the libraries and other files necessary to run basic application types built in LabVIEW.", "Maintainer"="National Instruments", "Maintainer email address"="support@ni.com", "Category"="Programming Environments", "Homepage"="https://www.ni.com", "Release notes"="Refer to the NI website at https://www.ni.com/r/labviewrn for installation instructions, known issues, bug fixes, compatibility information, and other important notices about this product.", "Depends"=["ni-activex-container (>= 17.1.2)", "ni-curl (>= 23.5.0)", "ni-deployment-framework-x86 (>= 23.3.0)", "ni-error-report-x86 (>= 20.1.0)", "ni-error-reporting-interface (>= 20.1.0)", "ni-labview-2023-realtime-nbfifo-x86 (>= 23.1.0)", "ni-labview-2023-runtime-engine-resource (>= 23.3.0)", "ni-logos (>= 23.3.0)", "ni-lv-web-server-labview-2023-runtime-engine-x86-support (>= 23.3.0)", "ni-matlab-interface (>= 23.3.0)", "ni-mdfsupport (>= 23.5.0)", "ni-mdnsresponder (>= 23.5.0)", "ni-metauninstaller (>= 23.5.0)", "ni-mkl-2017 (>= 17.0.1)", "ni-mkl-2020 (>= 20.0.0)", "ni-msiproperties (>= 23.5.0)", "ni-mstudio-cw3dgraph (>= 8.7.5)", "ni-msvcrt-2015 (>= 22.5.0)", "ni-python-interface (>= 23.3.0)", "ni-svcloc (>= 23.3.0)", "ni-systemlogging-utils (>= 20.0.0)", "ni-tdms (>= 23.3.0)", "ni-traceengine (>= 20.0.0)"], "Recommends"=[], "Suggests"=[], "Conflicts"=[], "Provides"=["4a9077c4-73d1-304e-be01-977ac35d2968 (= 23.30.49272)", "a3dd8cea-07bb-3eb5-a026-4ab75bdff807 (= 23.30.49272)", "ni-labview-runtime-engine-x86 (= 23.3.0)", "ni-labview-2023-runtime-engine-x86 (= 23.3.0.49272-0+f120)"], "Replaces"=[], "Supplements"=[], "Enhances"=[], "Product"=TRUE, "User visible"=TRUE, "Installed size (KB)"=0, "Package filesize (bytes)"=29259118, "Architecture"="windows_x64", "Agent"="wininst", "MD5Checksum"=""}}, {421, "package attributes"={"Package Name"="ni-labview-2023-runtime-engine", "Display name"="LabVIEW Runtime (64-bit)", "Version"="23.3.0.49272-0+f120", "Display version"="2023 Q3", "Synopsis"="The LabVIEW Runtime is a software add-on that enables engineers to run executables on a nondevelopment machine.", "Description"="The LabVIEW Runtime enables you to run executables created with the LabVIEW Application Builder on machines that do not have LabVIEW installed. The LabVIEW Runtime includes the libraries and other files necessary to run basic application types built in LabVIEW.", "Maintainer"="National Instruments", "Maintainer email address"="support@ni.com", "Category"="Programming Environments", "Homepage"="https://www.ni.com", "Release notes"="Refer to the NI website at https://www.ni.com/r/labviewrn for installation instructions, known issues, bug fixes, compatibility information, and other important notices about this product.", "Depends"=["ni-activex-container (>= 17.1.2)", "ni-curl (>= 23.5.0)", "ni-deployment-framework (>= 23.3.0)", "ni-error-report (>= 20.1.0)", "ni-error-reporting-interface (>= 20.1.0)", "ni-labview-2023-realtime-nbfifo (>= 23.1.0)", "ni-logos (>= 23.3.0)", "ni-lv-web-server-labview-2023-runtime-engine-support (>= 23.3.0)", "ni-matlab-interface (>= 23.3.0)", "ni-mdfsupport (>= 23.5.0)", "ni-mdnsresponder (>= 23.5.0)", "ni-metauninstaller (>= 23.5.0)", "ni-mkl-2017 (>= 17.0.1)", "ni-mkl-2020 (>= 20.0.0)", "ni-msiproperties (>= 23.5.0)", "ni-mstudio-cw3dgraph (>= 8.7.5)", "ni-msvcrt-2015 (>= 22.5.0)", "ni-python-interface (>= 23.3.0)", "ni-svcloc (>= 23.3.0)", "ni-systemlogging-utils (>= 20.0.0)", "ni-tdms (>= 23.3.0)", "ni-traceengine (>= 20.0.0)"], "Recommends"=[], "Suggests"=[], "Conflicts"=[], "Provides"=["95535c5e-6dcd-37f5-86dd-e68b5555a84d (= 23.30.49272)", "b5f88810-5fc9-3e79-b786-404c9235adc9 (= 23.30.49272)", "ni-labview-runtime-engine (= 23.3.0)", "ni-labview-2023-runtime-engine (= 23.3.0.49272-0+f120)"], "Replaces"=[], "Supplements"=[], "Enhances"=[], "Product"=TRUE, "User visible"=TRUE, "Installed size (KB)"=0, "Package filesize (bytes)"=34378290, "Architecture"="windows_x64", "Agent"="wininst", "MD5Checksum"=""}}, {422, "package attributes"={"Package Name"="ni-labview-2024-runtime-engine", "Display name"="LabVIEW Runtime (64-bit)", "Version"="24.1.0.49442-0+f290", "Display version"="2024 Q1", "Synopsis"="The LabVIEW Runtime is a software add-on that enables engineers to run executables on a nondevelopment machine.", "Description"="The LabVIEW Runtime enables you to run executables created with the LabVIEW Application Builder on machines that do not have LabVIEW installed. The LabVIEW Runtime includes the libraries and other files necessary to run basic application types built in LabVIEW.", "Maintainer"="National Instruments", "Maintainer email address"="support@ni.com", "Category"="Programming Environments", "Homepage"="https://www.ni.com", "Release notes"="Refer to the NI website at https://www.ni.com/r/labviewrn for installation instructions, known issues, bug fixes, compatibility information, and other important notices about this product.", "Depends"=["ni-activex-container (>= 17.1.2)", "ni-curl (>= 24.0.0)", "ni-deployment-framework (>= 24.1.0)", "ni-error-report (>= 20.1.0)", "ni-error-reporting-interface (>= 20.1.0)", "ni-labview-2024-realtime-nbfifo (>= 24.1.0)", "ni-logos (>= 24.1.0)", "ni-lv-web-server-labview-2024-runtime-engine-support (>= 24.1.0)", "ni-matlab-interface (>= 24.1.0)", "ni-mdfsupport (>= 24.0.0)", "ni-mdnsresponder (>= 24.0.0)", "ni-metauninstaller (>= 24.0.0)", "ni-mkl-2017 (>= 17.0.1)", "ni-mkl-2020 (>= 20.0.0)", "ni-msiproperties (>= 24.0.0)", "ni-mstudio-cw3dgraph (>= 8.7.5)", "ni-msvcrt-2015 (>= 22.5.0)", "ni-python-interface (>= 24.1.0)", "ni-svcloc (>= 24.1.0)", "ni-systemlogging-utils (>= 20.0.0)", "ni-tdms (>= 24.1.0)", "ni-traceengine (>= 20.0.0)"], "Recommends"=[], "Suggests"=[], "Conflicts"=[], "Provides"=["b2695a3e-34c2-3082-9b16-bb16f4df1a07 (= 24.10.49442)", "d5a1cc1a-cc93-31a0-b342-a12807d518ca (= 24.10.49442)", "ni-labview-runtime-engine (= 24.1.0)", "ni-labview-2024-runtime-engine (= 24.1.0.49442-0+f290)"], "Replaces"=[], "Supplements"=[], "Enhances"=[], "Product"=TRUE, "User visible"=TRUE, "Installed size (KB)"=0, "Package filesize (bytes)"=28272738, "Architecture"="windows_x64", "Agent"="wininst", "MD5Checksum"=""}}, {423, "package attributes"={"Package Name"="ni-labview-2024-runtime-engine-x86", "Display name"="LabVIEW Runtime (32-bit)", "Version"="24.1.1.49153-0+f1", "Display version"="2024 Q1 Patch 1", "Synopsis"="The LabVIEW Runtime is a software add-on that enables engineers to run executables on a nondevelopment machine.", "Description"="The LabVIEW Runtime enables you to run executables created with the LabVIEW Application Builder on machines that do not have LabVIEW installed. The LabVIEW Runtime includes the libraries and other files necessary to run basic application types built in LabVIEW.", "Maintainer"="National Instruments", "Maintainer email address"="support@ni.com", "Category"="Programming Environments", "Homepage"="https://www.ni.com", "Release notes"="Refer to the NI website at https://www.ni.com/r/labviewrn for installation instructions, known issues, bug fixes, compatibility information, and other important notices about this product.", "Depends"=["ni-activex-container (>= 17.1.2)", "ni-curl (>= 24.0.0)", "ni-deployment-framework-x86 (>= 24.1.0)", "ni-error-report-x86 (>= 20.1.0)", "ni-error-reporting-interface (>= 20.1.0)", "ni-labview-2024-realtime-nbfifo-x86 (>= 24.1.0)", "ni-labview-2024-runtime-engine-resource (>= 24.1.0)", "ni-logos (>= 24.1.0)", "ni-lv-web-server-labview-2024-runtime-engine-x86-support (>= 24.1.0)", "ni-matlab-interface (>= 24.1.0)", "ni-mdfsupport (>= 24.0.0)", "ni-mdnsresponder (>= 24.0.0)", "ni-metauninstaller (>= 24.0.0)", "ni-mkl-2017 (>= 17.0.1)", "ni-mkl-2020 (>= 20.0.0)", "ni-msiproperties (>= 24.0.0)", "ni-mstudio-cw3dgraph (>= 8.7.5)", "ni-msvcrt-2015 (>= 22.5.0)", "ni-python-interface (>= 24.1.0)", "ni-svcloc (>= 24.1.0)", "ni-systemlogging-utils (>= 20.0.0)", "ni-tdms (>= 24.1.0)", "ni-traceengine (>= 20.0.0)"], "Recommends"=[], "Suggests"=[], "Conflicts"=[], "Provides"=["5cf946e8-b758-3b92-867f-0e90e6a4c0eb (= 24.11.49153)", "b185da3f-07a4-3169-a5a5-4e748ac12a50 (= 24.11.49153)", "ni-labview-runtime-engine-x86 (= 24.1.1)", "ni-labview-2024-runtime-engine-x86 (= 24.1.1.49153-0+f1)"], "Replaces"=[], "Supplements"=[], "Enhances"=[], "Product"=TRUE, "User visible"=TRUE, "Installed size (KB)"=0, "Package filesize (bytes)"=24080322, "Architecture"="windows_x64", "Agent"="wininst", "MD5Checksum"=""}}, {424, "package attributes"={"Package Name"="ni-system-webserver", "Display name"="NI System Web Server 2024 Q1", "Version"="24.1.0.49346-0+f194", "Display version"="2024 Q1.1", "Synopsis"="Support for using Web services to communicate between National Instruments software, such as LabVIEW and NI Measurement & Automation Explorer.", "Description"="", "Maintainer"="National Instruments", "Maintainer email address"="support@ni.com", "Category"="Runtime", "Homepage"="https://www.ni.com", "Release notes"="", "Depends"=["ni-mdfsupport (>= 24.0.0)", "ni-metauninstaller (>= 24.0.0)", "ni-msiproperties (>= 24.0.0)", "ni-msvcrt-2015 (>= 22.5.0)", "ni-svcloc (>= 24.1.0)", "ni-system-webserver-appserver (>= 24.1.0)", "ni-system-webserver-base (>= 24.1.0)"], "Recommends"=[], "Suggests"=[], "Conflicts"=["fcf64b73-b7d4-4971-8f11-24baf7cc3e6c (< 17.9.9)"], "Provides"=["fcf64b73-b7d4-4971-8f11-24baf7cc3e6c (= 24.10.49346)", "ni-labview-web-server (= 24.10.49346)", "ni-system-webserver (= 24.1.0.49346-0+f194)"], "Replaces"=["fcf64b73-b7d4-4971-8f11-24baf7cc3e6c (< 17.9.9)"], "Supplements"=[], "Enhances"=[], "Product"=FALSE, "User visible"=TRUE, "Installed size (KB)"=0, "Package filesize (bytes)"=1962990, "Architecture"="windows_x64", "Agent"="wininst", "MD5Checksum"=""}}, {425, "package attributes"={"Package Name"="ni-syscfg-runtime", "Display name"="NI System Configuration Runtime", "Version"="24.0.0.49281-0+f129", "Display version"="2024 Q1", "Synopsis"="Run-time components required to deploy applications that use the NI System Configuration API.", "Description"="", "Maintainer"="National Instruments", "Maintainer email address"="support@ni.com", "Category"="Runtime", "Homepage"="https://www.ni.com", "Release notes"="", "Depends"=["ni-error-reporting-interface (>= 20.1.0)", "ni-mdfsupport (>= 24.0.0)", "ni-metauninstaller (>= 24.0.0)", "ni-msdotnet4x (>= 23.8.0)", "ni-msvcrt-2015 (>= 22.5.0)", "ni-networkdiscoverysvc (>= 24.0.0)", "ni-portable-configuration (>= 23.5.0)", "ni-remote-configuration (>= 24.0.0)", "ni-sysapi (>= 24.0.0)"], "Recommends"=[], "Suggests"=[], "Conflicts"=["0e192465-cc28-4c84-be81-710b71c595a3 (< 17.0.0)"], "Provides"=["0e192465-cc28-4c84-be81-710b71c595a3 (= 24.00.49281)", "ccd7729f-4b50-4e91-9a67-a3b1f932f350 (= 24.00.49281)", "ni-syscfg-runtime (= 24.0.0.49281-0+f129)"], "Replaces"=["0e192465-cc28-4c84-be81-710b71c595a3 (< 17.0.0)"], "Supplements"=[], "Enhances"=[], "Product"=FALSE, "User visible"=TRUE, "Installed size (KB)"=0, "Package filesize (bytes)"=4947172, "Architecture"="windows_x64", "Agent"="wininst", "MD5Checksum"=""}}, {427, "package attributes"={"Package Name"="ni-labview-datafinder-runtime", "Display name"="LabVIEW DataFinder Connectivity Runtime (64-bit)", "Version"="24.1.0.49442-0+f290", "Display version"="2024 Q1", "Synopsis"="LabVIEW DataFinder Connectivity Runtime enables the connection to DataFinder Server", "Description"="", "Maintainer"="National Instruments", "Maintainer email address"="support@ni.com", "Category"="Runtime", "Homepage"="https://www.ni.com", "Release notes"="", "Depends"=["ni-datafinder-client-api (>= 23.5.0)", "ni-dataplugins-aop5 (>= 21.5.0)", "ni-labview-2024-runtime-engine (>= 24.1.0)", "ni-mdfsupport (>= 24.0.0)", "ni-metauninstaller (>= 24.0.0)", "ni-msvcrt-2015 (>= 22.5.0)", "ni-usi-core (>= 21.5.0)"], "Recommends"=[], "Suggests"=[], "Conflicts"=[], "Provides"=["6b874e11-afa2-3c17-9a60-547be6539b93 (= 24.10.49442)", "ni-labview-datafinder-runtime (= 24.1.0.49442-0+f290)"], "Replaces"=[], "Supplements"=[], "Enhances"=[], "Product"=FALSE, "User visible"=TRUE, "Installed size (KB)"=0, "Package filesize (bytes)"=1604304, "Architecture"="windows_x64", "Agent"="wininst", "MD5Checksum"=""}}, {428, "package attributes"={"Package Name"="ni-labview-datafinder-runtime-x86", "Display name"="LabVIEW DataFinder Connectivity Runtime (32-bit)", "Version"="24.1.0.49448-0+f296", "Display version"="2024 Q1", "Synopsis"="LabVIEW DataFinder Connectivity Runtime enables the connection to DataFinder Server", "Description"="", "Maintainer"="National Instruments", "Maintainer email address"="support@ni.com", "Category"="Runtime", "Homepage"="https://www.ni.com", "Release notes"="Place Holder", "Depends"=["ni-datafinder-client-api (>= 23.5.0)", "ni-dataplugins-aop5 (>= 21.5.0)", "ni-labview-2024-runtime-engine-x86 (>= 24.1.0)", "ni-mdfsupport (>= 24.0.0)", "ni-metauninstaller (>= 24.0.0)", "ni-msvcrt-2015 (>= 22.5.0)", "ni-usi-core (>= 21.5.0)"], "Recommends"=[], "Suggests"=[], "Conflicts"=[], "Provides"=["ea4a692d-0dac-308f-88ed-dc875653b7e3 (= 24.10.49448)", "ni-labview-datafinder-runtime-x86 (= 24.1.0.49448-0+f296)"], "Replaces"=[], "Supplements"=[], "Enhances"=[], "Product"=FALSE, "User visible"=TRUE, "Installed size (KB)"=0, "Package filesize (bytes)"=1595422, "Architecture"="windows_x64", "Agent"="wininst", "MD5Checksum"=""}}, {429, "package attributes"={"Package Name"="ni-labview-command-line-interface-x86", "Display name"="NI LabVIEW Command Line Interface", "Version"="24.1.0.49355-0+f203", "Display version"="2024 Q1", "Synopsis"="The NI LabVIEW Command Line Interface (CLI) helps you run operations in LabVIEW by executing commands from the command line.", "Description"="The NI LabVIEW Command Line Interface (CLI) is a software add-on for LabVIEW. You can use it to automate the build process of LabVIEW applications and run the VIs and custom operations you create in LabVIEW.", "Maintainer"="National Instruments", "Maintainer email address"="support@ni.com", "Category"="Add-Ons", "Homepage"="https://www.ni.com", "Release notes"="Refer to the NI website at https://www.ni.com/r/labviewrn for installation instructions, known issues, bug fixes, compatibility information, and other important notices about this product.", "Depends"=["ni-labview-2024-runtime-engine-x86 (>= 24.1.0)", "ni-mdfsupport (>= 24.0.0)", "ni-metauninstaller (>= 24.0.0)"], "Recommends"=[], "Suggests"=[], "Conflicts"=["cf46d01c-2410-4cc1-affd-9ce404fedebe (< 1.0.0)"], "Provides"=["cf46d01c-2410-4cc1-affd-9ce404fedebe (= 24.10.49355)", "d27edd6f-752f-4478-a550-b7a34b7506ab (= 24.10.49355)", "ni-labview-command-line-interface-x86 (= 24.1.0.49355-0+f203)"], "Replaces"=["cf46d01c-2410-4cc1-affd-9ce404fedebe (< 1.0.0)"], "Supplements"=[], "Enhances"=[], "Product"=TRUE, "User visible"=TRUE, "Installed size (KB)"=0, "Package filesize (bytes)"=4419226, "Architecture"="windows_x64", "Agent"="wininst", "MD5Checksum"=""}}, {434, "package attributes"={"Package Name"="ni-syscfg-dotnet-runtime", "Display name"="NI System Configuration .NET Runtime", "Version"="23.8.0.49253-0+f101", "Display version"="2023 Q4", "Synopsis"="Enables you to run applications that use the NI System Configuration .NET API.", "Description"="", "Maintainer"="National Instruments", "Maintainer email address"="support@ni.com", "Category"="Runtime", "Homepage"="https://www.ni.com", "Release notes"="", "Depends"=["ni-mdfsupport (>= 23.8.0)", "ni-metauninstaller (>= 23.8.0)", "ni-syscfg-runtime (>= 23.8.0)"], "Recommends"=[], "Suggests"=[], "Conflicts"=["67b28cdf-779f-4203-89ff-094fa1fde46c (< 18.5.0)"], "Provides"=["67b28cdf-779f-4203-89ff-094fa1fde46c (= 23.80.49253)", "ni-syscfg-dotnet-runtime (= 23.8.0.49253-0+f101)"], "Replaces"=["67b28cdf-779f-4203-89ff-094fa1fde46c (< 18.5.0)"], "Supplements"=[], "Enhances"=[], "Product"=FALSE, "User visible"=TRUE, "Installed size (KB)"=0, "Package filesize (bytes)"=526894, "Architecture"="windows_x64", "Agent"="wininst", "MD5Checksum"=""}}, {442, "package attributes"={"Package Name"="ni-webserver", "Display name"="NI Web Server", "Version"="23.5.0.49152-0+f0", "Display version"="23.5.0", "Synopsis"="The NI Web Server hosts web applications and web UIs.", "Description"="", "Maintainer"="National Instruments", "Maintainer email address"="support@ni.com", "Category"="Utilities", "Homepage"="https://www.ni.com", "Release notes"="", "Depends"=["ni-ceip-x86 (>= 21.0.0)", "ni-mdfsupport (>= 21.0.0)", "ni-metauninstaller (>= 21.0.0)", "ni-msdotnet4x (>= 4.6.3)", "ni-msiproperties (>= 21.0.0)", "ni-msvcrt-2015 (>= 14.1.5)"], "Recommends"=[], "Suggests"=[], "Conflicts"=["8a12764f-2a58-45ad-a962-87d490209d58 (< 15.9.9)"], "Provides"=["8a12764f-2a58-45ad-a962-87d490209d58 (= 23.50.49152)", "ni-webserver (= 23.5.0.49152-0+f0)"], "Replaces"=["8a12764f-2a58-45ad-a962-87d490209d58 (< 15.9.9)"], "Supplements"=[], "Enhances"=[], "Product"=FALSE, "User visible"=TRUE, "Installed size (KB)"=0, "Package filesize (bytes)"=9725540, "Architecture"="windows_x64", "Agent"="wininst", "MD5Checksum"=""}}, {443, "package attributes"={"Package Name"="ni-license-manager", "Display name"="NI License Manager", "Version"="24.0.0.49245-0+f93", "Display version"="2024 Q1", "Synopsis"="NI License Manager is an application that helps you manage licensed NI software assets.", "Description"="NI License Manager is a tool designed to help you activate, deactivate, and transfer software products using license activation codes or license files. License administrators can use NI License Manager to automate product activation and add volume license servers.", "Maintainer"="National Instruments", "Maintainer email address"="support@ni.com", "Category"="Utilities", "Homepage"="https://www.ni.com", "Release notes"="Refer to the NI website at https://www.ni.com/r/nilmrn for installation instructions, known issues, bug fixes, compatibility information, and other important notices about this product.\n\nYou must have at least 1 GB of free space available to install this product.", "Depends"=["ni-ceip (>= 23.8.0)", "ni-ceip-x86 (>= 23.8.0)", "ni-license-manager-compatibility-server (>= 24.0.0)", "ni-mdfsupport (>= 24.0.0)", "ni-metauninstaller (>= 24.0.0)", "ni-msdotnet4x (>= 23.8.0)", "ni-msiproperties (>= 24.0.0)", "ni-msvcrt-2015 (>= 22.5.0)"], "Recommends"=[], "Suggests"=[], "Conflicts"=["cba7edb3-a142-43b6-b68b-a723624f1375 (< 4.0.0)"], "Provides"=["322ef433-71d5-4ca5-be56-ba7d280ac11c (= 24.00.49245)", "cba7edb3-a142-43b6-b68b-a723624f1375 (= 24.00.49245)", "ni-license-manager (= 24.0.0.49245-0+f93)"], "Replaces"=["cba7edb3-a142-43b6-b68b-a723624f1375 (< 4.0.0)"], "Supplements"=[], "Enhances"=[], "Product"=TRUE, "User visible"=TRUE, "Installed size (KB)"=0, "Package filesize (bytes)"=39408564, "Architecture"="windows_x64", "Agent"="wininst", "MD5Checksum"=""}}, {447, "package attributes"={"Package Name"="ni-max", "Display name"="NI Measurement & Automation Explorer", "Version"="23.8.0.49254-0+f102", "Display version"="2023 Q4", "Synopsis"="Use this application to configure, test, and communicate with your NI hardware.", "Description"="Use Measurement & Automation Explorer (MAX) to configure, test, and communicate with your NI hardware. You must install the appropriate driver software for your hardware to appear in MAX.", "Maintainer"="National Instruments", "Maintainer email address"="support@ni.com", "Category"="Utilities", "Homepage"="https://www.ni.com", "Release notes"="", "Depends"=["ni-ceip-x86 (>= 23.8.0)", "ni-error-report-x86 (>= 20.1.0)", "ni-error-reporting-interface (>= 20.1.0)", "ni-help-assistant (>= 2.2.0)", "ni-max-remote-provider (>= 23.8.0)", "ni-max-rempxi-provider (>= 23.8.0)", "ni-max-software-provider (>= 23.8.0)", "ni-mdfsupport (>= 23.8.0)", "ni-metauninstaller (>= 23.8.0)", "ni-msdotnet4x (>= 23.8.0)", "ni-msvcrt-2015 (>= 22.5.0)", "ni-mxs (>= 23.8.0)", "ni-portable-configuration (>= 23.5.0)", "ni-registration-wizard (>= 23.5.0)", "ni-resetniconfig (>= 23.8.0)", "ni-rpc (>= 23.8.0)", "ni-slcp-x86 (>= 23.8.0)", "ni-sysapi (>= 23.8.0)", "ni-syscfg-runtime (>= 23.8.0)", "ni-targetdiscoverywizard (>= 23.8.0)", "ni-webserver (>= 23.5.0)", "ni-xerces (>= 3.2.4)"], "Recommends"=["ni-hardware-configuration-importer (>= 8.4.0)"], "Suggests"=[], "Conflicts"=["ae940f24-cc0e-4148-9a96-10fb04d9796d (< 17.0.0)"], "Provides"=["ae940f24-cc0e-4148-9a96-10fb04d9796d (= 23.80.49254)", "dd8ce8fd-329b-49f9-a1c9-6235ae793e54 (= 23.80.49254)", "ni-max (= 23.8.0.49254-0+f102)"], "Replaces"=["ae940f24-cc0e-4148-9a96-10fb04d9796d (< 17.0.0)"], "Supplements"=[], "Enhances"=[], "Product"=FALSE, "User visible"=TRUE, "Installed size (KB)"=0, "Package filesize (bytes)"=5735830, "Architecture"="windows_x64", "Agent"="wininst", "MD5Checksum"=""}}, {460, "package attributes"={"Package Name"="ni-webservices-amqp-deployment-support-x86", "Display name"="NI Web Server Deployment Support for LabVIEW 2024 32-bit", "Version"="24.1.0.49345-0+f193", "Display version"="2024 Q1.1", "Synopsis"="Provides support for hosting Web services built in LabVIEW 2024 (32-bit) on NI Web Server.", "Description"="", "Maintainer"="National Instruments", "Maintainer email address"="support@ni.com", "Category"="Runtime", "Homepage"="https://www.ni.com", "Release notes"="", "Depends"=["ni-mdfsupport (>= 24.0.0)", "ni-metauninstaller (>= 24.0.0)", "ni-skyline-wif-webui (>= 24.0.0)", "ni-webserver-webservices-amqp (>= 23.5.1)"], "Recommends"=[], "Suggests"=[], "Conflicts"=["4b827355-0726-4dce-9d06-3e0341c537a4 (< 20.0.0)"], "Provides"=["4b827355-0726-4dce-9d06-3e0341c537a4 (= 24.10.49345)", "ni-webservices-amqp-deployment-support-x86 (= 24.1.0.49345-0+f193)"], "Replaces"=["4b827355-0726-4dce-9d06-3e0341c537a4 (< 20.0.0)"], "Supplements"=[], "Enhances"=[], "Product"=FALSE, "User visible"=TRUE, "Installed size (KB)"=0, "Package filesize (bytes)"=2342138, "Architecture"="windows_x64", "Agent"="wininst", "MD5Checksum"=""}}, {461, "package attributes"={"Package Name"="ni-certificates", "Display name"="NI Certificates Installer", "Version"="24.5.0.49157-0+f5", "Display version"="2024 Q3", "Synopsis"="NI Certificates configures Microsoft Windows to always trust software from NI. When NI Certificates are installed, no Windows security popups appear for installers that have a valid National Instruments digital signature.", "Description"="", "Maintainer"="National Instruments", "Maintainer email address"="support@ni.com", "Category"="Utilities", "Homepage"="https://www.ni.com", "Release notes"="", "Depends"=[], "Recommends"=[], "Suggests"=[], "Conflicts"=["1f2c1e66-64c0-4ce1-b96e-7bb6ec99fcb1 (< 1.99.0)"], "Provides"=["1f2c1e66-64c0-4ce1-b96e-7bb6ec99fcb1 (= 24.50.49157)", "ni-certificates (= 24.5.0.49157-0+f5)"], "Replaces"=["1f2c1e66-64c0-4ce1-b96e-7bb6ec99fcb1 (< 1.99.0)"], "Supplements"=[], "Enhances"=[], "Product"=FALSE, "User visible"=TRUE, "Installed size (KB)"=0, "Package filesize (bytes)"=463894, "Architecture"="windows_all", "Agent"="wininst", "MD5Checksum"=""}}, {462, "package attributes"={"Package Name"="ni-labview-2024-core-x86-en", "Display name"="LabVIEW (32-bit) English", "Version"="24.1.1.49153-0+f1", "Display version"="2024 Q1 Patch 1", "Synopsis"="LabVIEW is systems engineering software for applications that require test, measurement, and control with rapid access to hardware and data insights.", "Description"="The LabVIEW programming environment simplifies hardware integration for engineering applications so that you have a consistent way to acquire data from NI and third-party hardware. LabVIEW reduces the complexity of programming, so you can focus on your unique engineering problem. LabVIEW enables you to immediately visualize results with built-in, drag-and-drop engineering user interface creation and integrated data viewers. To turn your acquired data into real business results, you can develop algorithms for data analysis and advanced control with included math and signal processing IP or reuse your own libraries from a variety of tools. To ensure compatibility with other engineering tools, LabVIEW can interoperate with, and reuse libraries from, other software and open-source languages.", "Maintainer"="National Instruments", "Maintainer email address"="support@ni.com", "Category"="Programming Environments", "Homepage"="https://www.ni.com", "Release notes"="Refer to the NI website at https://www.ni.com/r/labviewrn for installation instructions, known issues, bug fixes, compatibility information, and other important notices about this product.", "Depends"=["ni-assistant-framework-labview-2024-codegen-x86-support (>= 24.1.0)", "ni-assistant-framework-x86 (>= 24.1.0)", "ni-ceip-x86 (>= 23.8.0)", "ni-codesignapi (>= 24.0.0)", "ni-curl (>= 24.0.0)", "ni-cvi-labview-dll-builder-15.1.0 (>= 15.1.1)", "ni-cvi-runtime-engine (>= 20.0.1)", "ni-daqmx-labview-shared-docs (>= 24.0.0)", "ni-datasocket (>= 24.1.0)", "ni-dfc-labview-support (>= 24.1.0)", "ni-error-report-x86 (>= 20.1.0)", "ni-example-finder-x86 (>= 24.1.0)", "ni-help-launcher (>= 24.0.0)", "ni-json-map (>= 24.1.0)", "ni-labview-2024-coreother-x86-en (>= 24.1.1)", "ni-labview-2024-deployable-license (>= 24.1.0)", "ni-labview-2024-example-x86-en (>= 24.1.0)", "ni-labview-2024-executable-x86 (>= 24.1.1)", "ni-labview-2024-help-x86-en (>= 24.1.0)", "ni-labview-2024-helpchm-en (>= 24.1.0)", "ni-labview-2024-license (>= 24.1.0)", "ni-labview-2024-manuals-x86-en (>= 24.1.0)", "ni-labview-2024-runtime-engine-x86 (>= 24.1.1)", "ni-labview-2024-scripting-codegen-x86 (>= 24.1.0)", "ni-labview-2024-simulation-x86-en (>= 24.1.0)", "ni-labview-2024-vilib-x86-en (>= 24.1.1)", "ni-labview-c-interface (>= 1.0.4)", "ni-labview-max-xml (>= 19.0.0)", "ni-labview-project-dependency-support (>= 24.1.0)", "ni-labview-vicompare-x86 (>= 24.1.0)", "ni-labview-vimerge-x86 (>= 24.1.0)", "ni-logos (>= 24.1.0)", "ni-logos-labview-2024-support-x86-en (>= 24.1.0)", "ni-mdfsupport (>= 24.0.0)", "ni-metauninstaller (>= 24.0.0)", "ni-mkl-2020 (>= 20.0.0)", "ni-msdotnet4x (>= 23.8.0)", "ni-msvcrt-2015 (>= 22.5.0)", "ni-mxs (>= 24.0.0)", "ni-opc-support (>= 24.1.0)", "ni-package-builder-labview-2024-support-x86-en (>= 24.1.0)", "ni-python-interface (>= 24.1.0)", "ni-search-labview-2024-support-x86 (>= 24.1.0)", "ni-slcp-x86 (>= 23.8.0)", "ni-ssl-labview-2024-x86-support (>= 24.1.0)", "ni-svcloc (>= 24.1.0)", "ni-system-webserver (>= 24.1.0)", "ni-system-webserver-appserver (>= 24.1.0)", "ni-systemlogging-utils (>= 20.0.0)", "ni-update-service (>= 21.0.0)", "ni-usi-core (>= 21.5.0)", "ni-variable-engine (>= 24.1.0)", "ni-variable-engine-labview-2024-support-x86-en (>= 24.1.0)", "ni-vipm-helper (>= 24.1.0)", "ni-web-based-configuration (>= 23.3.0)", "ni-web-pipeline-23.5 (>= 23.5.0)", "ni-web-services-labview-2024-x86-support (>= 24.1.0)"], "Recommends"=["mgi-solution-explorer (>= 2.5.5)", "ni-aspt-labview-support (>= 24.1.0)", "ni-certificates (>= 21.5.0)", "ni-dct-labview-support (>= 24.1.0)", "ni-dfdt-labview-support (>= 24.1.0)", "ni-distributed-system-manager-2024 (>= 24.1.0)", "ni-labview-command-line-interface-x86 (>= 24.1.0)", "ni-labview-dett (>= 24.1.0)", "ni-max (>= 23.8.0)", "ni-rgt-labview-support (>= 24.1.0)", "ni-syscfg-labview-support (>= 24.0.0)", "ni-tdm-excel-addin (>= 19.0.0)", "ni-utf-labview-support (>= 24.1.0)", "ni-viawin-labview-support (>= 24.1.0)", "ni-vipm (>= 24.1.0)", "ni-webservices-amqp-labview-2024-support-x86 (>= 24.1.0)"], "Suggests"=["jki-dragon (>= 2024.1.0)", "ni-labview-2024-ff-runtime-engine-x86 (>= 24.1.0)", "ni-wif (>= 20.5.1)"], "Conflicts"=["ni-labview-2024-x86-de (>= 0.0.0)", "ni-labview-2024-x86-fr (>= 0.0.0)", "ni-labview-2024-x86-ja (>= 0.0.0)", "ni-labview-2024-x86-ko (>= 0.0.0)", "ni-labview-2024-x86-zh-cn (>= 0.0.0)"], "Provides"=["0cbb534d-3dfd-365c-9aaa-3652599d4147 (= 24.11.49153)", "4529043c-1fc0-3029-887d-c30d66c7c372 (= 24.11.49153)", "ni-labview (= 24.1.1)", "ni-labview-2024-x86 (= 24.1.1)", "ni-labview-2024-x86-en", "ni-labview-x86 (= 24.1.1)", "ni-labview-2024-core-x86-en (= 24.1.1.49153-0+f1)"], "Replaces"=[], "Supplements"=[], "Enhances"=[], "Product"=TRUE, "User visible"=TRUE, "Installed size (KB)"=0, "Package filesize (bytes)"=3539278, "Architecture"="windows_x64", "Agent"="wininst", "MD5Checksum"=""}}, {463, "package attributes"={"Package Name"="ni-dfc-labview-support", "Display name"="NI LabVIEW DataFinder Connectivity VIs", "Version"="24.1.0.49448-0+f296", "Display version"="2024 Q1", "Synopsis"="LabVIEW DataFinder Connectivity Runtime enables the connection to DataFinder Server", "Description"="", "Maintainer"="National Instruments", "Maintainer email address"="support@ni.com", "Category"="Add-Ons", "Homepage"="https://www.ni.com", "Release notes"="Refer to the NI website at https://www.ni.com/r/lv2021rm for installation instructions, known issues, bug fixes, compatibility information, and other important notices about this product.", "Depends"=["ni-labview-datafinder-runtime (>= 24.1.0)", "ni-labview-datafinder-runtime-x86 (>= 24.1.0)", "ni-mdfsupport (>= 24.0.0)", "ni-metauninstaller (>= 24.0.0)", "ni-labview (>= 24.0.0)"], "Recommends"=[], "Suggests"=[], "Conflicts"=[], "Provides"=["ni-dfc-labview-support (= 24.1.0.49448-0+f296)"], "Replaces"=[], "Supplements"=["ni-labview (>= 24.0.0)"], "Enhances"=[], "Product"=TRUE, "User visible"=TRUE, "Installed size (KB)"=0, "Package filesize (bytes)"=1734080, "Architecture"="windows_x64", "Agent"="wininst", "MD5Checksum"=""}}, {464, "package attributes"={"Package Name"="ni-dct-labview-support", "Display name"="NI LabVIEW Database Connectivity Toolkit", "Version"="24.1.0.49444-0+f292", "Display version"="2024 Q1", "Synopsis"="The LabVIEW Database Connectivity Toolkit helps you connect to local and remote databases and implement common database operations.", "Description"="The LabVIEW Database Connectivity Toolkit is a software add-on for LabVIEW that helps you perform many database operations without using structured query language (SQL) programming. It readily connects to popular databases, such as Microsoft Access, SQL Server, and Oracle. If you need advanced database functionality and flexibility, the LabVIEW Database Connectivity Toolkit also offers complete SQL capabilities.", "Maintainer"="National Instruments", "Maintainer email address"="support@ni.com", "Category"="Add-Ons", "Homepage"="https://www.ni.com", "Release notes"="Refer to the NI website at https://www.ni.com/r/lvdctrn for installation instructions, known issues, bug fixes, compatibility information, and other important notices about this product.", "Depends"=["ni-labview-database-toolkit-lic (>= 24.1.0)", "ni-labview-database-toolkit-utility (>= 24.1.0)", "ni-mdfsupport (>= 24.0.0)", "ni-metauninstaller (>= 24.0.0)", "ni-labview (>= 24.0.0)"], "Recommends"=[], "Suggests"=[], "Conflicts"=[], "Provides"=["ni-dct-labview-support (= 24.1.0.49444-0+f292)"], "Replaces"=[], "Supplements"=["ni-labview (>= 24.0.0)"], "Enhances"=[], "Product"=TRUE, "User visible"=TRUE, "Installed size (KB)"=0, "Package filesize (bytes)"=3900380, "Architecture"="windows_x64", "Agent"="wininst", "MD5Checksum"=""}}, {465, "package attributes"={"Package Name"="ni-dett-labview-support", "Display name"="NI LabVIEW Desktop Execution Trace Toolkit", "Version"="24.1.0.49444-0+f292", "Display version"="2024 Q1", "Synopsis"="The LabVIEW Desktop Execution Trace Toolkit helps you perform dynamic code analysis for advanced debugging.", "Description"="The LabVIEW Desktop Execution Trace Toolkit helps you trace the execution of LabVIEW VIs on a Windows target during run time to detect and locate problems in code that could affect performance or cause unexpected behavior. It provides a chronological view of VI events, queue operations, reference leaks, memory allocation, unhandled errors, and subVI execution. With this toolkit, you can programmatically generate user-defined events from the block diagram of a LabVIEW application.", "Maintainer"="National Instruments", "Maintainer email address"="support@ni.com", "Category"="Add-Ons", "Homepage"="https://www.ni.com", "Release notes"="", "Depends"=["ni-mdfsupport (>= 24.0.0)", "ni-metauninstaller (>= 24.0.0)", "ni-labview (>= 24.0.0)"], "Recommends"=[], "Suggests"=[], "Conflicts"=[], "Provides"=["ni-dett-labview-support (= 24.1.0.49444-0+f292)"], "Replaces"=[], "Supplements"=["ni-labview (>= 24.0.0)"], "Enhances"=[], "Product"=FALSE, "User visible"=TRUE, "Installed size (KB)"=0, "Package filesize (bytes)"=1074712, "Architecture"="windows_x64", "Agent"="wininst", "MD5Checksum"=""}}, {466, "package attributes"={"Package Name"="ni-labview-dett", "Display name"="LabVIEW Desktop Execution Trace Toolkit", "Version"="24.1.0.49448-0+f296", "Display version"="2024 Q1", "Synopsis"="The LabVIEW Desktop Execution Trace Toolkit helps you perform dynamic code analysis for advanced debugging.", "Description"="The LabVIEW Desktop Execution Trace Toolkit helps you trace the execution of LabVIEW VIs on a Windows target during run time to detect and locate problems in code that could affect performance or cause unexpected behavior. It provides a chronological view of VI events, queue operations, reference leaks, memory allocation, unhandled errors, and subVI execution. With this toolkit, you can programmatically generate user-defined events from the block diagram of a LabVIEW application.", "Maintainer"="National Instruments", "Maintainer email address"="support@ni.com", "Category"="Add-Ons", "Homepage"="https://www.ni.com", "Release notes"="Refer to the NI website at https://www.ni.com/r/lvdettrn for installation instructions, known issues, bug fixes, compatibility information, and other important notices about this product.", "Depends"=["ni-labview-dett-core (>= 24.1.0)", "ni-mdfsupport (>= 24.0.0)", "ni-metauninstaller (>= 24.0.0)", "ni-update-service (>= 21.0.0)"], "Recommends"=["ni-dett-labview-support (>= 24.1.0)", "ni-labview-dett-labview-2021-support (>= 24.1.0)", "ni-labview-dett-labview-2021-support-x86 (>= 24.1.0)", "ni-labview-dett-labview-2022-support (>= 24.1.0)", "ni-labview-dett-labview-2022-support-x86 (>= 24.1.0)", "ni-labview-dett-labview-2023-support (>= 24.1.0)", "ni-labview-dett-labview-2023-support-x86 (>= 24.1.0)"], "Suggests"=[], "Conflicts"=["0fc217b4-710c-8871-ad88-9e092c9fa03c (< 19.0.0)"], "Provides"=["0fc217b4-710c-8871-ad88-9e092c9fa03c (= 24.10.49448)", "ni-labview-dett (= 24.1.0.49448-0+f296)"], "Replaces"=["0fc217b4-710c-8871-ad88-9e092c9fa03c (< 19.0.0)"], "Supplements"=[], "Enhances"=[], "Product"=TRUE, "User visible"=TRUE, "Installed size (KB)"=0, "Package filesize (bytes)"=604142, "Architecture"="windows_x64", "Agent"="wininst", "MD5Checksum"=""}}, {467, "package attributes"={"Package Name"="ni-rgt-labview-support", "Display name"="NI LabVIEW Report Generation Toolkit Support for LabVIEW", "Version"="24.1.0.49444-0+f292", "Display version"="2024 Q1", "Synopsis"="The LabVIEW Report Generation Toolkit provides VIs for programmatically creating and editing Microsoft Word and Excel reports from LabVIEW.", "Description"="The LabVIEW Report Generation Toolkit is a software add-on for LabVIEW that can generate reports on manufacturing test results or compile process statistics to improve your production yields. With this toolkit, you can easily populate report templates, email reports, execute macros, and manage report layout and appearance.", "Maintainer"="National Instruments", "Maintainer email address"="support@ni.com", "Category"="Add-Ons", "Homepage"="https://www.ni.com", "Release notes"="Refer to the NI website at https://www.ni.com/r/lvrgtrn for installation instructions, known issues, bug fixes, compatibility information, and other important notices about this product.", "Depends"=["ni-labview-report-generation-toolkit-lic (>= 24.1.0)", "ni-mdfsupport (>= 24.0.0)", "ni-metauninstaller (>= 24.0.0)", "ni-labview (>= 24.0.0)"], "Recommends"=[], "Suggests"=[], "Conflicts"=[], "Provides"=["ni-rgt-labview-support (= 24.1.0.49444-0+f292)"], "Replaces"=[], "Supplements"=["ni-labview (>= 24.0.0)"], "Enhances"=[], "Product"=TRUE, "User visible"=TRUE, "Installed size (KB)"=0, "Package filesize (bytes)"=4563382, "Architecture"="windows_x64", "Agent"="wininst", "MD5Checksum"=""}}, {469, "package attributes"={"Package Name"="ni-syscfg-labview-support", "Display name"="NI System Configuration Support for LabVIEW", "Version"="24.0.0.49281-0+f129", "Display version"="2024 Q1", "Synopsis"="Provides files required to create applications using the NI System Configuration API within LabVIEW.", "Description"="", "Maintainer"="National Instruments", "Maintainer email address"="support@ni.com", "Category"="Add-Ons", "Homepage"="https://www.ni.com", "Release notes"="", "Depends"=["ni-mdfsupport (>= 24.0.0)", "ni-metauninstaller (>= 24.0.0)", "ni-syscfg-labview-support-common (>= 24.0.0)", "ni-syscfg-runtime (>= 24.0.0)", "ni-labview (>= 22.0.0)"], "Recommends"=[], "Suggests"=[], "Conflicts"=[], "Provides"=["ni-syscfg-labview-support (= 24.0.0.49281-0+f129)"], "Replaces"=[], "Supplements"=["ni-labview (>= 22.0.0)"], "Enhances"=[], "Product"=FALSE, "User visible"=TRUE, "Installed size (KB)"=0, "Package filesize (bytes)"=11823896, "Architecture"="windows_x64", "Agent"="wininst", "MD5Checksum"=""}}, {470, "package attributes"={"Package Name"="ni-viawin-labview-support", "Display name"="NI LabVIEW VI Analyzer Toolkit Support for LabVIEW", "Version"="24.1.0.49444-0+f292", "Display version"="2024 Q1", "Synopsis"="The LabVIEW VI Analyzer Toolkit helps you perform static code analysis to improve the quality and readability of your LabVIEW code.", "Description"="The LabVIEW VI Analyzer Toolkit is a software add-on for LabVIEW that helps you improve graphical code developed in LabVIEW. With this toolkit, you can configure more than 90 included tests for automated code review and static code analysis of all VIs in an application, or you can create your own using the test creation wizard. The LabVIEW VI Analyzer Toolkit provides debugging tools that help you avoid improper coding techniques that could impact an application's performance, functionality, or maintainability. In addition, you can enforce effective programming practices and coding styles within teams of developers to ensure code readability and functionality.", "Maintainer"="National Instruments", "Maintainer email address"="support@ni.com", "Category"="Add-Ons", "Homepage"="https://www.ni.com", "Release notes"="Refer to the NI website at https://www.ni.com/r/lvviatrn for installation instructions, known issues, bug fixes, compatibility information, and other important notices about this product.", "Depends"=["ni-labview-vi-analyzer-toolkit-lic (>= 24.1.0)", "ni-mdfsupport (>= 24.0.0)", "ni-metauninstaller (>= 24.0.0)", "ni-labview (>= 24.0.0)"], "Recommends"=[], "Suggests"=[], "Conflicts"=[], "Provides"=["ni-viawin-labview-support (= 24.1.0.49444-0+f292)"], "Replaces"=[], "Supplements"=["ni-labview (>= 24.0.0)"], "Enhances"=[], "Product"=TRUE, "User visible"=TRUE, "Installed size (KB)"=0, "Package filesize (bytes)"=6868596, "Architecture"="windows_x64", "Agent"="wininst", "MD5Checksum"=""}}, {471, "package attributes"={"Package Name"="ni-webservices-amqp-labview-2024-support-x86", "Display name"="NI Web Server Development Support for LabVIEW 2024 32-bit", "Version"="24.1.0.49345-0+f193", "Display version"="2024 Q1.1", "Synopsis"="Provides support for developing Web services in LabVIEW 2024 (32-bit) hosted by NI Web Server.", "Description"="", "Maintainer"="National Instruments", "Maintainer email address"="support@ni.com", "Category"="Add-Ons", "Homepage"="https://www.ni.com", "Release notes"="", "Depends"=["ni-labview-2024-x86 (>= 24.0.0)", "ni-mdfsupport (>= 24.0.0)", "ni-metauninstaller (>= 24.0.0)", "ni-webservices-amqp-deployment-support-x86 (>= 24.1.0)"], "Recommends"=[], "Suggests"=[], "Conflicts"=[], "Provides"=["2be89605-ddca-39b9-9fce-bb464d9373e5 (= 24.10.49345)", "ni-webservices-amqp-labview-2024-support-x86 (= 24.1.0.49345-0+f193)"], "Replaces"=[], "Supplements"=["ni-labview-2024-x86 (>= 24.0.0)"], "Enhances"=[], "Product"=FALSE, "User visible"=TRUE, "Installed size (KB)"=0, "Package filesize (bytes)"=1042302, "Architecture"="windows_x64", "Agent"="wininst", "MD5Checksum"=""}}] ("Array")] -> w14
          frame Enabled {
            n8 = call <vilib>:"List Installed Packages.vi"() -> ("installed packages"=w19:string[][])  [unwired: 10 in, 1 out]
            n9 = Matrix Size(0:w19) -> (1:w20:i32)  [unwired: 1 out]
            n10 = for {
              tunnel: w19 -> [w29] mode=indexing
              tunnel: [w22] -> w18 mode=indexing if=w21
              tunnel: w20 -> [w28]
              i -> [w24]
              stop <- "System Stop Button" stop-if-true
              # "maintain original sort order"
              n11 = Decrement(x=w28) -> (x-1=w27:i32)
              n12 = Index Array(array=w29) -> (element #1=w31:string, element #2=w30:string)  [unwired: 2 in]
              n13 = Divide(x=w24, y=w27) -> (x/y=→"Package Info Progress":dbl)
              n14 = call <vilib>:"Get Package Attributes.vi"("version"=w30, "package name"=w31) -> ("package attributes"=w23:T1)  [unwired: 6 in, 3 out]
              n15 = Unbundle By Name(w23) -> ("User visible"=w21:bool)
              n16 = Bundle(w24, "package attributes"=w23) -> (w22:cluster{i32, "package attributes":T1})  [unwired: 1 in]
            }
          }
          frame Disabled {
            # "for testing - as takes a while to load"
          }
        }
        n17 = call "NIPKG Info to MCL Table.vi"("Array in"=w14) -> ("Array out"=w16:string[][])  [unwired: 10 in]
        n18 = property on="Installed NI Packages" class="MCListbox (strict)"("ItemNames"=w16, "Value"=w13) -> ()  [unwired: 2 in, 2 out]
        n19 = property on="Selected Packages" class="MCListbox (strict)"("ItemNames"=string[][] [] ("Item Names"), "Value"=w13) -> ()  [unwired: 2 in, 2 out]
      }
      event "Export": Value Change {
        # "Export selected package list to a JSON file"
        n20 = event-data() -> ()  [unwired: 1 in, 6 out]
        n21 = for {
          tunnel: w34 -> [w40] mode=indexing
          tunnel: [w39] -> w33 mode=indexing
          n22 = Unbundle(w40) -> ("package attributes"=w39:T1)  [unwired: 1 out]
        }
        n23 = call "To JSON Text.vim"("Anything"=w33) -> ("error out"=w35:errorcluster, "<JSON>"=w37:string)  [unwired: 9 in]
        n24 = Write to Text File(text=w37, error in=w35) -> (error out=w36:errorcluster)  [unwired: 2 in, 2 out]
        n25 = call <vilib>:"Simple Error Handler.vi"("error in (no error)"=w36) -> ()  [unwired: 4 in, 5 out]
      }
      event "Add": Value Change {
        w41 = i32[] [] ("Installed NI Packages")
        w46 = cluster{i32, "package attributes":T1}[] []
        # "Add selected packages to selected package list"
        n26 = event-data() -> ()  [unwired: 1 in, 1 out]
        n27 = local read "Installed NI Packages"() -> (w52:i32[])
        n28 = call-poly <userlib>:"Delete Elements from Array__ogtk.vi"("indices"=w52, "array"=w53) -> ("deleted elements"=w50:variant[], "array w/ subset deleted"=w51:variant[])  [unwired: 8 in]
        n29 = Variant To Data(type=w46, Variant=w51) -> (data=w43:cluster{i32, "package attributes":T1}[])  [unwired: 1 in, 1 out]
        n30 = Variant To Data(type=w46, Variant=w50) -> (data=w48:cluster{i32, "package attributes":T1}[])  [unwired: 1 in, 1 out]
        n31 = Build Array (concatenate)(w49, w48) -> (w47:cluster{i32, "package attributes":T1}[])
        n32 = Sort 1D Array(array=w47) -> (sorted array=w42:cluster{i32, "package attributes":T1}[])
        n33 = call "NIPKG Info to MCL Table.vi"("Array in"=w43) -> ("Array out"=w45:string[][])  [unwired: 10 in]
        n34 = call "NIPKG Info to MCL Table.vi"("Array in"=w42) -> ("Array out"=w44:string[][])  [unwired: 10 in]
        n35 = property on="Installed NI Packages" class="MCListbox (strict)"("ItemNames"=w45, "Value"=w41) -> ()  [unwired: 2 in, 2 out]
        n36 = property on="Selected Packages" class="MCListbox (strict)"("ItemNames"=w44, "Value"=w41) -> ()  [unwired: 2 in, 2 out]
      }
      event "Remove": Value Change {
        w54 = i32[] [] ("Installed NI Packages")
        w55 = cluster{i32, "package attributes":T1}[] []
        # "retain original sort order"
        # "Remove selected packages from selected package list (back to main list)"
        n37 = event-data() -> ()  [unwired: 1 in, 1 out]
        n38 = local read "Selected Packages"() -> (w64:i32[])
        n39 = call-poly <userlib>:"Delete Elements from Array__ogtk.vi"("indices"=w64, "array"=w63) -> ("deleted elements"=w65:variant[], "array w/ subset deleted"=w66:variant[])  [unwired: 8 in]
        n40 = Variant To Data(type=w55, Variant=w66) -> (data=w56:cluster{i32, "package attributes":T1}[])  [unwired: 1 in, 1 out]
        n41 = Variant To Data(type=w55, Variant=w65) -> (data=w61:cluster{i32, "package attributes":T1}[])  [unwired: 1 in, 1 out]
        n42 = Build Array (concatenate)(w60, w61) -> (w62:cluster{i32, "package attributes":T1}[])
        n43 = Sort 1D Array(array=w62) -> (sorted array=w57:cluster{i32, "package attributes":T1}[])
        n44 = call "NIPKG Info to MCL Table.vi"("Array in"=w57) -> ("Array out"=w59:string[][])  [unwired: 10 in]
        n45 = call "NIPKG Info to MCL Table.vi"("Array in"=w56) -> ("Array out"=w58:string[][])  [unwired: 10 in]
        n46 = property on="Installed NI Packages" class="MCListbox (strict)"("ItemNames"=w59, "Value"=w54) -> ()  [unwired: 2 in, 2 out]
        n47 = property on="Selected Packages" class="MCListbox (strict)"("ItemNames"=w58, "Value"=w54) -> ()  [unwired: 2 in, 2 out]
      }
    }
  }
  n48 = property on="System Refresh Button" class="Bool (strict)"("Val(Sgnl)"=FALSE ("Value (Signaling)")) -> ()  [unwired: 2 in, 2 out]
